vi "COD主界面（列队使用）.vi"() -> (8 "多列列表框":i32(listbox))   [LabVIEW 2016, in "斯坦道CODMn.lvlib"]
uses:
  <vilib>/Analysis/6fits.llb/Curve Fitting Criteria.ctl
  <vilib>/Utility/miscctls.llb/LVPointTypeDef.ctl
  <vilib>/Plasmionique/MB Master/MB_Master_Serial/MB_Master_Serial.lvclass
  D:/Program Files (x86)/National Instruments/LabVIEW 2016/vi.lib/Plasmionique/MB Master/MB_Master/MB_Master.lvclass
  <vilib>/Utility/config.llb/Write Key (Double).vi
  <vilib>/Utility/config.llb/Read Key (Double).vi
  <vilib>/Utility/config.llb/Read Key (Boolean).vi
  <vilib>/Utility/config.llb/Read Key (I32).vi
  <vilib>/Utility/config.llb/Write Key (Boolean).vi
  <vilib>/Utility/config.llb/Write Key (I32).vi
  <vilib>/Waveform/WDTFileIO.llb/Read Waveform from File.vi
  <vilib>/Plasmionique/MB Master/MB Master.lvlib
  <vilib>/ptbypt/NI_PtbyPt.lvlib
  <vilib>/Utility/config.llb/NI_LVConfig.lvlib
  <vilib>/Analysis/NI_AALPro.lvlib
panel:
  in  "一键写入":bool
  in  "测量模式(公式)":u16(ring)=1 items=["水样测试"=1, "标样核查"=2, "零点核查"=3, "跨度核查"=4, "空白测试"=5, "平行样"=6, "加标回收"=7]
  out "量程解释说明":string
  out "稀释倍数解释":string
  in  "低量程稀释倍数:":i8=1
  in  "高量程稀释倍数:":i8=2
  in  "测量模式":T1(ring)
  in  "高切低阈值":dbl
  in  "低切高阈值":dbl
  in  "数据查询":bool
  out "序列号:":string
  out "串口号:":refnum<visa-resource-name>
  in  "启用5":bool
  in  "校准5":bool
  in  "泵滴定数5":dbl
  in  "浓度5":dbl
  in  "启用4":bool
  in  "校准4":bool
  in  "泵滴定数4":dbl
  in  "浓度4":dbl
  out "波形时间":timestamp
  in  "历史波形":bool
  out "滴定数-ORP值":u16[](array[numeric]) caption="数组"
  in  "关闭 3":bool
  in  "滴定曲线":bool
  out "ORP滴定曲线2":u16[](graph)
  in  "跨度液浓度":dbl
  out "空白测试标记":bool
  out "跨度核查标记":bool
  out "启动选择 2":u16(ring) items=["水样测试", "标样核查", "零点核查", "跨度核查", "空白测试", "加标回收", "平行样", "校零", "校标"]
  in  "量程选择":enum16{"低量程", "高量程", "0-2量程"}(ring)
  in  "手动控制":bool
  in  "选用水样":enum16{"葡萄糖", "草酸钠"}(ring)
  in  "方程系数":cluster{"X":dbl, "b":dbl, "X^2":dbl} {"X^2" format="%#.4g"; "b" format="%#.4g"; "X" format="%#.4g"}
  out "多项式系数1":dbl[](array[numeric]) caption="多项式系数"
  out "XY图":cluster{"X Values":dbl[], "Y Values":dbl[]}[](graph)
  in  "模型":enum32{"线性", "多项式"}(ring)
  out "启动时间":timestamp format="%<%Y/%m/%d %H:%M:%S>T"
  in  "自动切换量程":bool=TRUE
  in  "24H周期设置":bool[](xcontrol)
  in  "关闭 2":bool
  in  "周期设置":bool
  out "r^2":dbl format="%.8g"
  out "拟合公式":string
  out "b":dbl format="%#.4g"
  out "K":dbl format="%#.4f"
  out "当前校准":i32
  in  "启用3":bool
  in  "启用2":bool
  in  "启用1":bool
  in  "校准3":bool
  in  "校准2":bool
  in  "校准1":bool
  in  "泵滴定数3":dbl
  in  "泵滴定数2":dbl
  in  "泵滴定数1":dbl
  in  "浓度3":dbl
  in  "浓度2":dbl
  in  "浓度1":dbl
  in  "写入":bool
  out "测量模式数字":i32
  out "零点核查标记":bool
  out "排液故障":bool
  out "进水样超量程":bool
  out "标样核查标记":bool
  out "平行样测量":bool
  out "加标回收测量":bool
  out "质控样测量":bool
  out "待机":bool
  out "校标错误":bool
  out "校零错误":bool
  out "测量错误":bool
  out "草酸钠报警":bool
  out "高锰酸钾报警":bool
  out "加热故障":bool
  out "温控器故障":bool
  out "ORP故障":bool
  out "排液标记":bool
  out "故障标记":bool
  out "校标标记":bool
  out "校零标记":bool
  out "通讯状态":bool
  out "水样测量":bool
  out "读取KB值":bool
  in  "读取":bool
  in  "返回":bool
  in  "校准配置":bool
  in  "修正系数 2":dbl
  in  "浓度 2":dbl
  in  "温度":dbl
  in  "恒温时间":dbl
  in  "基本量程":enum16{"L", "H"}(ring)
  in  "水样":dbl
  in  "蒸馏水":dbl
  in  "标液":dbl
  in  "质控样":dbl
  in  "加标回收":dbl
  in  "草酸钠":dbl
  in  "高锰酸钾":dbl
  in  "硫酸":dbl
  in  "零点泵计量数 2":dbl
  in  "标度泵计量数 2":dbl
  out "标度滴定值":dbl
  out "零点滴定值":dbl
  in  "保存":bool
  in  "关闭":bool
  out "测量数据区":T2 {"单位" items=["ug/L", "mg/L", "ppm", "mg/m3", "cm", "ppb", "ug/m3", "%", "nmol/mol", "umol/mol", "MPN/L", "MPN/100ml", "ng/m3", "NTU", "无量纲", "ms/cm", "us/cm", "℃", "mV", "万个/L"]}
  out "仪器时间":timestamp format="%<%Y/%m/%d %H:%M:%S>T"
  out "秒":u16
  out "分":u16
  out "COD浓度（mg/L)":dbl format="%.2g"
  out "进样管":dbl
  out "高锰酸钾":dbl
  out "草酸钠":dbl
  out "硫酸":dbl
  out "ORP显示":dbl
  out "温度":dbl
  out "加热":bool
  out "搅拌":bool
  out "进硫酸":bool
  out "进加标回收样":bool
  out "进质控样":bool
  out "进标液":bool
  out "进蒸馏水":bool
  out "进水样":bool
  out "进草酸钠":bool
  out "进高锰酸钾":bool
  out "定时启动":bool
  in  "启动":bool
  in  "故障清除":bool
  in  "参数配置":bool
  in  "停止":bool
  in  "单步启动":bool
  out "系统时间":timestamp
  in  "时间校准":bool
  in  "枚举":enum16{"读取数据", "写入数据", "读取写入DATABASE", "读取参数"}(ring)
  out "Registers":u16[](array[numeric])
  in  "Slave ID":u8=1
  in  "Serial Config":T3={"baud rate (bps)"=115200, "stop bits"=10, "parity"=0, "flow control"=0, "timeout"=1000, "retries"=1} {"stop bits" items=["1.0"=10, "1.5"=15, "2.0"=20]; "flow control" items=["None", "XON/XOFF", "RTS/CTS", "XON/XOFF & RTS/CTS", "DTR/DSR", "XON/XOFF & DTR/DSR"]; "parity" items=["None", "Odd", "Even", "Mark", "Space"]}
  in  "温度 2":dbl
  in  "浓度":dbl
  in  "修正系数":dbl
  in  "标样浓度 2":dbl
  out "模式（受控）":u16
  in  "VISA resource name":refnum<visa-resource-name>="COM4" caption="VISA资源名称"
  # "测量时间："
  # "水样~加标回收"
  # "mV"
  # "℃"
  # "注：遇到加热故障和排液故障时仪器不能正常启动，\n必须排查故障并点击报警清除按钮方可运行。"
  # "mg/L"
  # "基本参数设置"
  # "泵计量参数设置"
  # "校零校标结果"
  # "加热恒温温度（℃）："
  # "水样："
  # "高锰酸钾："
  # "校零结果："
  # "校零滴定值："
  # "恒温时间（分钟）："
  # "蒸馏水："
  # "草酸钠："
  # "校标结果："
  # "标度滴定值："
  # "标准液浓度（mg/L）："
  # "标液："
  # "硫酸："
  # "零点泵计量值："
  # "修正系数："
  # "标度泵计量值："
  # "质控样："
  # "跨度液浓度："
  # "标样浓度："
  # "基本量程（L、H可选）："
  # "加标回收样："
  # "（mg/L）"
  # "是否启用"
  # "泵滴定数"
  # "浓度"
  # "辅\n助\n计\n算\n区"
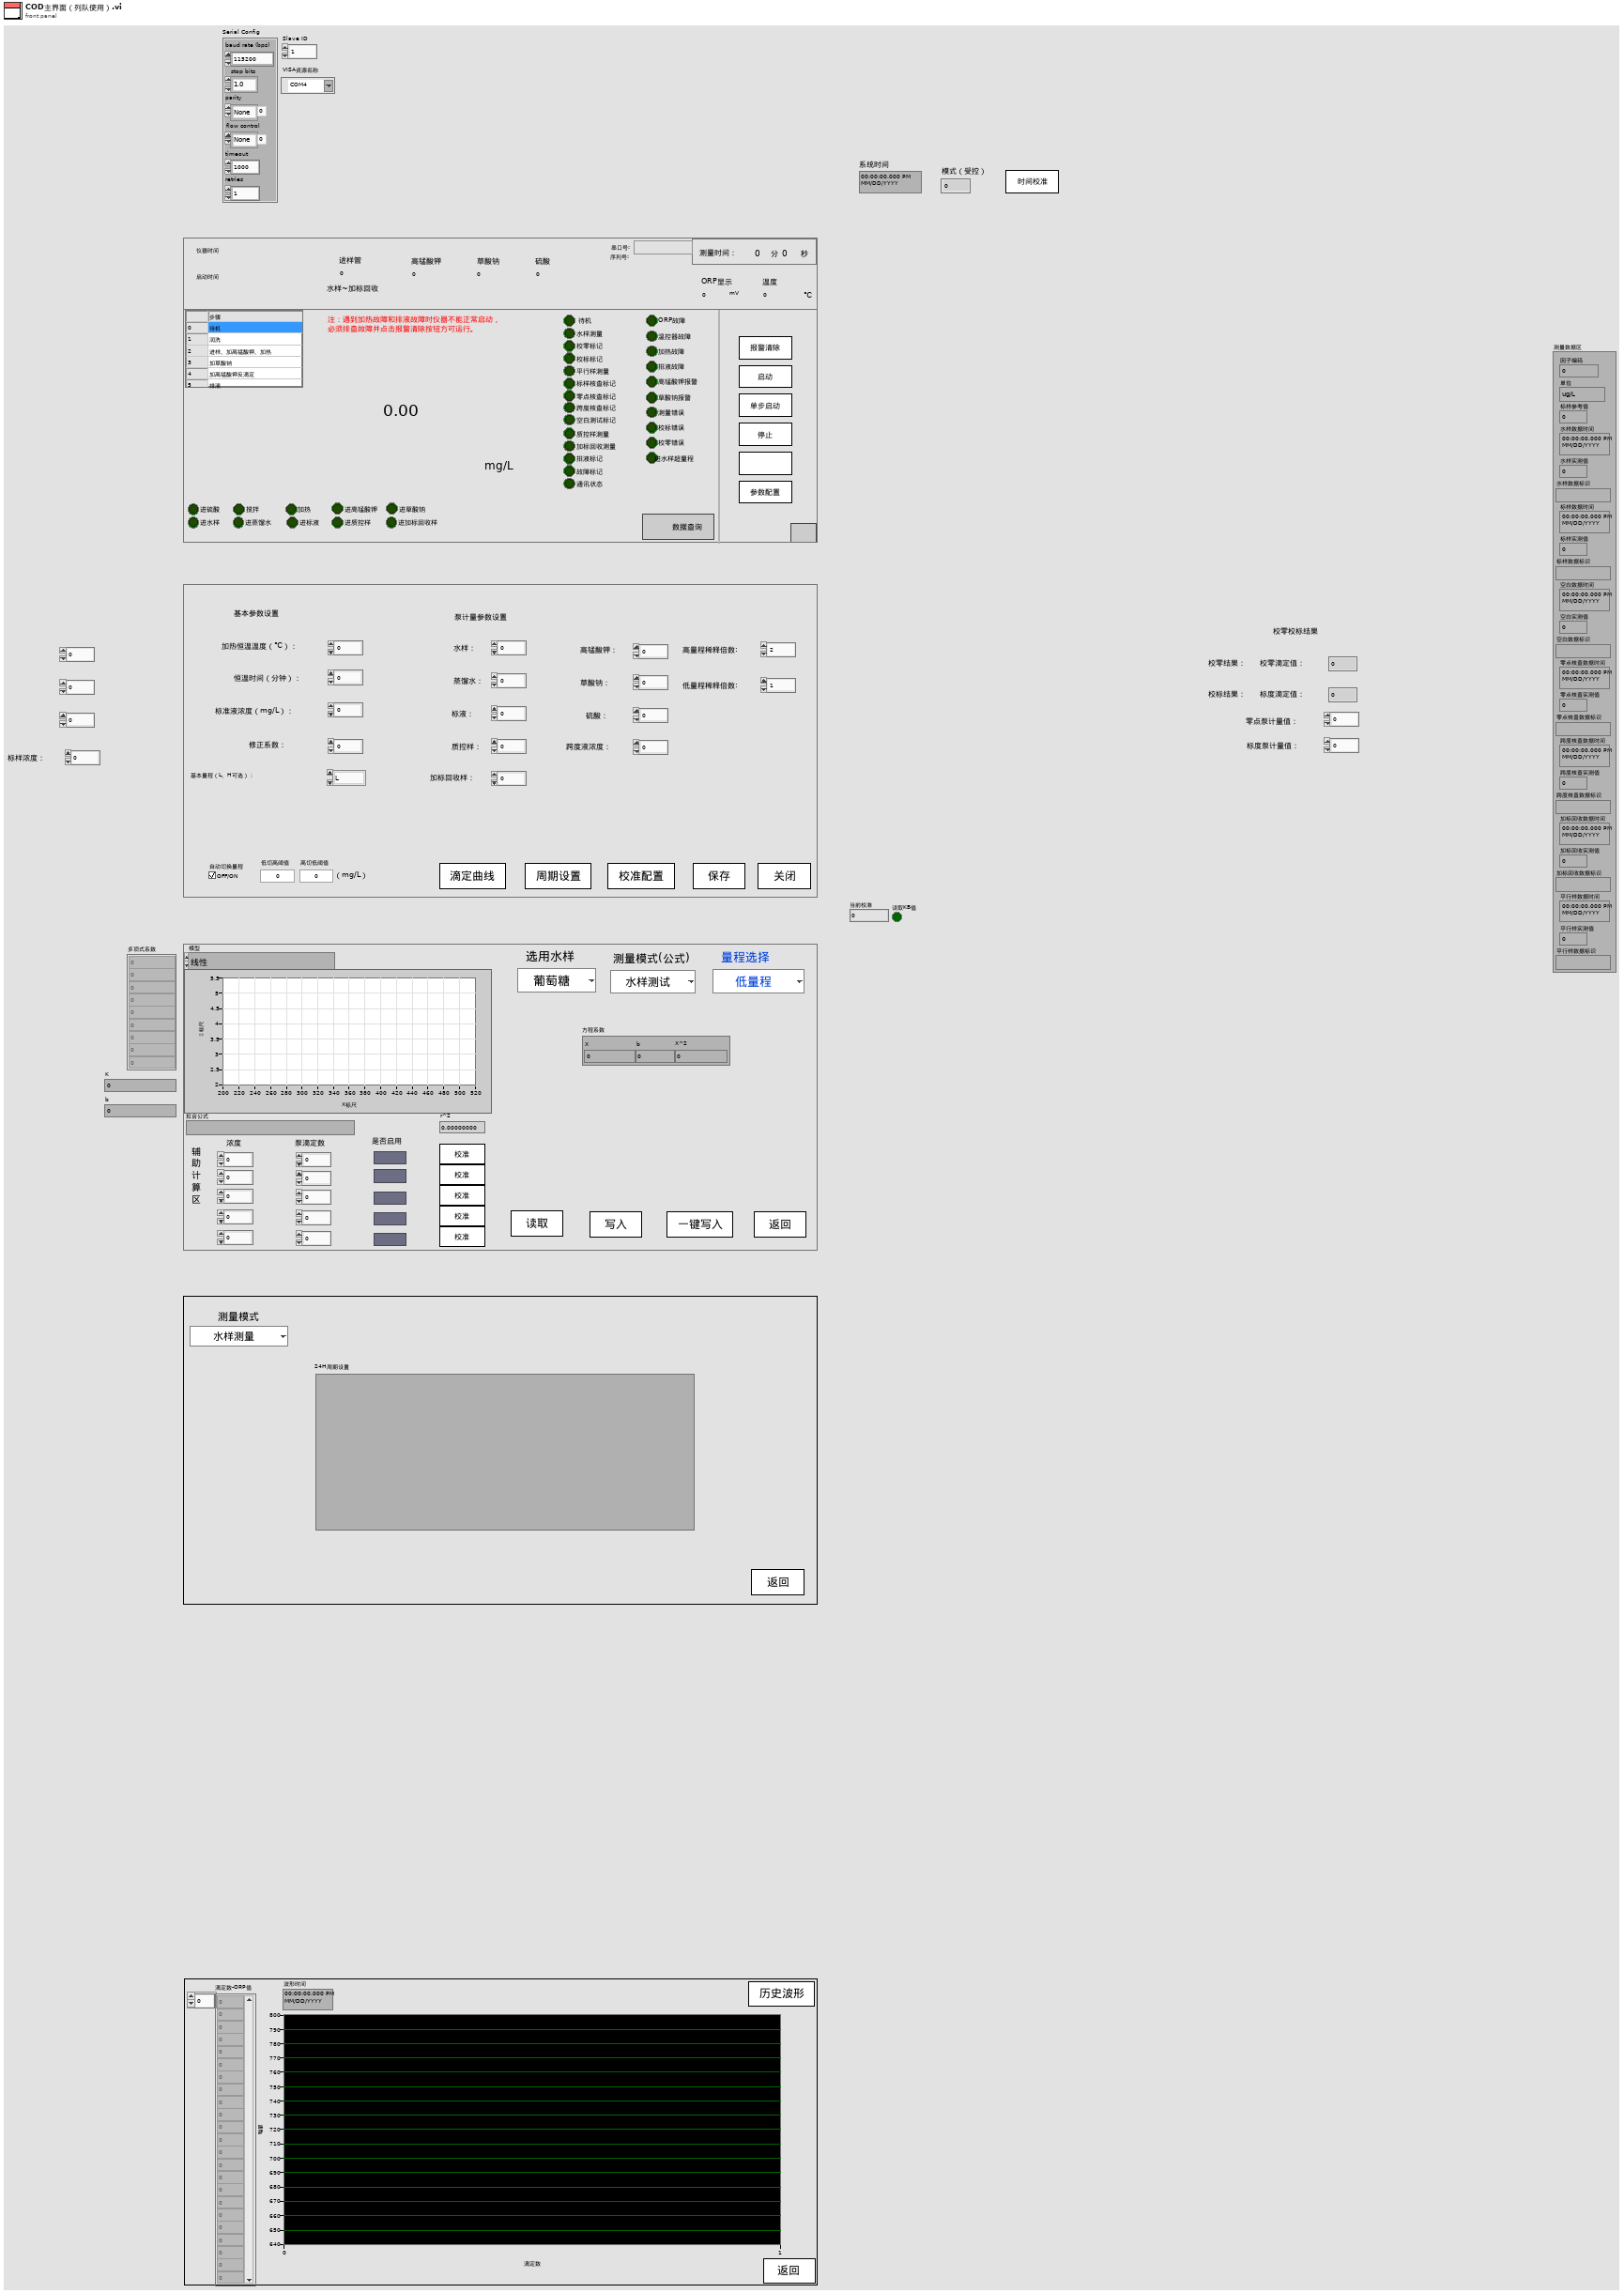
[diagram p1: front panel]
types:
  T1 = enum16{"水样测量", "标样核查", "零点核查", "跨度核查", "空白测试", "加标回收", "平行样", "校零", "校标"}
  T2 = cluster{"因子编码":u32, "单位":u16, "标样参考值":sgl, "水样数据时间":timestamp, "水样实测值":sgl, "水样数据标识":string, "标样数据时间":timestamp, "标样实测值":sgl, "标样数据标识":string, "空白数据时间":timestamp, "空白实测值":sgl, "空白数据标识":string, "零点核查数据时间":timestamp, "零点核查实测值":sgl, "零点核查数据标识":string, "跨度核查数据时间":timestamp, "跨度核查实测值":sgl, "跨度核查数据标识":string, "加标回收数据时间":timestamp, "加标回收实测值":sgl, "加标回收数据标识":string, "平行样数据时间":timestamp, "平行样实测值":sgl, "平行样数据标识":string}
  T3 = cluster{"baud rate (bps)":u32, "stop bits":u16, "parity":u16, "flow control":u16, "timeout":u32, "retries":i32}
  T4 = cluster{"starting address":u16, "number of holding registers":u16}
  T5 = cluster{"测量模式":enum16{"水样测量", "标样核查", "零点核查", "跨度核查", "空白测试", "加标回收", "平行样", "校零", "校标"}}
  T6 = cluster{"仪器测试类型":enum16{"水样测试", "标样核查", "空白测试", "跨度核查"}, "周期设置类型":enum16{"定点启动", "间隔启动"}, "定时功能启用":bool, "定时间隔":dbl, "24H周期设置":bool[]}
  T7 = typedef "LVDateTimeRec.ctl" = cluster{"秒数的小数部分":dbl, "秒":i32, "分":i32, "时":i32, "日":i32, "月":i32, "年":i32, "天数（周）":i32, "天数（年）":i32, "DST":i32}
  T8 = typedef "imagedata.ctl" = cluster{"image type":i32, "image depth":i32, "image":u8[], "mask":u8[], "colors":u32[], "Rectangle":cluster{"left":i16, "top":i16, "right":i16, "bottom":i16}}
  T9 = typedef "NI_LVConfig.lvlib/Config Data RefNum.ctl" = refnum<k1>
  T10 = typedef "LVPointTypeDef.ctl" = cluster{"Horizontal":i16, "Vertical":i16}
  T11 = enum8{"Enabled", "Disabled", "Disabled and Grayed Out"}
  T12 = cluster{"ORP故障":bool, "温控器故障":bool, "加热故障":bool, "高锰酸钾报警":bool, "草酸钠报警":bool, "测量错误":bool, "校零错误":bool, "校标错误":bool, " 进水样超量程":bool, "排液阀故障":bool}
  T13 = cluster{"时间标识":timestamp, "参数":string, "日志信息":string, "流程参数":string}
  T14 = cluster{"时间标识":timestamp, "设备":string, "日志信息":string}
  T15 = typedef "NI_AALPro.lvlib/Curve Fitting Criteria.ctl" = u16
  T16 = cluster{"时间标识":timestamp, "设备":string, "日志信息":string, "流程参数":string}
  T17 = cluster{"时间":timestamp, "测量模式":string, "数据类型":string, "检测值":sgl, "单位":string, "数据标识":string, "因子编码":string, "标样参考值":sgl, "ORP-A":sgl, "ORP-B":sgl, "ORP-K":sgl, "COD滴定值":sgl, "高锰酸钾滴定数":sgl, "温度":sgl, "序列号":string}
  T18 = cluster{"数组 2[0]":sgl, "数组 2[1]":sgl, "数组 2[2]":sgl, "数组 2[3]":sgl, "数组 2[4]":sgl, "数组 2[5]":sgl, "数组 2[6]":sgl, "数组 2[7]":sgl, "数组 2[8]":sgl, "数组 2[9]":sgl, "数组 2[10]":sgl, "数组 2[11]":sgl, "数组 2[12]":sgl, "数组 2[13]":sgl, "数组 2[14]":sgl, "数组 2[15]":sgl, "数组 2[16]":sgl, "数组 2[17]":sgl, "数组 2[18]":sgl, "数组 2[19]":sgl, "数组 2[20]":sgl, "数组 2[21]":sgl, "数组 2[22]":sgl, "数组 2[23]":sgl, "数组 2[24]":sgl, "数组 2[25]":sgl, "数组 2[26]":sgl, "数组 2[27]":sgl, "数组 2[28]":sgl, "数组 2[29]":sgl, "数组 2[30]":sgl, "数组 2[31]":sgl, "数组 2[32]":sgl, "数组 2[33]":sgl, "数组 2[34]":sgl, "数组 2[35]":sgl, "数组 2[36]":sgl, "数组 2[37]":sgl, "数组 2[38]":sgl, "数组 2[39]":sgl, "数组 2[40]":sgl, "数组 2[41]":sgl}
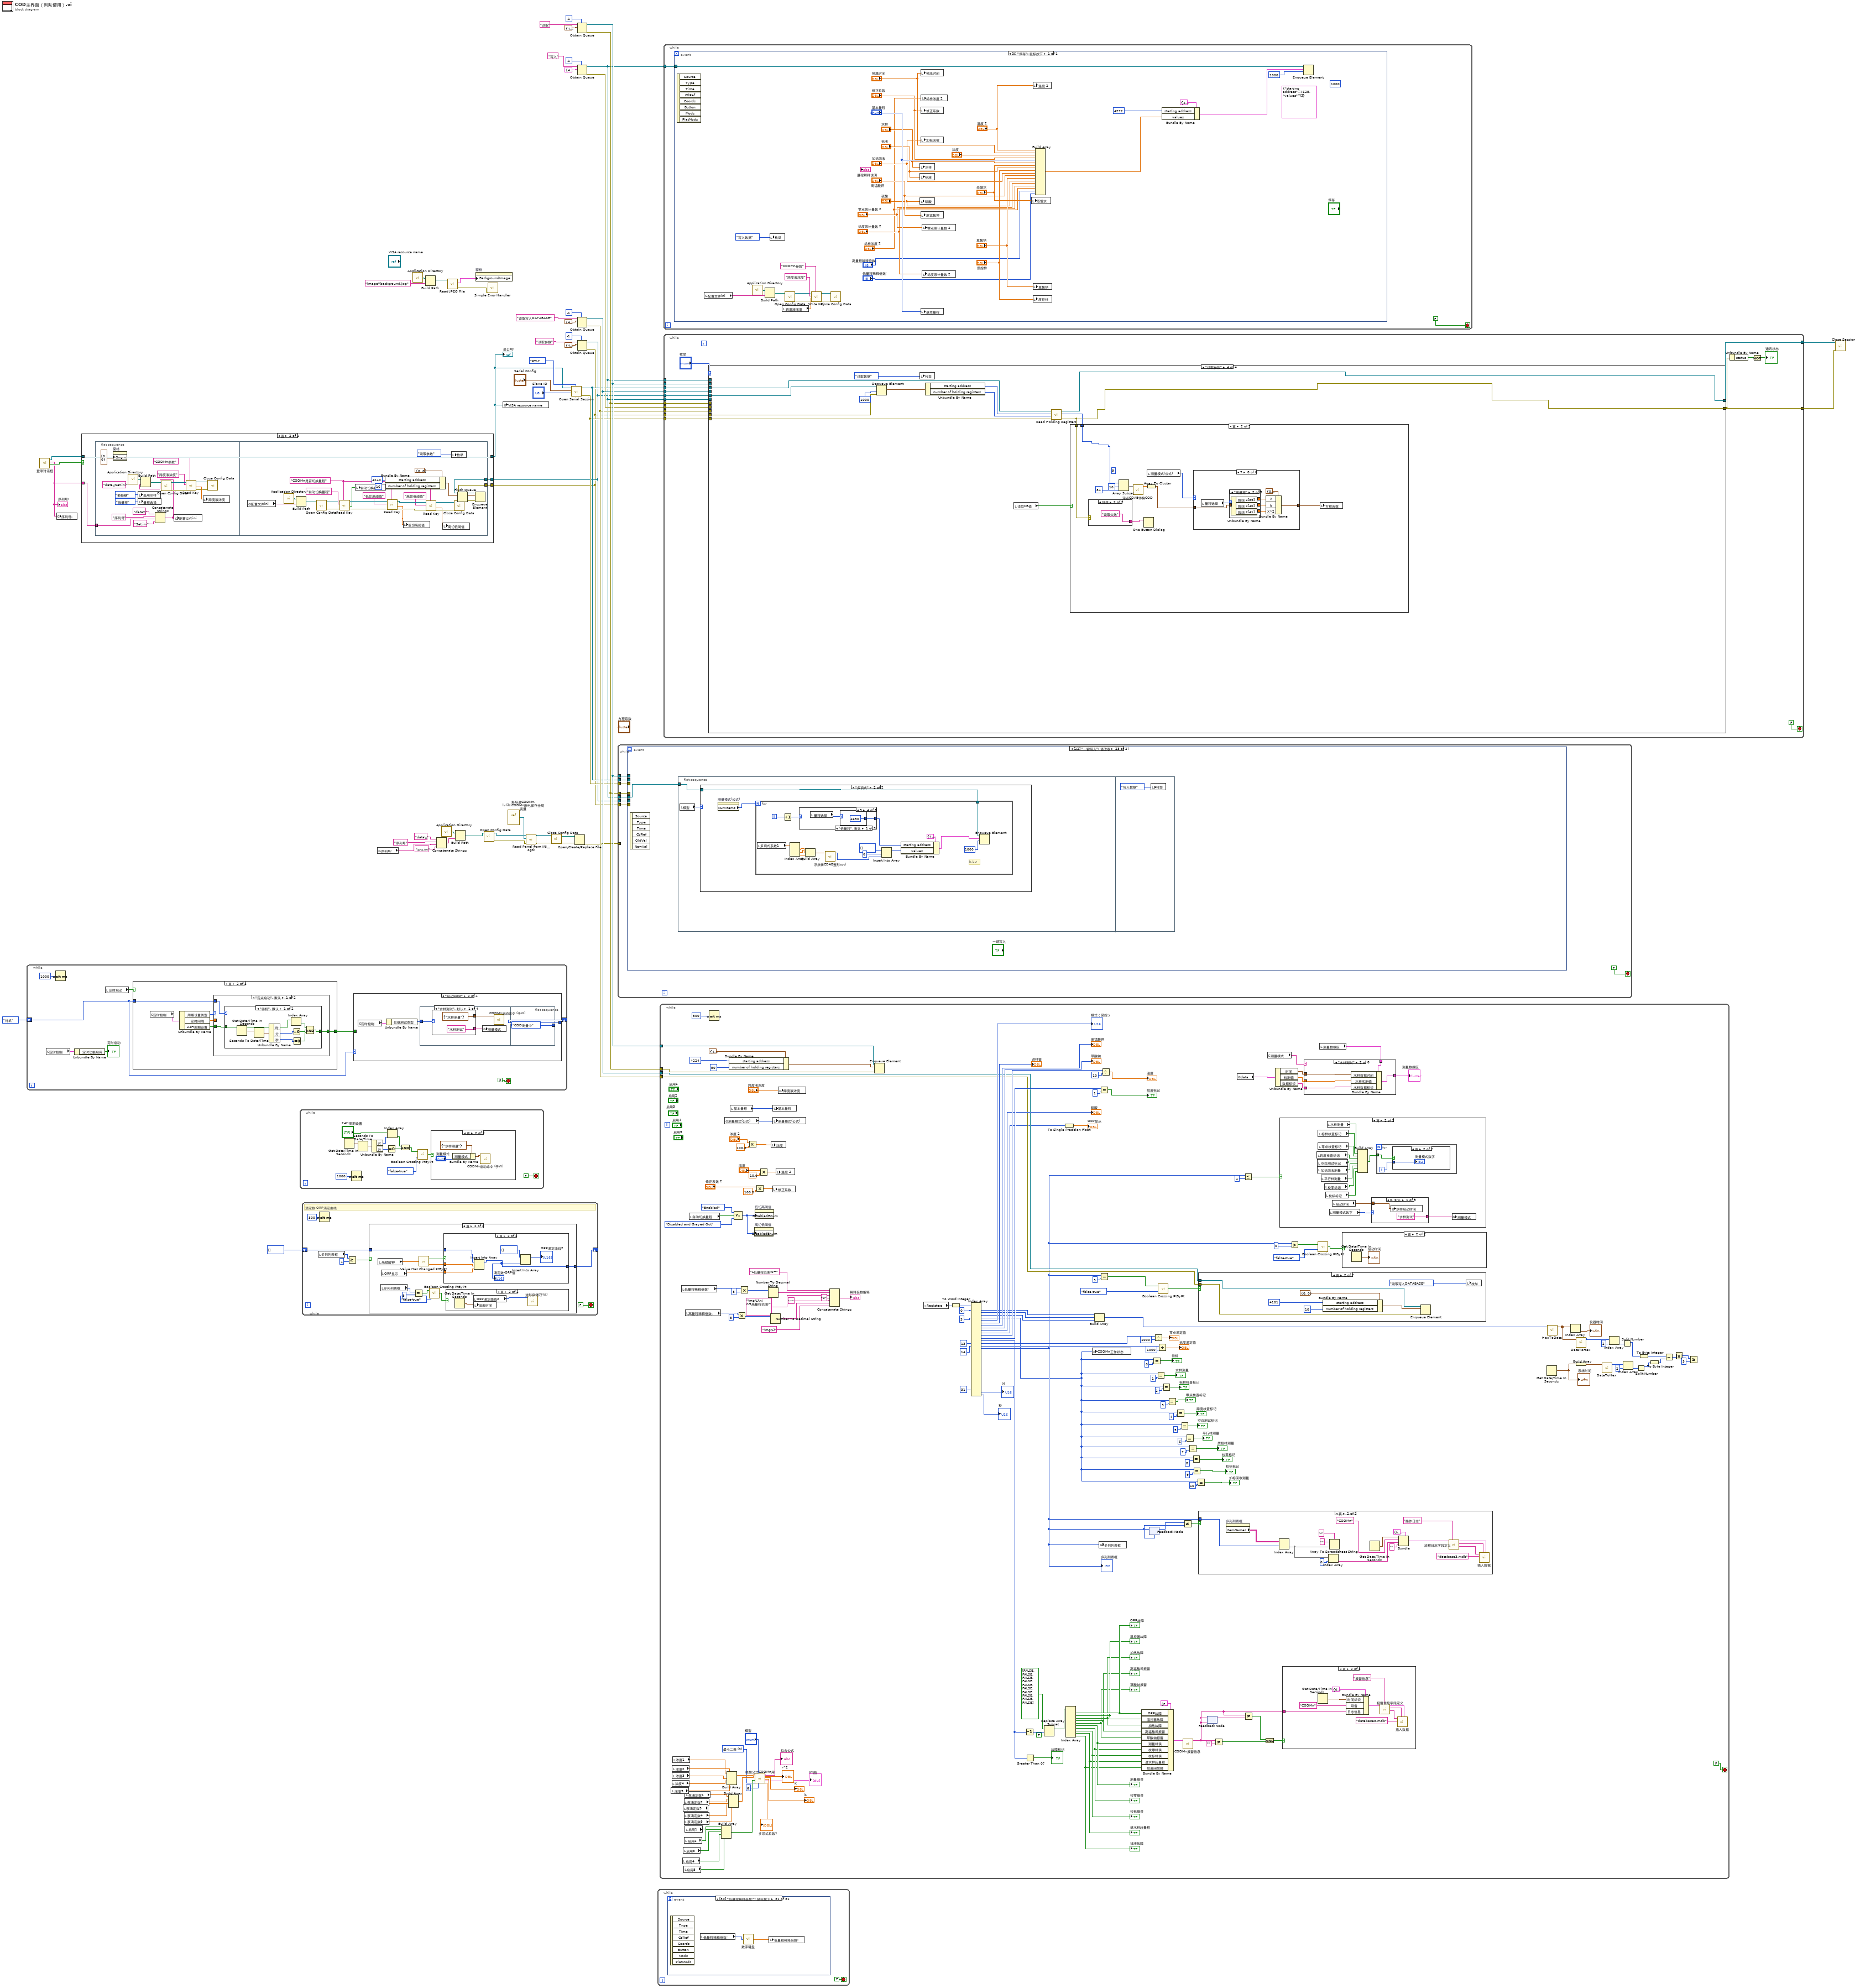
[diagram p0: block diagram]
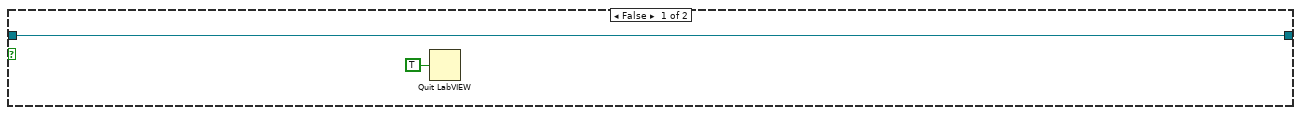
[diagram p2: hidden frame]
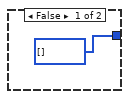
[diagram p3: hidden frame]
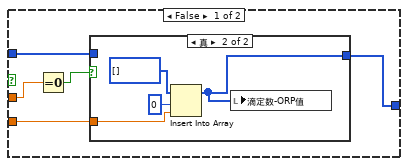
[diagram p5: hidden frame]
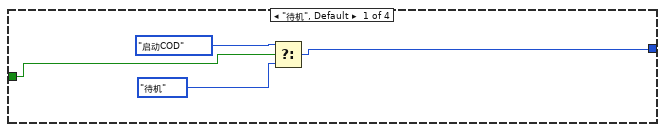
[diagram p8: hidden frame]
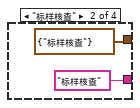
[diagram p9: hidden frame]
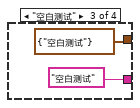
[diagram p10: hidden frame]
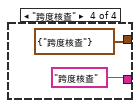
[diagram p11: hidden frame]
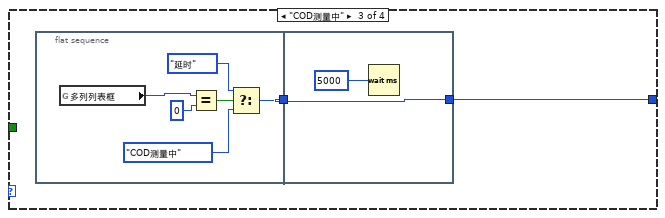
[diagram p12: hidden frame]
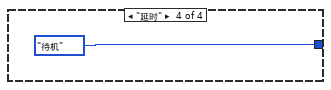
[diagram p13: hidden frame]
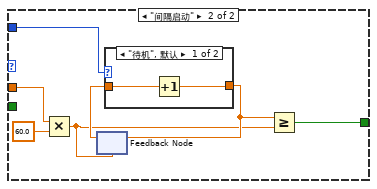
[diagram p16: hidden frame]
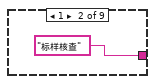
[diagram p20: hidden frame]
diagram:
  n1 = while {
    shift-right: [w54] -> _
    shift-left: enum16{"待机", "启动COD", "COD测量中", "延时"}."待机" -> [w56]
    stop <- FALSE stop-if-true
    n2 = global read "CODMn断电保存全局变量.vi" "定时控制"() -> (w58:T6)
    n3 = Wait (ms)(milliseconds to wait=u32 1000 ("等待时间（毫秒）")) -> ()  [unwired: 1 out]
    n4 = Unbundle By Name(w58) -> ("定时功能启用"=→"定时启动":bool)
    n5 = local read "定时启动"() -> (w60:bool)
    n6 = case shown="真" w60 {
      tunnel: w56 -> [_ w95]
      tunnel: [_ w94] -> w55
      frame False {
      }
      frame True {
        n7 = global read "CODMn断电保存全局变量.vi" "定时控制"() -> (w97:T6)
        n8 = Unbundle By Name(w97) -> ("周期设置类型"=w96:enum16{"定点启动", "间隔启动"}, "定时间隔"=w92:dbl, "24H周期设置"=w93:bool[])
        n9 = case shown="\"定点启动\", 默认" w96 {
          tunnel: w95 -> [w100 w116]
          tunnel: w93 -> [w99 _]
          tunnel: [w98 w111] -> w94
          tunnel: w92 -> [_ w110]
          frame "定点启动", Default {
            n10 = case shown="\"待机\", 默认" w100 {
              tunnel: w99 -> [w107 _]
              tunnel: [w101 _] -> w98
              frame "待机", Default {
                n11 = Get Date/Time In Seconds() -> (seconds since 1Jan1904=w109:timestamp)
                n12 = Seconds To Date/Time(time stamp (now)=w109) -> (date time rec=w108:T7)  [unwired: 1 in]
                n13 = Unbundle By Name(w108) -> ("分"=w105:i32, "秒"=w104:i32)  [unwired: 1 out]
                n14 = Index Array(array=w107) -> (element=w106:bool)  [unwired: 1 in]
                n15 = Equal To 0?(x=w105) -> (x = 0?=w103:bool)
                n16 = Equal To 0?(x=w104) -> (x = 0?=w102:bool)
                n17 = Compound Arithmetic op=AND ("复合运算")(w106, w103, w102) -> (w101:bool)
              }
              frame "启动COD" {
              }
            }
          }
          frame "间隔启动" {
            n18 = Multiply(x=w110, y=60.0) -> (x*y=w112:dbl)
            n19 = feedback #1(w112) -> (w115:dbl)
            n20 = case shown="\"待机\", 默认" w116 {
              tunnel: w115 -> [w118 _]
              tunnel: [w117 _] -> w113
              frame "待机", Default {
                n21 = Increment(x=w118) -> (x+1=w117:dbl)
              }
              frame "启动COD" {
              }
            }
            n22 = feedback-in #1(w113) -> ()
            n23 = Greater Or Equal?(x=w113, y=w112) -> (x >= y?=w111:bool)
          }
        }
      }
    }
    n24 = case shown="\"启动COD\"" w56 {
      tunnel: [w62 w68 w82 enum16{"待机", "启动COD", "COD测量中", "延时"}."待机"] -> w54
      tunnel: w55 -> [w63 _ _ _]
      frame "待机", Default {
        n25 = Select(t=enum16{"待机", "启动COD", "COD测量中", "延时"}."启动COD", s=w63, f=enum16{"待机", "启动COD", "COD测量中", "延时"}."待机") -> (s? t:f=w62:enum16{"待机", "启动COD", "COD测量中", "延时"})
      }
      frame "启动COD" {
        n26 = global read "CODMn断电保存全局变量.vi" "定时控制"() -> (w67:T6)
        n27 = Unbundle By Name(w67) -> ("仪器测试类型"=w66:enum16{"水样测试", "标样核查", "空白测试", "跨度核查"})
        n28 = flat-sequence {
          tunnel: w66 -> [w69]
          tunnel: [enum16{"待机", "启动COD", "COD测量中", "延时"}."COD测量中"] -> w68
          frame #0 {
            n29 = case shown="\"水样测试\", 默认" w69 {
              tunnel: ["水样测试" ("测量模式") "标样核查" ("测量模式") "空白测试" ("测量模式") "跨度核查" ("测量模式")] -> w71
              tunnel: [T5 {"测量模式"=enum."水样测量"} ("启动测量模式") T5 {"测量模式"=enum."标样核查"} ("启动测量模式") T5 {"测量模式"=enum."空白测试"} ("启动测量模式") T5 {"测量模式"=enum."跨度核查"} ("启动测量模式")] -> w70
              frame "水样测试", Default {
              }
              frame "标样核查" {
              }
              frame "空白测试" {
              }
              frame "跨度核查" {
              }
            }
            n30 = global write "COD测量模式全局.vi" "测量模式"(w71) -> ()
            n31 = call "CODMn启动命令 (子VI).vi"("启动测量模式"=w70) -> ()  [unwired: 11 in]
          }
          frame #1 {
          }
        }
      }
      frame "COD测量中" {
        n32 = flat-sequence {
          tunnel: [w83] -> w81
          tunnel: [w90] -> w82
          tunnel: w81 -> [w90]
          frame #0 {
            n33 = global read "运行时序全局变量.vi" "多列列表框"() -> (w88:i32)
            n34 = Equal?(x=w88, y=0) -> (x = y?=w86:bool)
            n35 = Select(t=enum16{"待机", "启动COD", "COD测量中", "延时"}."延时", s=w86, f=enum16{"待机", "启动COD", "COD测量中", "延时"}."COD测量中") -> (s? t:f=w83:enum16{"待机", "启动COD", "COD测量中", "延时"})
          }
          frame #1 {
            n36 = Wait (ms)(milliseconds to wait=u32 5000 ("等待时间（毫秒）")) -> ()  [unwired: 1 out]
          }
        }
      }
      frame "延时" {
      }
    }
  }
  n37 = call "登录对话框.vi"() -> ("输出"=w25:bool, "序列号"=w23:string, "串口号"=w26:refnum<visa-resource-name>)  [unwired: 7 in]
  "序列号:" <- w23
  n38 = global write "COD浓度全局变量.vi" "序列号:"(w23) -> ()
  n39 = while {
    stop <- FALSE stop-if-true
    n40 = Get Date/Time In Seconds() -> (seconds since 1Jan1904=w130:timestamp)
    n41 = Wait (ms)(milliseconds to wait=u32 1000 ("等待时间（毫秒）")) -> ()  [unwired: 1 out]
    n42 = Seconds To Date/Time(time stamp (now)=w130) -> (date time rec=w129:T7)  [unwired: 1 in]
    n43 = Unbundle By Name(w129) -> ("时"=w126:i32, "分"=w128:i32)
    n44 = Equal To 0?(x=w128) -> (x = 0?=w127:bool)
    n45 = Index Array(array="24H周期设置", index=w126) -> (element=w125:bool)
    n46 = And(x=w125, y=w127) -> (x .and. y?=w123:bool)
    n47 = call <vilib>:"Boolean Crossing PtByPt.vi"("direction"=enum16{"either", "false-true", "true-false"}."false-true", "input"=w123) -> ("crossing"=w122:bool)  [unwired: 1 in]
    n48 = case shown="真" w122 {
      frame False {
      }
      frame True {
        n49 = Bundle By Name(cluster=T5 {"测量模式"=enum."水样测量"} ("启动测量模式"), "测量模式"="测量模式") -> (w132:T5)
        n50 = call "CODMn启动命令 (子VI).vi"("启动测量模式"=w132) -> ()  [unwired: 11 in]
      }
    }
  }
  n51 = while {
    shift-right: [w137] -> _
    shift-left: u16[] [] ("ORP滴定曲线") -> [w138]
    stop <- FALSE stop-if-true
    # "滴定数-ORP滴定曲线"
    n52 = local read "多列列表框"() -> (w136:i32)
    n53 = Wait (ms)(milliseconds to wait=u32 300 ("等待时间（毫秒）")) -> ()  [unwired: 1 out]
    n54 = Greater Or Equal?(x=w136, y=4) -> (x >= y?=w134:bool)
    n55 = case shown="真" w134 {
      tunnel: w138 -> [_ w152]
      tunnel: [u16[] [] ("ORP滴定曲线") w151] -> w137
      frame False {
      }
      frame True {
        n56 = local read "高锰酸钾"() -> (w148:dbl)
        n57 = local read "多列列表框"() -> (w146:i32)
        n58 = local read "ORP显示"() -> (w147:dbl)
        n59 = Equal?(x=w146, y=5) -> (x = y?=w144:bool)
        n60 = call <vilib>:"Value Has Changed PtByPt.vi"("input data point"=w148) -> ("has changed"=w150:bool, "output data point"=w149:dbl)  [unwired: 1 in]
        n61 = call <vilib>:"Boolean Crossing PtByPt.vi"("direction"=enum16{"either", "false-true", "true-false"}."false-true", "input"=w144) -> ("crossing"=w142:bool)  [unwired: 1 in]
        n62 = case shown="真" w150 {
          tunnel: w152 -> [w158 w168]
          tunnel: [w157 w167] -> w151
          tunnel: w149 -> [w159 w166]
          tunnel: w147 -> [w155 w165]
          frame False {
            n63 = Equal To 0?(x=w159) -> (x = 0?=w156:bool)
            n64 = case shown="真" w156 {
              tunnel: [w160 w163] -> w157
              tunnel: w158 -> [w160 _]
              tunnel: w155 -> [_ w162]
              frame False {
              }
              frame True {
                n65 = Insert Into Array(array=u16[] [] ("ORP滴定曲线"), index=0 ("索引"), new element=w162) -> (w163:u16[])
                n66 = local write "滴定数-ORP值"(w163) -> ()
              }
            }
          }
          frame True {
            n67 = Insert Into Array(array=w168, index=w166, new element=w165) -> (w167:u16[])
            "滴定数-ORP值" <- w167
            n68 = Insert Into Array(array=u16[] [] ("ORP滴定曲线"), new element=w167) -> (→"ORP滴定曲线2":u16[])  [unwired: 1 in]
          }
        }
        n69 = case shown="真" w142 {
          frame False {
          }
          frame True {
            n70 = Get Date/Time In Seconds() -> (seconds since 1Jan1904=w153:timestamp)
            n71 = local read "ORP滴定曲线2"() -> (w154:u16[])
            n72 = local write "波形时间"(w153) -> ()
            n73 = call "波形存储(子VI).vi"("ORP滴定曲线"=w154) -> ()  [unwired: 11 in]
          }
        }
      }
    }
  }
  n74 = global read "COD浓度全局变量.vi" "序列号:"() -> (w11:string)
  n75 = call <vilib>:"Application Directory.vi"() -> ("Application Directory"=w22:path)
  n76 = Build Path(base path=w22, name or relative path="image\\background.jpg" ("名称或相对路径")) -> (appended path=w20:path)
  n77 = Concatenate Strings("data\\" ("字符串"), "序列号" ("字符串"), w11, "sys.ini" ("名称或相对路径")) -> (w12:string)
  n78 = call <vilib>:"Application Directory.vi"() -> ("Application Directory"=w7:path)
  n79 = call <vilib>:"Read JPEG File.vi"("path to JPEG file"=w20) -> ("error out"=w18:errorcluster, "image data"=w19:T8)  [unwired: 8 in, 1 out]
  n80 = Build Path(base path=w7, name or relative path=w12) -> (appended path=w13:path)
  n81 = property on="窗格" class="Pane"("BackgroundImage"=w19) -> ()  [unwired: 2 in, 2 out]
  n82 = call <vilib>:"Open Config Data.vi"("configuration file path"=w13) -> ("error out"=w4:errorcluster, "refnum"=w6:T9)  [unwired: 8 in, 1 out]
  n83 = call <vilib>:"Simple Error Handler.vi"("error in (no error)"=w18) -> ()  [unwired: 4 in, 5 out]
  n84 = vi-ref "斯坦道CODMn.lvlib:CODMn断电保存全局变量.vi"() -> (w5:refnum<vi>)
  n85 = call <userlib>:"Read Panel from INI__ogtk.vi"("error in (no error)"=w4, "VI ref"=w5, "refnum"=w6) -> ("error out"=w2:errorcluster, "refnum out"=w3:T9)  [unwired: 7 in]
  n86 = call <vilib>:"Close Config Data.vi"("error in (no error)"=w2, "refnum"=w3) -> ("error out"=w15:errorcluster, "file path"=w14:path)  [unwired: 8 in]
  n87 = Open/Create/Replace File(file path (use dialog)=w14, error in=w15) -> (error out=w1:errorcluster)  [unwired: 4 in, 2 out]
  n88 = Obtain Queue(max queue size (-1, unlimited)=-1 ("队列最大值（-1，无限）"), name (unnamed)="读取" ("名称（未命名）"), element data type=T4 {"starting address"=4224, "number of holding registers"=16}) -> (queue out=w44:refnum<queue>, error out=w43:errorcluster)  [unwired: 2 in, 1 out]
  n89 = Obtain Queue(max queue size (-1, unlimited)=-1 ("队列最大值（-1，无限）"), name (unnamed)="写入" ("名称（未命名）"), element data type=cluster{"starting address":u16, "values":u16[]} {"starting address"=4272, "values"=[]}) -> (queue out=w28:refnum<queue>, error out=w32:errorcluster)  [unwired: 2 in, 1 out]
  n90 = Obtain Queue(max queue size (-1, unlimited)=-1 ("队列最大值（-1，无限）"), name (unnamed)="读取写入DATABASE" ("名称（未命名）"), element data type=T4 {"starting address"=4224, "number of holding registers"=16}) -> (queue out=w34:refnum<queue>, error out=w33:errorcluster)  [unwired: 2 in, 1 out]
  n91 = Obtain Queue(max queue size (-1, unlimited)=-1 ("队列最大值（-1，无限）"), name (unnamed)="读取参数" ("名称（未命名）"), element data type=T4 {"starting address"=4224, "number of holding registers"=16}) -> (queue out=w17:refnum<queue>, error out=w16:errorcluster)  [unwired: 2 in, 1 out]
  n92 = case shown="真" w25 {
    tunnel: w26 -> [w171 w176]
    tunnel: [w171 w176] -> w24
    tunnel: w23 -> [_ w175]
    tunnel: w17 -> [_ w174]
    tunnel: w16 -> [_ w173]
    frame False {
      n93 = Quit LabVIEW(quit? (T)=TRUE ("退出？(T)")) -> ()
    }
    frame True {
      n94 = flat-sequence {
        tunnel: w175 -> [w179]
        tunnel: w174 -> [w213]
        tunnel: w173 -> [w212]
        frame #0 {
          (unwired) "data\\Set.ini" ("名称或相对路径")
          n95 = property on="窗格" class="Pane"("Origin"=T10 {"Horizontal"=0, "Vertical"=0} ("原点")) -> ()  [unwired: 2 in, 2 out]
          n96 = call <vilib>:"Application Directory.vi"() -> ("Application Directory"=w184:path)
          n97 = local write "选用水样"(enum16{"葡萄糖", "草酸钠"}."葡萄糖" ("选用水样")) -> ()
          n98 = local write "量程选择"(enum16{"低量程", "高量程", "0-2量程"}."低量程" ("量程选择")) -> ()
          n99 = Concatenate Strings("data\\" ("字符串"), "序列号" ("字符串"), w179, "Set.ini" ("名称或相对路径")) -> (w178:string)
          n100 = Build Path(base path=w184, name or relative path=w178) -> (appended path=w185:path)
          n101 = call <vilib>:"Open Config Data.vi"("configuration file path"=w185) -> ("error out"=w189:errorcluster, "refnum"=w188:T9)  [unwired: 8 in, 1 out]
          n102 = global write "COD浓度全局变量.vi" "配置文件ini"(w178) -> ()
          n103 = call-poly <vilib>:"Read Key.vi"("section"="CODMn参数" ("key"), "error in (no error)"=w189, "key"="跨度液浓度", "refnum"=w188) -> ("error out"=w191:errorcluster, "value"=w192:dbl, "refnum out"=w190:T9)  [unwired: 4 in, 1 out]
          n104 = local write "跨度液浓度"(w192) -> ()
          n105 = call <vilib>:"Close Config Data.vi"("error in (no error)"=w191, "refnum"=w190) -> ()  [unwired: 8 in, 2 out]
        }
        frame #1 {
          w208 = "CODMn是否切换量程" ("key")
          n106 = global read "COD浓度全局变量.vi" "配置文件ini"() -> (w200:string)
          n107 = call <vilib>:"Application Directory.vi"() -> ("Application Directory"=w196:path)
          n108 = Build Path(base path=w196, name or relative path=w200) -> (appended path=w197:path)
          n109 = call <vilib>:"Open Config Data.vi"("configuration file path"=w197) -> ("error out"=w195:errorcluster, "refnum"=w194:T9)  [unwired: 8 in, 1 out]
          n110 = call-poly <vilib>:"Read Key.vi"("section"=w208, "error in (no error)"=w195, "key"="自动切换量程", "refnum"=w194) -> ("error out"=w204:errorcluster, "value"=w199:bool, "refnum out"=w203:T9)  [unwired: 4 in, 1 out]
          n111 = local write "自动切换量程"(w199) -> ()
          n112 = Bundle By Name(cluster=T4 {"starting address"=0, "number of holding registers"=0}, "starting address"=u16 4240, "number of holding registers"=u16 16) -> (w220:T4)
          n113 = call-poly <vilib>:"Read Key.vi"("section"=w208, "error in (no error)"=w204, "key"="低切高阈值", "refnum"=w203) -> ("error out"=w207:errorcluster, "value"=w205:dbl, "refnum out"=w206:T9)  [unwired: 4 in, 1 out]
          n114 = local write "低切高阈值"(w205) -> ()
          n115 = call-poly <vilib>:"Read Key.vi"("section"=w208, "error in (no error)"=w207, "key"="高切低阈值", "refnum"=w206) -> ("error out"=w211:errorcluster, "value"=w209:dbl, "refnum out"=w210:T9)  [unwired: 4 in, 1 out]
          n116 = local write "高切低阈值"(w209) -> ()
          n117 = local write "枚举"(enum16{"读取数据", "写入数据", "读取写入DATABASE", "读取参数"}."读取参数" ("枚举")) -> ()
          n118 = call <vilib>:"Close Config Data.vi"("error in (no error)"=w211, "refnum"=w210) -> ()  [unwired: 8 in, 2 out]
          n119 = Flush Queue(queue=w213, error in (no error)=w212) -> (queue out=w216:refnum<queue>, error out=w215:errorcluster)  [unwired: 1 out]
          n120 = Enqueue Element(queue=w216, element=w220, error in (no error)=w215) -> ()  [unwired: 1 in, 3 out]
        }
      }
    }
  }
  "串口号:" <- w24
  n121 = global write "COD浓度全局变量.vi" "VISA resource name"(w24) -> ()
  n122 = call <vilib>:"Open Serial Session.vi"("Mode (RTU)"=enum16{"RTU", "ASCII"}."RTU", "Slave ID"="Slave ID", "Serial Config"="Serial Config", "VISA Resource"=w24) -> ("Error out"=w30:errorcluster, "MB_Serial session"=w31:refnum<class "MB_Master_Serial.lvclass">)  [unwired: 6 in]
  n123 = while {
    tunnel: w44 -> [w228]
    tunnel: w43 -> [w227]
    tunnel: w28 -> [w226]
    tunnel: w17 -> [w225]
    tunnel: w16 -> [w224]
    tunnel: w31 -> [w222]
    tunnel: w30 -> [w221]
    tunnel: w1 -> [_]
    stop <- FALSE stop-if-true
    n124 = event shown="[22] \"一键写入\": 值改变" {
      selector: _ -> [_ _ _ _ _ _ _ _ _ _ _ _ _ _ _ _ _ _ _ _ _ _ _ _ _ _ _]
      dyn-events: _ -> [_ _ _ _ _ _ _ _ _ _ _ _ _ _ _ _ _ _ _ _ _ _ _ _ _ _ _]
      timeout: _ -> [_ _ _ _ _ _ _ _ _ _ _ _ _ _ _ _ _ _ _ _ _ _ _ _ _ _ _]
      tunnel: w228 -> [_ _ _ _ _ _ _ _ _ _ _ _ _ _ _ _ _ _ _ _ _ _ _ _ _ _ _]
      tunnel: w227 -> [_ _ _ _ _ _ _ _ _ _ _ _ _ _ _ _ _ _ _ _ _ _ _ _ _ _ _]
      tunnel: w226 -> [w236 w269 w306 _ _ _ _ _ _ _ _ _ _ w690 w704 _ w730 _ _ _ _ w917 w1017 _ _ _ _]
      tunnel: w225 -> [_ _ _ _ w339 _ _ _ _ _ _ _ _ _ _ _ _ _ _ _ w909 _ _ _ _ _ _]
      tunnel: w224 -> [_ _ _ _ w338 _ _ _ _ _ _ _ _ _ _ _ _ _ _ _ w908 _ _ _ _ _ _]
      tunnel: w222 -> [_ _ _ w312 _ _ _ _ _ _ _ _ w689 _ _ _ _ _ _ _ _ _ _ _ _ _ _]
      tunnel: w221 -> [_ _ _ w311 _ _ _ _ _ _ _ _ w688 _ _ _ _ _ _ _ _ _ _ _ _ _ _]
      event "单步启动": Mouse Down {
        n125 = event-data() -> ()  [unwired: 1 in, 8 out]
        n126 = call "单步启动选择对话框.vi"() -> ("启动选择2"=w229:u16)  [unwired: 10 in, 1 out]
        n127 = case shown="3" w229 {
          tunnel: [u16 4610 ("address") u16 4610 ("address") u16 4610 ("address") u16 4610 ("address") u16 4610 ("address") u16 4610 ("address") u16 4610 ("address") u16 4610 ("address") u16 4610 ("address") u16 4610 ("address") u16 4610 ("address") u16 4610 ("address") u16 4610 ("address")] -> w235
          tunnel: [u16 1 ("address") u16 2 ("address") u16 3 ("address") u16 4 ("address") u16 5 ("address") u16 6 ("address") u16 7 ("address") u16 8 ("address") u16 9 ("holding register value") u16 10 ("holding register value") u16 11 ("holding register value") u16 12 ("address") u16 0 ("address")] -> w232
          frame 0 {
          }
          frame 1 {
          }
          frame 2 {
          }
          frame 3 {
          }
          frame 4 {
          }
          frame 5 {
          }
          frame 6 {
          }
          frame 7 {
          }
          frame 8 {
          }
          frame 9 {
          }
          frame 10 {
          }
          frame 11 {
          }
          frame 12, Default {
          }
        }
        n128 = local write "枚举"(enum16{"读取数据", "写入数据", "读取写入DATABASE", "读取参数"}."写入数据" ("枚举")) -> ()
        n129 = Insert Into Array(array=u16[] [] ("values"), index=0 ("索引"), new element=w232) -> (w231:u16[])
        n130 = Bundle By Name(cluster=cluster{"starting address":u16, "values":u16[]} {"starting address"=0, "values"=[]}, "starting address"=w235, "values"=w231) -> (w237:cluster{"starting address":u16, "values":u16[]})
        n131 = Enqueue Element(queue=w236, element=w237) -> ()  [unwired: 2 in, 3 out]
      }
      event "启动": Mouse Down {
        n132 = event-data() -> ()  [unwired: 1 in, 8 out]
        n133 = flat-sequence {
          tunnel: w269 -> [w272]
          tunnel: [w272] -> w268
          tunnel: [w271] -> w265
          tunnel: w268 -> [w275]
          tunnel: [w275] -> w267
          tunnel: [w273] -> w266
          tunnel: w265 -> [w273]
          tunnel: w267 -> [w277]
          tunnel: w266 -> [w276]
          frame #0 {
            n134 = call "启动测量模式选择对话框.vi"() -> ("启动选择 2"=w271:u16)  [unwired: 11 in]
            "启动选择 2" <- w271
          }
          frame #1 {
            n135 = property on="启动选择 2" class="Ring (严格)"() -> ("RingText.Text"=w274:string)  [unwired: 2 in, 2 out]
            n136 = global write "COD测量模式全局.vi" "测量模式"(w274) -> ()
          }
          frame #2 {
            n137 = case shown="9, 默认" w276 {
              tunnel: [u16 4608 ("address") u16 4608 ("address") u16 4608 ("address") u16 4608 ("address") u16 4608 ("address") u16 4608 ("address") u16 4608 ("address") u16 4608 ("address") u16 4608 ("address") u16 4608 ("address")] -> w278
              tunnel: [u16 1 ("address") u16 2 ("address") u16 3 ("address") u16 4 ("address") u16 5 ("address") u16 7 ("address") u16 6 ("address") u16 8 ("address") u16 9 ("address") u16 0 ("address")] -> w279
              frame 0 {
              }
              frame 1 {
              }
              frame 2 {
              }
              frame 3 {
              }
              frame 4 {
              }
              frame 5 {
              }
              frame 6 {
              }
              frame 7 {
              }
              frame 8 {
              }
              frame 9, Default {
              }
            }
            n138 = Insert Into Array(array=u16[] [] ("values"), index=0 ("索引"), new element=w279) -> (w284:u16[])
            n139 = Bundle By Name(cluster=cluster{"starting address":u16, "values":u16[]} {"starting address"=0, "values"=[]}, "starting address"=w278, "values"=w284) -> (w281:cluster{"starting address":u16, "values":u16[]})
            n140 = Enqueue Element(queue=w277, element=w281) -> ()  [unwired: 2 in, 3 out]
          }
        }
        n141 = local write "枚举"(enum16{"读取数据", "写入数据", "读取写入DATABASE", "读取参数"}."写入数据" ("枚举")) -> ()
      }
      event "停止": Value Change {
        n142 = event-data() -> ()  [unwired: 1 in, 6 out]
        n143 = local write "枚举"(enum16{"读取数据", "写入数据", "读取写入DATABASE", "读取参数"}."写入数据" ("枚举")) -> ()
        n144 = Bundle By Name(cluster=cluster{"starting address":u16, "values":u16[]} {"starting address"=0, "values"=[]}, "starting address"=u16 4608, "values"=u16[] [11]) -> (w308:cluster{"starting address":u16, "values":u16[]})
        n145 = Enqueue Element(queue=w306, element=w308) -> ()  [unwired: 2 in, 3 out]
      }
      event "手动控制": Value Change {
        n146 = event-data() -> ()  [unwired: 1 in, 6 out]
        n147 = call "数字密码键盘.vi"() -> ("NewNumber"=w313:sgl)  [unwired: 1 in]
        n148 = Equal?(x=w313, y=8.0) -> (x = y?=w314:bool)
        n149 = case shown="真" w314 {
          tunnel: w312 -> [_ w318]
          tunnel: w311 -> [_ w317]
          frame False {
            n150 = call "窗口弹出对话框(子VI).vi"("消息"="密码错误") -> ()  [unwired: 10 in, 1 out]
          }
          frame True {
            n151 = call "CODMn手动控制框.vi"("Error in"=w317, "MB_Serial session"=w318) -> ()  [unwired: 10 in]
          }
        }
      }
      event "参数配置": Value Change {
        w322 = "CODMn是否切换量程" ("key")
        n152 = event-data() -> ()  [unwired: 1 in, 6 out]
        n153 = property on="窗格" class="Pane"("Origin"=T10 {"Horizontal"=0, "Vertical"=650} ("原点")) -> ()  [unwired: 2 in, 2 out]
        n154 = Bundle By Name(cluster=T4 {"starting address"=0, "number of holding registers"=0}, "starting address"=u16 4272, "number of holding registers"=u16 20) -> (w346:T4)
        n155 = local write "读取KB值"(FALSE ("读取KB值")) -> ()
        n156 = local write "枚举"(enum16{"读取数据", "写入数据", "读取写入DATABASE", "读取参数"}."读取参数" ("枚举")) -> ()
        n157 = Flush Queue(queue=w339, error in (no error)=w338) -> (queue out=w342:refnum<queue>, error out=w341:errorcluster)  [unwired: 1 out]
        n158 = Enqueue Element(queue=w342, element=w346, error in (no error)=w341) -> ()  [unwired: 1 in, 3 out]
        n159 = global read "COD浓度全局变量.vi" "配置文件ini"() -> (w330:string)
        n160 = call <vilib>:"Application Directory.vi"() -> ("Application Directory"=w334:path)
        n161 = Build Path(base path=w334, name or relative path=w330) -> (appended path=w333:path)
        n162 = call <vilib>:"Open Config Data.vi"("configuration file path"=w333) -> ("error out"=w335:errorcluster, "refnum"=w336:T9)  [unwired: 8 in, 1 out]
        n163 = call-poly <vilib>:"Read Key.vi"("section"=w322, "error in (no error)"=w335, "key"="自动切换量程", "refnum"=w336) -> ("error out"=w326:errorcluster, "value"=w331:bool, "refnum out"=w327:T9)  [unwired: 4 in, 1 out]
        n164 = local write "自动切换量程"(w331) -> ()
        n165 = call-poly <vilib>:"Read Key.vi"("section"=w322, "error in (no error)"=w326, "key"="低切高阈值", "refnum"=w327) -> ("error out"=w323:errorcluster, "value"=w325:dbl, "refnum out"=w324:T9)  [unwired: 4 in, 1 out]
        n166 = local write "低切高阈值"(w325) -> ()
        n167 = call-poly <vilib>:"Read Key.vi"("section"=w322, "error in (no error)"=w323, "key"="高切低阈值", "refnum"=w324) -> ("error out"=w319:errorcluster, "value"=w321:dbl, "refnum out"=w320:T9)  [unwired: 4 in, 1 out]
        n168 = local write "高切低阈值"(w321) -> ()
        n169 = call <vilib>:"Close Config Data.vi"("error in (no error)"=w319, "refnum"=w320) -> ()  [unwired: 8 in, 2 out]
      }
      event "校准配置": Value Change {
        n170 = event-data() -> ()  [unwired: 1 in, 6 out]
        n171 = property on="窗格" class="Pane"("Origin"=T10 {"Horizontal"=0, "Vertical"=1300} ("原点")) -> ()  [unwired: 2 in, 2 out]
        n172 = global read "COD浓度全局变量.vi" "配置文件ini"() -> (w348:string)
        n173 = call <vilib>:"Application Directory.vi"() -> ("Application Directory"=w398:path)
        n174 = Build Path(base path=w398, name or relative path=w348) -> (appended path=w397:path)
        n175 = call <vilib>:"Open Config Data.vi"("configuration file path"=w397) -> ("error out"=w367:errorcluster, "refnum"=w368:T9)  [unwired: 8 in, 1 out]
        n176 = call-poly <vilib>:"Read Key.vi"("section"="CODMn模型选择" ("key"), "error in (no error)"=w367, "key"="线性和多项式", "refnum"=w368) -> ("error out"=w363:errorcluster, "value"=w366:i32, "refnum out"=w364:T9)  [unwired: 4 in, 1 out]
        n177 = local write "模型"(w366) -> ()
        n178 = call-poly <vilib>:"Read Key.vi"("section"="标线选择", "error in (no error)"=w363, "key"="选用水样", "refnum"=w364) -> ("error out"=w361:errorcluster, "value"=w365:i32, "refnum out"=w362:T9)  [unwired: 4 in, 1 out]
        n179 = local write "选用水样"(w365) -> ()
        n180 = local read "量程选择"() -> (w374:enum16{"低量程", "高量程", "0-2量程"})
        n181 = case shown="0, 默认" w365 {
          tunnel: ["葡萄糖标线" ("section") "草酸钠标线" ("section")] -> w373
          frame 0, Default {
          }
          frame 1 {
          }
        }
        n182 = case shown="\"0-2量程\"" w374 {
          tunnel: ["低量程" "高量程" "0-2量程"] -> w372
          frame "低量程", Default {
          }
          frame "高量程" {
          }
          frame "0-2量程" {
          }
        }
        n183 = Concatenate Strings(w373, w372) -> (w371:string)
        n184 = call-poly <vilib>:"Read Key.vi"("section"=w371, "error in (no error)"=w361, "key"="浓度1", "refnum"=w362) -> ("error out"=w402:errorcluster, "value"=w400:dbl, "refnum out"=w401:T9)  [unwired: 4 in, 1 out]
        n185 = local write "浓度1"(w400) -> ()
        n186 = call-poly <vilib>:"Read Key.vi"("section"=w371, "error in (no error)"=w402, "key"="浓度2", "refnum"=w401) -> ("error out"=w416:errorcluster, "value"=w403:dbl, "refnum out"=w415:T9)  [unwired: 4 in, 1 out]
        n187 = local write "浓度2"(w403) -> ()
        n188 = call-poly <vilib>:"Read Key.vi"("section"=w371, "error in (no error)"=w416, "key"="浓度3", "refnum"=w415) -> ("error out"=w417:errorcluster, "value"=w405:dbl, "refnum out"=w414:T9)  [unwired: 4 in, 1 out]
        n189 = local write "浓度3"(w405) -> ()
        n190 = call-poly <vilib>:"Read Key.vi"("section"=w371, "error in (no error)"=w417, "key"="泵滴定数1", "refnum"=w414) -> ("error out"=w418:errorcluster, "value"=w407:dbl, "refnum out"=w413:T9)  [unwired: 4 in, 1 out]
        n191 = local write "泵滴定数1"(w407) -> ()
        n192 = call-poly <vilib>:"Read Key.vi"("section"=w371, "error in (no error)"=w418, "key"="泵滴定数2", "refnum"=w413) -> ("error out"=w412:errorcluster, "value"=w410:dbl, "refnum out"=w419:T9)  [unwired: 4 in, 1 out]
        n193 = local write "泵滴定数2"(w410) -> ()
        n194 = call-poly <vilib>:"Read Key.vi"("section"=w371, "error in (no error)"=w412, "key"="泵滴定数3", "refnum"=w419) -> ("error out"=w424:errorcluster, "value"=w423:dbl, "refnum out"=w420:T9)  [unwired: 4 in, 1 out]
        n195 = local write "泵滴定数3"(w423) -> ()
        n196 = call-poly <vilib>:"Read Key.vi"("section"=w371, "error in (no error)"=w424, "key"="浓度4", "refnum"=w420) -> ("error out"=w425:errorcluster, "value"=w354:dbl, "refnum out"=w421:T9)  [unwired: 4 in, 1 out]
        n197 = local write "浓度4"(w354) -> ()
        n198 = call-poly <vilib>:"Read Key.vi"("section"=w371, "error in (no error)"=w425, "key"="浓度5", "refnum"=w421) -> ("error out"=w359:errorcluster, "value"=w353:dbl, "refnum out"=w360:T9)  [unwired: 4 in, 1 out]
        n199 = local write "浓度5"(w353) -> ()
        n200 = call-poly <vilib>:"Read Key.vi"("section"=w371, "error in (no error)"=w359, "key"="泵滴定数4", "refnum"=w360) -> ("error out"=w426:errorcluster, "value"=w352:dbl, "refnum out"=w422:T9)  [unwired: 4 in, 1 out]
        n201 = local write "泵滴定数4"(w352) -> ()
        n202 = call-poly <vilib>:"Read Key.vi"("section"=w371, "error in (no error)"=w426, "key"="泵滴定数5", "refnum"=w422) -> ("error out"=w357:errorcluster, "value"=w351:dbl, "refnum out"=w358:T9)  [unwired: 4 in, 1 out]
        n203 = local write "泵滴定数5"(w351) -> ()
        n204 = call-poly <vilib>:"Read Key.vi"("section"=w371, "error in (no error)"=w357, "key"="当前选用的校准", "refnum"=w358) -> ("error out"=w393:errorcluster, "value"=w395:i32, "refnum out"=w394:T9)  [unwired: 4 in, 1 out]
        n205 = local write "当前校准"(w395) -> ()
        n206 = call-poly <vilib>:"Read Key.vi"("section"=w371, "error in (no error)"=w393, "key"="启用1", "refnum"=w394) -> ("error out"=w390:errorcluster, "value"=w379:bool, "refnum out"=w391:T9)  [unwired: 4 in, 1 out]
        n207 = local write "启用1"(w379) -> ()
        n208 = call-poly <vilib>:"Read Key.vi"("section"=w371, "error in (no error)"=w390, "key"="启用2", "refnum"=w391) -> ("error out"=w388:errorcluster, "value"=w378:bool, "refnum out"=w389:T9)  [unwired: 4 in, 1 out]
        n209 = local write "启用2"(w378) -> ()
        n210 = call-poly <vilib>:"Read Key.vi"("section"=w371, "error in (no error)"=w388, "key"="启用3", "refnum"=w389) -> ("error out"=w386:errorcluster, "value"=w377:bool, "refnum out"=w387:T9)  [unwired: 4 in, 1 out]
        n211 = local write "启用3"(w377) -> ()
        n212 = call-poly <vilib>:"Read Key.vi"("section"=w371, "error in (no error)"=w386, "key"="启用4", "refnum"=w387) -> ("error out"=w384:errorcluster, "value"=w350:bool, "refnum out"=w385:T9)  [unwired: 4 in, 1 out]
        n213 = local write "启用4"(w350) -> ()
        n214 = call-poly <vilib>:"Read Key.vi"("section"=w371, "error in (no error)"=w384, "key"="启用5", "refnum"=w385) -> ("error out"=w355:errorcluster, "value"=w349:bool, "refnum out"=w356:T9)  [unwired: 4 in, 1 out]
        n215 = local write "启用5"(w349) -> ()
        n216 = call <vilib>:"Close Config Data.vi"("error in (no error)"=w355, "refnum"=w356) -> ()  [unwired: 8 in, 2 out]
      }
      event "选用水样": Value Change {
        (unwired) "浓度6" ("key")
        n217 = event-data() -> ()  [unwired: 1 in, 6 out]
        n218 = property on="窗格" class="Pane"("Origin"=T10 {"Horizontal"=0, "Vertical"=1300} ("原点")) -> ()  [unwired: 2 in, 2 out]
        n219 = local read "量程选择"() -> (w451:enum16{"低量程", "高量程", "0-2量程"})
        n220 = global read "COD浓度全局变量.vi" "配置文件ini"() -> (w437:string)
        n221 = case shown="\"0-2量程\"" w451 {
          tunnel: ["低量程" "高量程" "0-2量程"] -> w452
          frame "低量程", Default {
          }
          frame "高量程" {
          }
          frame "0-2量程" {
          }
        }
        n222 = case shown="\"葡萄糖\", 默认" "选用水样" {
          tunnel: ["葡萄糖标线" ("section") "草酸钠标线" ("section")] -> w453
          frame "葡萄糖", Default {
          }
          frame "草酸钠" {
          }
        }
        n223 = call <vilib>:"Application Directory.vi"() -> ("Application Directory"=w476:path)
        n224 = Build Path(base path=w476, name or relative path=w437) -> (appended path=w475:path)
        n225 = call <vilib>:"Open Config Data.vi"("configuration file path"=w475) -> ("error out"=w477:errorcluster, "refnum"=w478:T9)  [unwired: 8 in, 1 out]
        n226 = Concatenate Strings(w453, w452) -> (w450:string)
        n227 = call-poly <vilib>:"Read Key.vi"("section"=w450, "error in (no error)"=w477, "key"="浓度1", "refnum"=w478) -> ("error out"=w482:errorcluster, "value"=w480:dbl, "refnum out"=w481:T9)  [unwired: 4 in, 1 out]
        n228 = local write "浓度1"(w480) -> ()
        n229 = call-poly <vilib>:"Read Key.vi"("section"=w450, "error in (no error)"=w482, "key"="浓度2", "refnum"=w481) -> ("error out"=w496:errorcluster, "value"=w483:dbl, "refnum out"=w495:T9)  [unwired: 4 in, 1 out]
        n230 = local write "浓度2"(w483) -> ()
        n231 = call-poly <vilib>:"Read Key.vi"("section"=w450, "error in (no error)"=w496, "key"="浓度3", "refnum"=w495) -> ("error out"=w497:errorcluster, "value"=w485:dbl, "refnum out"=w494:T9)  [unwired: 4 in, 1 out]
        n232 = local write "浓度3"(w485) -> ()
        n233 = call-poly <vilib>:"Read Key.vi"("section"=w450, "error in (no error)"=w497, "key"="泵滴定数1", "refnum"=w494) -> ("error out"=w498:errorcluster, "value"=w487:dbl, "refnum out"=w493:T9)  [unwired: 4 in, 1 out]
        n234 = local write "泵滴定数1"(w487) -> ()
        n235 = call-poly <vilib>:"Read Key.vi"("section"=w450, "error in (no error)"=w498, "key"="泵滴定数2", "refnum"=w493) -> ("error out"=w492:errorcluster, "value"=w490:dbl, "refnum out"=w499:T9)  [unwired: 4 in, 1 out]
        n236 = local write "泵滴定数2"(w490) -> ()
        n237 = call-poly <vilib>:"Read Key.vi"("section"=w450, "error in (no error)"=w492, "key"="泵滴定数3", "refnum"=w499) -> ("error out"=w504:errorcluster, "value"=w503:dbl, "refnum out"=w500:T9)  [unwired: 4 in, 1 out]
        n238 = local write "泵滴定数3"(w503) -> ()
        n239 = call-poly <vilib>:"Read Key.vi"("section"=w450, "error in (no error)"=w504, "key"="浓度4", "refnum"=w500) -> ("error out"=w505:errorcluster, "value"=w445:dbl, "refnum out"=w501:T9)  [unwired: 4 in, 1 out]
        n240 = local write "浓度4"(w445) -> ()
        n241 = call-poly <vilib>:"Read Key.vi"("section"=w450, "error in (no error)"=w505, "key"="浓度5", "refnum"=w501) -> ("error out"=w448:errorcluster, "value"=w444:dbl, "refnum out"=w449:T9)  [unwired: 4 in, 1 out]
        n242 = local write "浓度5"(w444) -> ()
        n243 = call-poly <vilib>:"Read Key.vi"("section"=w450, "error in (no error)"=w448, "key"="泵滴定数4", "refnum"=w449) -> ("error out"=w506:errorcluster, "value"=w443:dbl, "refnum out"=w502:T9)  [unwired: 4 in, 1 out]
        n244 = local write "泵滴定数4"(w443) -> ()
        n245 = call-poly <vilib>:"Read Key.vi"("section"=w450, "error in (no error)"=w506, "key"="泵滴定数5", "refnum"=w502) -> ("error out"=w446:errorcluster, "value"=w442:dbl, "refnum out"=w447:T9)  [unwired: 4 in, 1 out]
        n246 = local write "泵滴定数5"(w442) -> ()
        n247 = call-poly <vilib>:"Read Key.vi"("section"=w450, "error in (no error)"=w446, "key"="当前选用的校准", "refnum"=w447) -> ("error out"=w471:errorcluster, "value"=w473:i32, "refnum out"=w472:T9)  [unwired: 4 in, 1 out]
        n248 = local write "当前校准"(w473) -> ()
        n249 = call-poly <vilib>:"Read Key.vi"("section"=w450, "error in (no error)"=w471, "key"="启用1", "refnum"=w472) -> ("error out"=w468:errorcluster, "value"=w457:bool, "refnum out"=w469:T9)  [unwired: 4 in, 1 out]
        n250 = local write "启用1"(w457) -> ()
        n251 = call-poly <vilib>:"Read Key.vi"("section"=w450, "error in (no error)"=w468, "key"="启用2", "refnum"=w469) -> ("error out"=w466:errorcluster, "value"=w456:bool, "refnum out"=w467:T9)  [unwired: 4 in, 1 out]
        n252 = local write "启用2"(w456) -> ()
        n253 = call-poly <vilib>:"Read Key.vi"("section"=w450, "error in (no error)"=w466, "key"="启用3", "refnum"=w467) -> ("error out"=w464:errorcluster, "value"=w455:bool, "refnum out"=w465:T9)  [unwired: 4 in, 1 out]
        n254 = local write "启用3"(w455) -> ()
        n255 = call-poly <vilib>:"Read Key.vi"("section"=w450, "error in (no error)"=w464, "key"="启用4", "refnum"=w465) -> ("error out"=w462:errorcluster, "value"=w439:bool, "refnum out"=w463:T9)  [unwired: 4 in, 1 out]
        n256 = local write "启用4"(w439) -> ()
        n257 = call-poly <vilib>:"Read Key.vi"("section"=w450, "error in (no error)"=w462, "key"="启用5", "refnum"=w463) -> ("error out"=w440:errorcluster, "value"=w438:bool, "refnum out"=w441:T9)  [unwired: 4 in, 1 out]
        n258 = local write "启用5"(w438) -> ()
        n259 = call <vilib>:"Close Config Data.vi"("error in (no error)"=w440, "refnum"=w441) -> ()  [unwired: 8 in, 2 out]
      }
      event "量程选择": Value Change {
        n260 = event-data() -> ()  [unwired: 1 in, 6 out]
        n261 = property on="窗格" class="Pane"("Origin"=T10 {"Horizontal"=0, "Vertical"=1300} ("原点")) -> ()  [unwired: 2 in, 2 out]
        n262 = local read "选用水样"() -> (w534:enum16{"葡萄糖", "草酸钠"})
        n263 = global read "COD浓度全局变量.vi" "配置文件ini"() -> (w517:string)
        n264 = case shown="\"葡萄糖\", 默认" w534 {
          tunnel: ["葡萄糖标线" ("section") "草酸钠标线" ("section")] -> w533
          frame "葡萄糖", Default {
          }
          frame "草酸钠" {
          }
        }
        n265 = case shown="\"0-2量程\"" "量程选择" {
          tunnel: ["低量程" "高量程" "0-2量程"] -> w530
          frame "低量程", Default {
          }
          frame "高量程" {
          }
          frame "0-2量程" {
          }
        }
        n266 = call <vilib>:"Application Directory.vi"() -> ("Application Directory"=w556:path)
        n267 = Build Path(base path=w556, name or relative path=w517) -> (appended path=w555:path)
        n268 = call <vilib>:"Open Config Data.vi"("configuration file path"=w555) -> ("error out"=w557:errorcluster, "refnum"=w558:T9)  [unwired: 8 in, 1 out]
        n269 = Concatenate Strings(w533, w530) -> (w532:string)
        n270 = call-poly <vilib>:"Read Key.vi"("section"=w532, "error in (no error)"=w557, "key"="浓度1", "refnum"=w558) -> ("error out"=w562:errorcluster, "value"=w560:dbl, "refnum out"=w561:T9)  [unwired: 4 in, 1 out]
        n271 = local write "浓度1"(w560) -> ()
        n272 = call-poly <vilib>:"Read Key.vi"("section"=w532, "error in (no error)"=w562, "key"="浓度2", "refnum"=w561) -> ("error out"=w576:errorcluster, "value"=w563:dbl, "refnum out"=w575:T9)  [unwired: 4 in, 1 out]
        n273 = local write "浓度2"(w563) -> ()
        n274 = call-poly <vilib>:"Read Key.vi"("section"=w532, "error in (no error)"=w576, "key"="浓度3", "refnum"=w575) -> ("error out"=w577:errorcluster, "value"=w565:dbl, "refnum out"=w574:T9)  [unwired: 4 in, 1 out]
        n275 = local write "浓度3"(w565) -> ()
        n276 = call-poly <vilib>:"Read Key.vi"("section"=w532, "error in (no error)"=w577, "key"="泵滴定数1", "refnum"=w574) -> ("error out"=w578:errorcluster, "value"=w567:dbl, "refnum out"=w573:T9)  [unwired: 4 in, 1 out]
        n277 = local write "泵滴定数1"(w567) -> ()
        n278 = call-poly <vilib>:"Read Key.vi"("section"=w532, "error in (no error)"=w578, "key"="泵滴定数2", "refnum"=w573) -> ("error out"=w572:errorcluster, "value"=w570:dbl, "refnum out"=w579:T9)  [unwired: 4 in, 1 out]
        n279 = local write "泵滴定数2"(w570) -> ()
        n280 = call-poly <vilib>:"Read Key.vi"("section"=w532, "error in (no error)"=w572, "key"="泵滴定数3", "refnum"=w579) -> ("error out"=w584:errorcluster, "value"=w583:dbl, "refnum out"=w580:T9)  [unwired: 4 in, 1 out]
        n281 = local write "泵滴定数3"(w583) -> ()
        n282 = call-poly <vilib>:"Read Key.vi"("section"=w532, "error in (no error)"=w584, "key"="浓度4", "refnum"=w580) -> ("error out"=w585:errorcluster, "value"=w521:dbl, "refnum out"=w581:T9)  [unwired: 4 in, 1 out]
        n283 = local write "浓度4"(w521) -> ()
        n284 = call-poly <vilib>:"Read Key.vi"("section"=w532, "error in (no error)"=w585, "key"="浓度5", "refnum"=w581) -> ("error out"=w528:errorcluster, "value"=w520:dbl, "refnum out"=w529:T9)  [unwired: 4 in, 1 out]
        n285 = local write "浓度5"(w520) -> ()
        n286 = call-poly <vilib>:"Read Key.vi"("section"=w532, "error in (no error)"=w528, "key"="泵滴定数4", "refnum"=w529) -> ("error out"=w586:errorcluster, "value"=w519:dbl, "refnum out"=w582:T9)  [unwired: 4 in, 1 out]
        n287 = local write "泵滴定数4"(w519) -> ()
        n288 = call-poly <vilib>:"Read Key.vi"("section"=w532, "error in (no error)"=w586, "key"="泵滴定数5", "refnum"=w582) -> ("error out"=w526:errorcluster, "value"=w518:dbl, "refnum out"=w527:T9)  [unwired: 4 in, 1 out]
        n289 = local write "泵滴定数5"(w518) -> ()
        n290 = call-poly <vilib>:"Read Key.vi"("section"=w532, "error in (no error)"=w526, "key"="当前选用的校准", "refnum"=w527) -> ("error out"=w551:errorcluster, "value"=w553:i32, "refnum out"=w552:T9)  [unwired: 4 in, 1 out]
        n291 = local write "当前校准"(w553) -> ()
        n292 = call-poly <vilib>:"Read Key.vi"("section"=w532, "error in (no error)"=w551, "key"="启用1", "refnum"=w552) -> ("error out"=w548:errorcluster, "value"=w537:bool, "refnum out"=w549:T9)  [unwired: 4 in, 1 out]
        n293 = local write "启用1"(w537) -> ()
        n294 = call-poly <vilib>:"Read Key.vi"("section"=w532, "error in (no error)"=w548, "key"="启用2", "refnum"=w549) -> ("error out"=w546:errorcluster, "value"=w536:bool, "refnum out"=w547:T9)  [unwired: 4 in, 1 out]
        n295 = local write "启用2"(w536) -> ()
        n296 = call-poly <vilib>:"Read Key.vi"("section"=w532, "error in (no error)"=w546, "key"="启用3", "refnum"=w547) -> ("error out"=w544:errorcluster, "value"=w535:bool, "refnum out"=w545:T9)  [unwired: 4 in, 1 out]
        n297 = local write "启用3"(w535) -> ()
        n298 = call-poly <vilib>:"Read Key.vi"("section"=w532, "error in (no error)"=w544, "key"="启用4", "refnum"=w545) -> ("error out"=w542:errorcluster, "value"=w523:bool, "refnum out"=w543:T9)  [unwired: 4 in, 1 out]
        n299 = local write "启用4"(w523) -> ()
        n300 = call-poly <vilib>:"Read Key.vi"("section"=w532, "error in (no error)"=w542, "key"="启用5", "refnum"=w543) -> ("error out"=w524:errorcluster, "value"=w522:bool, "refnum out"=w525:T9)  [unwired: 4 in, 1 out]
        n301 = local write "启用5"(w522) -> ()
        n302 = call <vilib>:"Close Config Data.vi"("error in (no error)"=w524, "refnum"=w525) -> ()  [unwired: 8 in, 2 out]
      }
      event "测量模式(公式)": Value Change {
        n303 = event-data() -> ()  [unwired: 1 in, 6 out]
        n304 = flat-sequence {
          frame #0 {
            n305 = local read "测量模式(公式)"() -> (w597:u16)
            n306 = global write "CODMn断电保存全局变量.vi" "测量模式(公式)"(w597) -> ()
          }
          frame #1 {
            n307 = call <vilib>:"Application Directory.vi"() -> ("Application Directory"=w611:path)
            n308 = Build Path(base path=w611, name or relative path="data\\sys.ini" ("名称或相对路径")) -> (appended path=w609:path)
            n309 = call <vilib>:"Open Config Data.vi"("configuration file path"=w609) -> ("error out"=w605:errorcluster, "refnum"=w608:T9)  [unwired: 8 in, 1 out]
            n310 = vi-ref "斯坦道CODMn.lvlib:CODMn断电保存全局变量.vi"() -> (w607:refnum<vi>)
            n311 = call <userlib>:"Write Panel to INI__ogtk.vi"("error in (no error)"=w605, "VI ref"=w607, "refnum"=w608) -> ("error out"=w604:errorcluster, "refnum out"=w606:T9)  [unwired: 7 in]
            n312 = call <vilib>:"Close Config Data.vi"("error in (no error)"=w604, "refnum"=w606) -> ("error out"=w599:errorcluster, "file path"=w598:path)  [unwired: 8 in]
            n313 = Open/Create/Replace File(file path (use dialog)=w598, error in=w599) -> (refnum out=w602:refnum<file>, error out=w603:errorcluster)  [unwired: 4 in, 1 out]
            n314 = Flush File(refnum=w602, error in=w603) -> (refnum out=w601:refnum<file>, error out=w600:errorcluster)
            n315 = Close File(refnum=w601, error in=w600) -> ()  [unwired: 2 out]
          }
        }
      }
      event "周期设置": Value Change {
        n316 = event-data() -> ()  [unwired: 1 in, 6 out]
        n317 = call "数字密码键盘.vi"() -> ("NewNumber"=w612:sgl)  [unwired: 1 in]
        n318 = Equal?(x=w612, y=8.0) -> (x = y?=w613:bool)
        n319 = case shown="真" w613 {
          frame False {
            n320 = call "窗口弹出对话框(子VI).vi"("消息"="密码错误") -> ()  [unwired: 10 in, 1 out]
          }
          frame True {
            n321 = call "窗口弹出对话框(子VI).vi"("消息"="登录成功") -> ("true"=w616:bool)  [unwired: 10 in]
            n322 = case shown="真" w616 {
              frame False {
              }
              frame True {
                n323 = property on="窗格" class="Pane"("Origin"=T10 {"Horizontal"=0, "Vertical"=1950} ("原点")) -> ()  [unwired: 2 in, 2 out]
              }
            }
          }
        }
      }
      event "返回": Value Change {
        (unwired) "泵滴定数6" ("key")
        w633 = "CODMn" ("section")
        n324 = event-data() -> ()  [unwired: 1 in, 6 out]
        n325 = property on="窗格" class="Pane"("Origin"=T10 {"Horizontal"=0, "Vertical"=0} ("原点")) -> ()  [unwired: 2 in, 2 out]
        n326 = global read "COD浓度全局变量.vi" "配置文件ini"() -> (w619:string)
        n327 = call <vilib>:"Application Directory.vi"() -> ("Application Directory"=w685:path)
        n328 = Build Path(base path=w685, name or relative path=w619) -> (appended path=w684:path)
        n329 = local write "读取KB值"(FALSE ("读取KB值")) -> ()
        n330 = call <vilib>:"Open Config Data.vi"("configuration file path"=w684) -> ("error out"=w682:errorcluster, "refnum"=w683:T9)  [unwired: 8 in, 1 out]
        n331 = local read "浓度1"() -> (w680:dbl)
        n332 = local read "浓度2"() -> (w664:dbl)
        n333 = call-poly <vilib>:"Write Key.vi"("section"=w633, "error in (no error)"=w682, "value"=w680, "key"="浓度1", "refnum"=w683) -> ("error out"=w679:errorcluster, "refnum out"=w678:T9)  [unwired: 4 in, 1 out]
        n334 = local read "浓度3"() -> (w660:dbl)
        n335 = call-poly <vilib>:"Write Key.vi"("section"=w633, "error in (no error)"=w679, "value"=w664, "key"="浓度2", "refnum"=w678) -> ("error out"=w677:errorcluster, "refnum out"=w676:T9)  [unwired: 4 in, 1 out]
        n336 = local read "泵滴定数1"() -> (w658:dbl)
        n337 = call-poly <vilib>:"Write Key.vi"("section"=w633, "error in (no error)"=w677, "value"=w660, "key"="浓度3", "refnum"=w676) -> ("error out"=w675:errorcluster, "refnum out"=w674:T9)  [unwired: 4 in, 1 out]
        n338 = call-poly <vilib>:"Write Key.vi"("section"=w633, "error in (no error)"=w675, "value"=w658, "key"="泵滴定数1", "refnum"=w674) -> ("error out"=w673:errorcluster, "refnum out"=w672:T9)  [unwired: 4 in, 1 out]
        n339 = local read "泵滴定数2"() -> (w656:dbl)
        n340 = call-poly <vilib>:"Write Key.vi"("section"=w633, "error in (no error)"=w673, "value"=w656, "key"="泵滴定数2", "refnum"=w672) -> ("error out"=w671:errorcluster, "refnum out"=w670:T9)  [unwired: 4 in, 1 out]
        n341 = local read "泵滴定数3"() -> (w654:dbl)
        n342 = local read "浓度4"() -> (w621:dbl)
        n343 = call-poly <vilib>:"Write Key.vi"("section"=w633, "error in (no error)"=w671, "value"=w654, "key"="泵滴定数3", "refnum"=w670) -> ("error out"=w669:errorcluster, "refnum out"=w668:T9)  [unwired: 4 in, 1 out]
        n344 = call-poly <vilib>:"Write Key.vi"("section"=w633, "error in (no error)"=w669, "value"=w621, "key"="浓度4", "refnum"=w668) -> ("error out"=w662:errorcluster, "refnum out"=w663:T9)  [unwired: 4 in, 1 out]
        n345 = local read "浓度5"() -> (w620:dbl)
        n346 = call-poly <vilib>:"Write Key.vi"("section"=w633, "error in (no error)"=w662, "value"=w620, "key"="浓度5", "refnum"=w663) -> ("error out"=w630:errorcluster, "refnum out"=w631:T9)  [unwired: 4 in, 1 out]
        n347 = local read "泵滴定数4"() -> (w622:dbl)
        n348 = call-poly <vilib>:"Write Key.vi"("section"=w633, "error in (no error)"=w630, "value"=w622, "key"="泵滴定数4", "refnum"=w631) -> ("error out"=w667:errorcluster, "refnum out"=w666:T9)  [unwired: 4 in, 1 out]
        n349 = local read "泵滴定数5"() -> (w623:dbl)
        n350 = call-poly <vilib>:"Write Key.vi"("section"=w633, "error in (no error)"=w667, "value"=w623, "key"="泵滴定数5", "refnum"=w666) -> ("error out"=w628:errorcluster, "refnum out"=w629:T9)  [unwired: 4 in, 1 out]
        n351 = local read "启用1"() -> (w642:bool)
        n352 = call-poly <vilib>:"Write Key.vi"("section"=w633, "error in (no error)"=w628, "value"=w642, "key"="启用1", "refnum"=w629) -> ("error out"=w638:errorcluster, "refnum out"=w641:T9)  [unwired: 4 in, 1 out]
        n353 = local read "启用2"() -> (w639:bool)
        n354 = call-poly <vilib>:"Write Key.vi"("section"=w633, "error in (no error)"=w638, "value"=w639, "key"="启用2", "refnum"=w641) -> ("error out"=w649:errorcluster, "refnum out"=w648:T9)  [unwired: 4 in, 1 out]
        n355 = local read "启用3"() -> (w637:bool)
        n356 = call-poly <vilib>:"Write Key.vi"("section"=w633, "error in (no error)"=w649, "value"=w637, "key"="启用3", "refnum"=w648) -> ("error out"=w647:errorcluster, "refnum out"=w646:T9)  [unwired: 4 in, 1 out]
        n357 = local read "启用4"() -> (w625:bool)
        n358 = call-poly <vilib>:"Write Key.vi"("section"=w633, "error in (no error)"=w647, "value"=w625, "key"="启用4", "refnum"=w646) -> ("error out"=w645:errorcluster, "refnum out"=w644:T9)  [unwired: 4 in, 1 out]
        n359 = local read "启用5"() -> (w624:bool)
        n360 = call-poly <vilib>:"Write Key.vi"("section"=w633, "error in (no error)"=w645, "value"=w624, "key"="启用5", "refnum"=w644) -> ("error out"=w626:errorcluster, "refnum out"=w627:T9)  [unwired: 4 in, 1 out]
        n361 = call <vilib>:"Close Config Data.vi"("error in (no error)"=w626, "refnum"=w627) -> ()  [unwired: 8 in, 2 out]
      }
      event "关闭", "关闭 2", "关闭 3": Value Change {
        n362 = event-data() -> ()  [unwired: 1 in, 6 out]
        n363 = property on="窗格" class="Pane"("Origin"=T10 {"Horizontal"=0, "Vertical"=0} ("原点")) -> ()  [unwired: 2 in, 2 out]
      }
      event Timeout; Application Instance Close {
        n364 = event-data() -> ()  [unwired: 1 in, 3 out]
        n365 = call-dynamic "Close Session.vi"("error in (no error)"=w688, "MB_Serial session"=w689) -> ()  [unwired: 9 in, 1 out]
      }
      event "时间校准": Value Change {
        n366 = event-data() -> ()  [unwired: 1 in, 6 out]
        n367 = flat-sequence {
          tunnel: w690 -> [w695]
          frame #0 {
            n368 = Get Date/Time In Seconds() -> (seconds since 1Jan1904=w700:timestamp)
            n369 = Build Array(w700) -> (w699:timestamp[])
            n370 = call "DateToHex.vi"("DATE"=w699) -> ("数组"=w693:u16[])  [unwired: 10 in]
            n371 = Insert Into Array(array=u16[] [1] ("values"), index=1 ("索引"), new element=w693) -> (w691:u16[])
            n372 = Bundle By Name(cluster=cluster{"starting address":u16, "values":u16[]} {"starting address"=0, "values"=[]}, "starting address"=u16 4612, "values"=w691) -> (w696:cluster{"starting address":u16, "values":u16[]})
            n373 = Enqueue Element(queue=w695, element=w696) -> ()  [unwired: 2 in, 3 out]
          }
          frame #1 {
            n374 = local write "枚举"(enum16{"读取数据", "写入数据", "读取写入DATABASE", "读取参数"}."写入数据" ("枚举")) -> ()
          }
        }
      }
      event "故障清除": Value Change {
        n375 = event-data() -> ()  [unwired: 1 in, 6 out]
        n376 = local write "枚举"(enum16{"读取数据", "写入数据", "读取写入DATABASE", "读取参数"}."写入数据" ("枚举")) -> ()
        n377 = Bundle By Name(cluster=cluster{"starting address":u16, "values":u16[]} {"starting address"=0, "values"=[]}, "starting address"=u16 4611, "values"=u16[] [1]) -> (w705:cluster{"starting address":u16, "values":u16[]})
        n378 = Enqueue Element(queue=w704, element=w705) -> ()  [unwired: 2 in, 3 out]
      }
      event "定时启动": Mouse Down {
        n379 = event-data() -> ()  [unwired: 1 in, 8 out]
        n380 = flat-sequence {
          frame #0 {
            n381 = global read "CODMn断电保存全局变量.vi" "定时控制"() -> (w708:T6)
            n382 = call "周期设置.vi"("定时控制参数输入"=w708) -> ("定时控制参数输出"=w709:T6)  [unwired: 10 in]
            n383 = global write "CODMn断电保存全局变量.vi" "定时控制"(w709) -> ()
          }
          frame #1 {
            n384 = global read "COD浓度全局变量.vi" "序列号:"() -> (w714:string)
            n385 = Concatenate Strings("data\\" ("字符串"), "序列号" ("字符串"), w714, "sys.ini" ("名称或相对路径")) -> (w715:string)
            n386 = call <vilib>:"Application Directory.vi"() -> ("Application Directory"=w710:path)
            n387 = Build Path(base path=w710, name or relative path=w715) -> (appended path=w716:path)
            n388 = call <vilib>:"Open Config Data.vi"("configuration file path"=w716) -> ("error out"=w719:errorcluster, "refnum"=w717:T9)  [unwired: 8 in, 1 out]
            n389 = vi-ref "斯坦道CODMn.lvlib:CODMn断电保存全局变量.vi"() -> (w718:refnum<vi>)
            n390 = call <userlib>:"Write Panel to INI__ogtk.vi"("error in (no error)"=w719, "VI ref"=w718, "refnum"=w717) -> ("error out"=w721:errorcluster, "refnum out"=w720:T9)  [unwired: 7 in]
            n391 = call <vilib>:"Close Config Data.vi"("error in (no error)"=w721, "refnum"=w720) -> ("error out"=w723:errorcluster, "file path"=w722:path)  [unwired: 8 in]
            n392 = Open/Create/Replace File(file path (use dialog)=w722, error in=w723) -> (refnum out=w724:refnum<file>, error out=w725:errorcluster)  [unwired: 4 in, 1 out]
            n393 = Flush File(refnum=w724, error in=w725) -> (refnum out=w726:refnum<file>, error out=w727:errorcluster)
            n394 = Close File(refnum=w726, error in=w727) -> ()  [unwired: 2 out]
          }
        }
      }
      event "校准1", "校准2", "校准3", "校准4", "校准5": Value Change {
        n395 = event-data() -> ()  [unwired: 1 in, 6 out]
        n396 = flat-sequence {
          tunnel: w730 -> [w735]
          tunnel: [w734] -> w729
          tunnel: [w733] -> w728
          tunnel: w729 -> [w768]
          tunnel: w728 -> [w767]
          frame #0 {
            n397 = Build Array("校准1", "校准2", "校准3", "校准4", "校准5") -> (w736:bool[])
            n398 = for {
              tunnel: w736 -> [w750] mode=indexing
              tunnel: w735 -> [w746]
              tunnel: [w742] -> w734
              tunnel: [w741] -> w733
              i -> [w740]
              n399 = case shown="4" w740 {
                tunnel: ["浓度1" "浓度2" "浓度3" "浓度4" "浓度5"] -> w745
                frame 0, Default {
                }
                frame 1 {
                }
                frame 2 {
                }
                frame 3 {
                }
                frame 4 {
                }
              }
              n400 = Multiply(x=w745, y=100.0) -> (x*y=w743:dbl)
              n401 = Insert Into Array(array=u16[] [] ("values"), index=0 ("索引"), new element=w743) -> (w747:u16[])
              n402 = case shown="真" w750 {
                tunnel: w747 -> [_ w762]
                tunnel: w746 -> [w756 w761]
                tunnel: [w756 w760] -> w742
                tunnel: [_ w759] -> w741
                tunnel: w740 -> [_ w758]
                frame False {
                }
                frame True {
                  n403 = Increment(x=w758) -> (x+1=→"当前校准":i32)
                  n404 = Bundle By Name(cluster=cluster{"starting address":u16, "values":u16[]} {"starting address"=4272, "values"=[]}, "starting address"=u16 4274, "values"=w762) -> (w764:cluster{"starting address":u16, "values":u16[]})
                  n405 = Enqueue Element(queue=w761, element=w764) -> (queue out=w760:refnum<queue>, error out=w759:errorcluster)  [unwired: 2 in, 1 out]
                }
              }
            }
          }
          frame #1 {
            n406 = local read "当前校准"() -> (w773:i32)
            n407 = case shown="5" w773 {
              tunnel: [w779 w780 w781 w782 w783] -> w772
              frame 1, Default {
                n408 = local read "浓度1"() -> (w779:dbl)
              }
              frame 2 {
                n409 = local read "浓度2"() -> (w780:dbl)
              }
              frame 3 {
                n410 = local read "浓度3"() -> (w781:dbl)
              }
              frame 4 {
                n411 = local read "浓度4"() -> (w782:dbl)
              }
              frame 5 {
                n412 = local read "浓度5"() -> (w783:dbl)
              }
            }
            n413 = Not Equal To 0?(x=w772) -> (x != 0?=w771:bool)
            n414 = case shown="假" w771 {
              tunnel: [u16 8 ("address") u16 9 ("address")] -> w776
              tunnel: ["校零" ("测量模式") "校标" ("测量模式")] -> w766
              frame False {
              }
              frame True {
              }
            }
            n415 = global write "COD测量模式全局.vi" "测量模式"(w766) -> ()
            n416 = Insert Into Array(array=u16[] [] ("values"), index=0 ("索引"), new element=w776) -> (w770:u16[])
            n417 = Bundle By Name(cluster=cluster{"starting address":u16, "values":u16[]} {"starting address"=0, "values"=[]}, "starting address"=u16 4608 ("address"), "values"=w770) -> (w778:cluster{"starting address":u16, "values":u16[]})
            n418 = Enqueue Element(queue=w768, element=w778, error in (no error)=w767) -> ()  [unwired: 1 in, 3 out]
          }
          frame #2 {
            n419 = global read "COD浓度全局变量.vi" "配置文件ini"() -> (w788:string)
            n420 = local write "枚举"(enum16{"读取数据", "写入数据", "读取写入DATABASE", "读取参数"}."写入数据" ("枚举")) -> ()
            n421 = call <vilib>:"Application Directory.vi"() -> ("Application Directory"=w796:path)
            n422 = Build Path(base path=w796, name or relative path=w788) -> (appended path=w797:path)
            n423 = local read "当前校准"() -> (w791:i32)
            n424 = call <vilib>:"Open Config Data.vi"("configuration file path"=w797) -> ("error out"=w794:errorcluster, "refnum"=w795:T9)  [unwired: 8 in, 1 out]
            n425 = call-poly <vilib>:"Write Key.vi"("section"="CODMn", "error in (no error)"=w794, "value"=w791, "key"="当前选用的校准" ("section"), "refnum"=w795) -> ("error out"=w789:errorcluster, "refnum out"=w790:T9)  [unwired: 4 in, 1 out]
            n426 = call <vilib>:"Close Config Data.vi"("error in (no error)"=w789, "refnum"=w790) -> ()  [unwired: 8 in, 2 out]
          }
        }
      }
      event "自动切换量程", "低切高阈值", "高切低阈值": Value Change {
        w809 = "CODMn是否切换量程" ("key")
        n427 = event-data() -> ()  [unwired: 1 in, 6 out]
        n428 = global read "COD浓度全局变量.vi" "配置文件ini"() -> (w810:string)
        n429 = call <vilib>:"Application Directory.vi"() -> ("Application Directory"=w816:path)
        n430 = Build Path(base path=w816, name or relative path=w810) -> (appended path=w815:path)
        n431 = local read "自动切换量程"() -> (w811:bool)
        n432 = call <vilib>:"Open Config Data.vi"("configuration file path"=w815) -> ("error out"=w813:errorcluster, "refnum"=w814:T9)  [unwired: 8 in, 1 out]
        n433 = call-poly <vilib>:"Write Key.vi"("section"=w809, "error in (no error)"=w813, "value"=w811, "key"="自动切换量程", "refnum"=w814) -> ("error out"=w806:errorcluster, "refnum out"=w808:T9)  [unwired: 4 in, 1 out]
        n434 = local read "低切高阈值"() -> (w800:dbl)
        n435 = call-poly <vilib>:"Write Key.vi"("section"=w809, "error in (no error)"=w806, "value"=w800, "key"="低切高阈值", "refnum"=w808) -> ("error out"=w803:errorcluster, "refnum out"=w805:T9)  [unwired: 4 in, 1 out]
        n436 = local read "高切低阈值"() -> (w799:dbl)
        n437 = call-poly <vilib>:"Write Key.vi"("section"=w809, "error in (no error)"=w803, "value"=w799, "key"="高切低阈值", "refnum"=w805) -> ("error out"=w801:errorcluster, "refnum out"=w802:T9)  [unwired: 4 in, 1 out]
        n438 = call <vilib>:"Close Config Data.vi"("error in (no error)"=w801, "refnum"=w802) -> ()  [unwired: 8 in, 2 out]
      }
      event "模型": Value Change {
        n439 = event-data() -> ()  [unwired: 1 in, 6 out]
        n440 = global read "COD浓度全局变量.vi" "配置文件ini"() -> (w817:string)
        n441 = call <vilib>:"Application Directory.vi"() -> ("Application Directory"=w826:path)
        n442 = Build Path(base path=w826, name or relative path=w817) -> (appended path=w825:path)
        n443 = call <vilib>:"Open Config Data.vi"("configuration file path"=w825) -> ("error out"=w823:errorcluster, "refnum"=w824:T9)  [unwired: 8 in, 1 out]
        n444 = local read "模型"() -> (w818:enum32{"线性", "多项式"})
        n445 = call-poly <vilib>:"Write Key.vi"("section"="CODMn模型选择" ("key"), "error in (no error)"=w823, "value"=w818, "key"="线性和多项式", "refnum"=w824) -> ("error out"=w819:errorcluster, "refnum out"=w820:T9)  [unwired: 4 in, 1 out]
        n446 = call <vilib>:"Close Config Data.vi"("error in (no error)"=w819, "refnum"=w820) -> ()  [unwired: 8 in, 2 out]
      }
      event "浓度1", "浓度2", "浓度3", "泵滴定数1", "泵滴定数2", "泵滴定数3", "启用1", "启用2", "启用3", "浓度4", "浓度5", "泵滴定数4", "泵滴定数5", "启用4", "启用5": Value Change {
        n447 = event-data() -> ()  [unwired: 1 in, 6 out]
        n448 = global read "COD浓度全局变量.vi" "配置文件ini"() -> (w827:string)
        n449 = local read "选用水样"() -> (w843:enum16{"葡萄糖", "草酸钠"})
        n450 = local read "量程选择"() -> (w842:enum16{"低量程", "高量程", "0-2量程"})
        n451 = case shown="\"0-2量程\"" w842 {
          tunnel: ["低量程" "高量程" "0-2量程"] -> w840
          frame "低量程", Default {
          }
          frame "高量程" {
          }
          frame "0-2量程" {
          }
        }
        n452 = call <vilib>:"Application Directory.vi"() -> ("Application Directory"=w901:path)
        n453 = case shown="\"葡萄糖\", 默认" w843 {
          tunnel: ["葡萄糖标线" ("section") "草酸钠标线" ("section")] -> w849
          frame "葡萄糖", Default {
          }
          frame "草酸钠" {
          }
        }
        n454 = Build Path(base path=w901, name or relative path=w827) -> (appended path=w900:path)
        n455 = call <vilib>:"Open Config Data.vi"("configuration file path"=w900) -> ("error out"=w898:errorcluster, "refnum"=w899:T9)  [unwired: 8 in, 1 out]
        n456 = local read "浓度1"() -> (w896:dbl)
        n457 = Concatenate Strings(w849, w840) -> (w841:string)
        n458 = local read "浓度2"() -> (w880:dbl)
        n459 = call-poly <vilib>:"Write Key.vi"("section"=w841, "error in (no error)"=w898, "value"=w896, "key"="浓度1", "refnum"=w899) -> ("error out"=w895:errorcluster, "refnum out"=w894:T9)  [unwired: 4 in, 1 out]
        n460 = local read "浓度3"() -> (w876:dbl)
        n461 = call-poly <vilib>:"Write Key.vi"("section"=w841, "error in (no error)"=w895, "value"=w880, "key"="浓度2", "refnum"=w894) -> ("error out"=w893:errorcluster, "refnum out"=w892:T9)  [unwired: 4 in, 1 out]
        n462 = local read "泵滴定数1"() -> (w874:dbl)
        n463 = call-poly <vilib>:"Write Key.vi"("section"=w841, "error in (no error)"=w893, "value"=w876, "key"="浓度3", "refnum"=w892) -> ("error out"=w891:errorcluster, "refnum out"=w890:T9)  [unwired: 4 in, 1 out]
        n464 = call-poly <vilib>:"Write Key.vi"("section"=w841, "error in (no error)"=w891, "value"=w874, "key"="泵滴定数1", "refnum"=w890) -> ("error out"=w889:errorcluster, "refnum out"=w888:T9)  [unwired: 4 in, 1 out]
        n465 = local read "泵滴定数2"() -> (w872:dbl)
        n466 = call-poly <vilib>:"Write Key.vi"("section"=w841, "error in (no error)"=w889, "value"=w872, "key"="泵滴定数2", "refnum"=w888) -> ("error out"=w887:errorcluster, "refnum out"=w886:T9)  [unwired: 4 in, 1 out]
        n467 = local read "泵滴定数3"() -> (w870:dbl)
        n468 = local read "浓度4"() -> (w839:dbl)
        n469 = call-poly <vilib>:"Write Key.vi"("section"=w841, "error in (no error)"=w887, "value"=w870, "key"="泵滴定数3", "refnum"=w886) -> ("error out"=w885:errorcluster, "refnum out"=w884:T9)  [unwired: 4 in, 1 out]
        n470 = local read "浓度5"() -> (w838:dbl)
        n471 = call-poly <vilib>:"Write Key.vi"("section"=w841, "error in (no error)"=w885, "value"=w839, "key"="浓度4", "refnum"=w884) -> ("error out"=w878:errorcluster, "refnum out"=w879:T9)  [unwired: 4 in, 1 out]
        n472 = call-poly <vilib>:"Write Key.vi"("section"=w841, "error in (no error)"=w878, "value"=w838, "key"="浓度5", "refnum"=w879) -> ("error out"=w836:errorcluster, "refnum out"=w837:T9)  [unwired: 4 in, 1 out]
        n473 = local read "泵滴定数4"() -> (w835:dbl)
        n474 = call-poly <vilib>:"Write Key.vi"("section"=w841, "error in (no error)"=w836, "value"=w835, "key"="泵滴定数4", "refnum"=w837) -> ("error out"=w883:errorcluster, "refnum out"=w882:T9)  [unwired: 4 in, 1 out]
        n475 = local read "泵滴定数5"() -> (w834:dbl)
        n476 = call-poly <vilib>:"Write Key.vi"("section"=w841, "error in (no error)"=w883, "value"=w834, "key"="泵滴定数5", "refnum"=w882) -> ("error out"=w832:errorcluster, "refnum out"=w833:T9)  [unwired: 4 in, 1 out]
        n477 = local read "启用1"() -> (w858:bool)
        n478 = call-poly <vilib>:"Write Key.vi"("section"=w841, "error in (no error)"=w832, "value"=w858, "key"="启用1", "refnum"=w833) -> ("error out"=w854:errorcluster, "refnum out"=w857:T9)  [unwired: 4 in, 1 out]
        n479 = local read "启用2"() -> (w855:bool)
        n480 = call-poly <vilib>:"Write Key.vi"("section"=w841, "error in (no error)"=w854, "value"=w855, "key"="启用2", "refnum"=w857) -> ("error out"=w865:errorcluster, "refnum out"=w864:T9)  [unwired: 4 in, 1 out]
        n481 = local read "启用3"() -> (w853:bool)
        n482 = call-poly <vilib>:"Write Key.vi"("section"=w841, "error in (no error)"=w865, "value"=w853, "key"="启用3", "refnum"=w864) -> ("error out"=w863:errorcluster, "refnum out"=w862:T9)  [unwired: 4 in, 1 out]
        n483 = local read "启用4"() -> (w828:bool)
        n484 = call-poly <vilib>:"Write Key.vi"("section"=w841, "error in (no error)"=w863, "value"=w828, "key"="启用4", "refnum"=w862) -> ("error out"=w861:errorcluster, "refnum out"=w860:T9)  [unwired: 4 in, 1 out]
        n485 = local read "启用5"() -> (w829:bool)
        n486 = call-poly <vilib>:"Write Key.vi"("section"=w841, "error in (no error)"=w861, "value"=w829, "key"="启用5", "refnum"=w860) -> ("error out"=w830:errorcluster, "refnum out"=w831:T9)  [unwired: 4 in, 1 out]
        n487 = local read "选用水样"() -> (w848:enum16{"葡萄糖", "草酸钠"})
        n488 = call-poly <vilib>:"Write Key.vi"("section"="标线选择", "error in (no error)"=w830, "value"=w848, "key"="选用水样", "refnum"=w831) -> ("error out"=w845:errorcluster, "refnum out"=w846:T9)  [unwired: 4 in, 1 out]
        n489 = call <vilib>:"Close Config Data.vi"("error in (no error)"=w845, "refnum"=w846) -> ()  [unwired: 8 in, 2 out]
      }
      event "读取": Value Change {
        n490 = event-data() -> ()  [unwired: 1 in, 6 out]
        n491 = local write "枚举"(enum16{"读取数据", "写入数据", "读取写入DATABASE", "读取参数"}."读取参数" ("枚举")) -> ()
        n492 = Bundle By Name(cluster=T4 {"starting address"=0, "number of holding registers"=0}, "starting address"=u16 4616, "number of holding registers"=u16 94) -> (w916:T4)
        n493 = Flush Queue(queue=w909, error in (no error)=w908) -> (queue out=w912:refnum<queue>, error out=w911:errorcluster)  [unwired: 1 out]
        n494 = Enqueue Element(queue=w912, element=w916, error in (no error)=w911) -> ()  [unwired: 1 in, 3 out]
        "读取KB值" <- TRUE
      }
      event "写入": Mouse Down {
        n495 = event-data() -> ()  [unwired: 1 in, 8 out]
        n496 = flat-sequence {
          tunnel: w917 -> [w920]
          frame #0 {
            n497 = local read "模型"() -> (w918:enum32{"线性", "多项式"})
            n498 = case shown="\"线性\", 默认" w918 {
              tunnel: [w932 w973] -> w922
              tunnel: w920 -> [w926 w972]
              tunnel: [w926 w972] -> w919
              frame "线性", Default {
                n499 = local read "测量模式(公式)"() -> (w924:u16)
                n500 = local read "K"() -> (w929:dbl)
                n501 = local read "b"() -> (w928:dbl)
                n502 = case shown="7" w924 {
                  tunnel: [u16 4626 ("starting address") w935 w940 w945 w950 w955 w960 w965] -> w923
                  frame 0, Default {
                  }
                  frame 1 {
                    n503 = local read "量程选择"() -> (w934:enum16{"低量程", "高量程", "0-2量程"})
                    n504 = case shown="\"0-2量程\"" w934 {
                      tunnel: [u16 4626 ("starting address") u16 4632 ("starting address") u16 4638 ("starting address")] -> w935
                      frame "低量程", Default {
                      }
                      frame "高量程" {
                      }
                      frame "0-2量程" {
                      }
                    }
                  }
                  frame 2 {
                    n505 = local read "量程选择"() -> (w939:enum16{"低量程", "高量程", "0-2量程"})
                    n506 = case shown="\"低量程\", 默认" w939 {
                      tunnel: [u16 4638 ("starting address") u16 4644 ("starting address") u16 4638 ("starting address")] -> w940
                      frame "低量程", Default {
                      }
                      frame "高量程" {
                      }
                      frame "0-2量程" {
                      }
                    }
                  }
                  frame 3 {
                    n507 = local read "量程选择"() -> (w944:enum16{"低量程", "高量程", "0-2量程"})
                    n508 = case shown="\"低量程\", 默认" w944 {
                      tunnel: [u16 4650 ("starting address") u16 4656 ("starting address") u16 4638 ("starting address")] -> w945
                      frame "低量程", Default {
                      }
                      frame "高量程" {
                      }
                      frame "0-2量程" {
                      }
                    }
                  }
                  frame 4 {
                    n509 = local read "量程选择"() -> (w949:enum16{"低量程", "高量程", "0-2量程"})
                    n510 = case shown="\"低量程\", 默认" w949 {
                      tunnel: [u16 4662 ("starting address") u16 4668 ("starting address") u16 4638 ("starting address")] -> w950
                      frame "低量程", Default {
                      }
                      frame "高量程" {
                      }
                      frame "0-2量程" {
                      }
                    }
                  }
                  frame 5 {
                    n511 = local read "量程选择"() -> (w954:enum16{"低量程", "高量程", "0-2量程"})
                    n512 = case shown="\"低量程\", 默认" w954 {
                      tunnel: [u16 4674 ("starting address") u16 4680 ("starting address") u16 4638 ("starting address")] -> w955
                      frame "低量程", Default {
                      }
                      frame "高量程" {
                      }
                      frame "0-2量程" {
                      }
                    }
                  }
                  frame 6 {
                    n513 = local read "量程选择"() -> (w959:enum16{"低量程", "高量程", "0-2量程"})
                    n514 = case shown="\"低量程\", 默认" w959 {
                      tunnel: [u16 4686 ("starting address") u16 4692 ("starting address") u16 4638 ("starting address")] -> w960
                      frame "低量程", Default {
                      }
                      frame "高量程" {
                      }
                      frame "0-2量程" {
                      }
                    }
                  }
                  frame 7 {
                    n515 = local read "量程选择"() -> (w964:enum16{"低量程", "高量程", "0-2量程"})
                    n516 = case shown="\"低量程\", 默认" w964 {
                      tunnel: [u16 4698 ("starting address") u16 4704 ("starting address") u16 4638 ("starting address")] -> w965
                      frame "低量程", Default {
                      }
                      frame "高量程" {
                      }
                      frame "0-2量程" {
                      }
                    }
                  }
                }
                n517 = Build Array(w929, w928, 0.0 ("元素")) -> (w927:dbl[])
                n518 = call "浮点转CDAB整形cod.vi"("浮点数"=w927) -> ("CDAB整形输出"=w930:u16[])  [unwired: 10 in]
                n519 = Bundle By Name(cluster=cluster{"starting address":u16, "values":u16[]} {"starting address"=4272, "values"=[]}, "starting address"=w923, "values"=w930) -> (w932:cluster{"starting address":u16, "values":u16[]})
              }
              frame "多项式" {
                # "b,k,c"
                n520 = local read "测量模式(公式)"() -> (w970:u16)
                n521 = local read "多项式系数1"() -> (w979:dbl[])
                n522 = Index Array(array=w979) -> (element #1=w975:dbl, element #2=w976:dbl, element #3=w971:dbl)  [unwired: 3 in]
                n523 = case shown="7" w970 {
                  tunnel: [u16 4626 ("starting address") w982 w987 w992 w997 w1002 w1007 w1012] -> w969
                  frame 0, Default {
                  }
                  frame 1 {
                    n524 = local read "量程选择"() -> (w981:enum16{"低量程", "高量程", "0-2量程"})
                    n525 = case shown="\"0-2量程\"" w981 {
                      tunnel: [u16 4626 ("starting address") u16 4632 ("starting address") u16 4638 ("starting address")] -> w982
                      frame "低量程", Default {
                      }
                      frame "高量程" {
                      }
                      frame "0-2量程" {
                      }
                    }
                  }
                  frame 2 {
                    n526 = local read "量程选择"() -> (w986:enum16{"低量程", "高量程", "0-2量程"})
                    n527 = case shown="\"低量程\", 默认" w986 {
                      tunnel: [u16 4638 ("starting address") u16 4644 ("starting address") u16 4638 ("starting address")] -> w987
                      frame "低量程", Default {
                      }
                      frame "高量程" {
                      }
                      frame "0-2量程" {
                      }
                    }
                  }
                  frame 3 {
                    n528 = local read "量程选择"() -> (w991:enum16{"低量程", "高量程", "0-2量程"})
                    n529 = case shown="\"低量程\", 默认" w991 {
                      tunnel: [u16 4650 ("starting address") u16 4656 ("starting address") u16 4638 ("starting address")] -> w992
                      frame "低量程", Default {
                      }
                      frame "高量程" {
                      }
                      frame "0-2量程" {
                      }
                    }
                  }
                  frame 4 {
                    n530 = local read "量程选择"() -> (w996:enum16{"低量程", "高量程", "0-2量程"})
                    n531 = case shown="\"低量程\", 默认" w996 {
                      tunnel: [u16 4662 ("starting address") u16 4668 ("starting address") u16 4638 ("starting address")] -> w997
                      frame "低量程", Default {
                      }
                      frame "高量程" {
                      }
                      frame "0-2量程" {
                      }
                    }
                  }
                  frame 5 {
                    n532 = local read "量程选择"() -> (w1001:enum16{"低量程", "高量程", "0-2量程"})
                    n533 = case shown="\"低量程\", 默认" w1001 {
                      tunnel: [u16 4674 ("starting address") u16 4680 ("starting address") u16 4638 ("starting address")] -> w1002
                      frame "低量程", Default {
                      }
                      frame "高量程" {
                      }
                      frame "0-2量程" {
                      }
                    }
                  }
                  frame 6 {
                    n534 = local read "量程选择"() -> (w1006:enum16{"低量程", "高量程", "0-2量程"})
                    n535 = case shown="\"低量程\", 默认" w1006 {
                      tunnel: [u16 4686 ("starting address") u16 4692 ("starting address") u16 4638 ("starting address")] -> w1007
                      frame "低量程", Default {
                      }
                      frame "高量程" {
                      }
                      frame "0-2量程" {
                      }
                    }
                  }
                  frame 7 {
                    n536 = local read "量程选择"() -> (w1011:enum16{"低量程", "高量程", "0-2量程"})
                    n537 = case shown="\"低量程\", 默认" w1011 {
                      tunnel: [u16 4698 ("starting address") u16 4704 ("starting address") u16 4638 ("starting address")] -> w1012
                      frame "低量程", Default {
                      }
                      frame "高量程" {
                      }
                      frame "0-2量程" {
                      }
                    }
                  }
                }
                n538 = Build Array(w976, w975, w971) -> (w978:dbl[])
                n539 = call "浮点转CDAB整形cod.vi"("浮点数"=w978) -> ("CDAB整形输出"=w977:u16[])  [unwired: 10 in]
                n540 = Bundle By Name(cluster=cluster{"starting address":u16, "values":u16[]} {"starting address"=4272, "values"=[]}, "starting address"=w969, "values"=w977) -> (w973:cluster{"starting address":u16, "values":u16[]})
              }
            }
            n541 = Enqueue Element(queue=w919, element=w922, timeout in ms (-1)=1000 ("超时毫秒(-1)")) -> ()  [unwired: 1 in, 3 out]
          }
          frame #1 {
            n542 = local write "枚举"(enum16{"读取数据", "写入数据", "读取写入DATABASE", "读取参数"}."写入数据" ("枚举")) -> ()
          }
        }
      }
      event "一键写入": Value Change {
        n543 = event-data() -> ()  [unwired: 1 in, 6 out]
        n544 = flat-sequence {
          tunnel: w1017 -> [w1019]
          frame #0 {
            n545 = local read "模型"() -> (w1018:enum32{"线性", "多项式"})
            n546 = case shown="\"多项式\"" w1018 {
              tunnel: w1019 -> [w1020 w1074]
              frame "线性", Default {
                n547 = property on="测量模式(公式)" class="Ring (严格)"() -> ("NumItems"=w1021:u32)  [unwired: 2 in, 2 out]
                n548 = for {
                  N: w1021 -> [_]
                  tunnel: w1020 -> [w1029]
                  i -> [w1025]
                  n549 = Increment(x=w1025) -> (x+1=w1026:i32)
                  n550 = case shown="7" w1026 {
                    tunnel: [u16 4626 ("starting address") w1039 w1044 w1049 w1054 w1059 w1064 w1069] -> w1022
                    frame 0, Default {
                    }
                    frame 1 {
                      n551 = local read "量程选择"() -> (w1038:enum16{"低量程", "高量程", "0-2量程"})
                      n552 = case shown="\"低量程\", 默认" w1038 {
                        tunnel: [u16 4626 ("starting address") u16 4632 ("starting address") u16 4638 ("starting address")] -> w1039
                        frame "低量程", Default {
                        }
                        frame "高量程" {
                        }
                        frame "0-2量程" {
                        }
                      }
                    }
                    frame 2 {
                      n553 = local read "量程选择"() -> (w1043:enum16{"低量程", "高量程", "0-2量程"})
                      n554 = case shown="\"低量程\", 默认" w1043 {
                        tunnel: [u16 4638 ("starting address") u16 4644 ("starting address") u16 4638 ("starting address")] -> w1044
                        frame "低量程", Default {
                        }
                        frame "高量程" {
                        }
                        frame "0-2量程" {
                        }
                      }
                    }
                    frame 3 {
                      n555 = local read "量程选择"() -> (w1048:enum16{"低量程", "高量程", "0-2量程"})
                      n556 = case shown="\"低量程\", 默认" w1048 {
                        tunnel: [u16 4650 ("starting address") u16 4656 ("starting address") u16 4638 ("starting address")] -> w1049
                        frame "低量程", Default {
                        }
                        frame "高量程" {
                        }
                        frame "0-2量程" {
                        }
                      }
                    }
                    frame 4 {
                      n557 = local read "量程选择"() -> (w1053:enum16{"低量程", "高量程", "0-2量程"})
                      n558 = case shown="\"高量程\"" w1053 {
                        tunnel: [u16 4662 ("starting address") u16 4668 ("starting address") u16 4638 ("starting address")] -> w1054
                        frame "低量程", Default {
                        }
                        frame "高量程" {
                        }
                        frame "0-2量程" {
                        }
                      }
                    }
                    frame 5 {
                      n559 = local read "量程选择"() -> (w1058:enum16{"低量程", "高量程", "0-2量程"})
                      n560 = case shown="\"低量程\", 默认" w1058 {
                        tunnel: [u16 4674 ("starting address") u16 4680 ("starting address") u16 4638 ("starting address")] -> w1059
                        frame "低量程", Default {
                        }
                        frame "高量程" {
                        }
                        frame "0-2量程" {
                        }
                      }
                    }
                    frame 6 {
                      n561 = local read "量程选择"() -> (w1063:enum16{"低量程", "高量程", "0-2量程"})
                      n562 = case shown="\"低量程\", 默认" w1063 {
                        tunnel: [u16 4686 ("starting address") u16 4692 ("starting address") u16 4638 ("starting address")] -> w1064
                        frame "低量程", Default {
                        }
                        frame "高量程" {
                        }
                        frame "0-2量程" {
                        }
                      }
                    }
                    frame 7 {
                      n563 = local read "量程选择"() -> (w1068:enum16{"低量程", "高量程", "0-2量程"})
                      n564 = case shown="\"高量程\"" w1068 {
                        tunnel: [u16 4698 ("starting address") u16 4704 ("starting address") u16 4638 ("starting address")] -> w1069
                        frame "低量程", Default {
                        }
                        frame "高量程" {
                        }
                        frame "0-2量程" {
                        }
                      }
                    }
                  }
                  n565 = local read "K"() -> (w1033:dbl)
                  n566 = local read "b"() -> (w1034:dbl)
                  n567 = Build Array(w1033, w1034, 0.0 ("元素")) -> (w1035:dbl[])
                  n568 = call "浮点转CDAB整形cod.vi"("浮点数"=w1035) -> ("CDAB整形输出"=w1024:u16[])  [unwired: 10 in]
                  n569 = Insert Into Array(array=u16[] [], index=0 ("索引"), new element=w1024) -> (w1023:u16[])
                  n570 = Bundle By Name(cluster=cluster{"starting address":u16, "values":u16[]} {"starting address"=4272, "values"=[]}, "starting address"=w1022, "values"=w1023) -> (w1030:cluster{"starting address":u16, "values":u16[]})
                  n571 = Enqueue Element(queue=w1029, element=w1030, timeout in ms (-1)=1000 ("超时毫秒(-1)")) -> ()  [unwired: 1 in, 3 out]
                }
              }
              frame "多项式" {
                n572 = property on="测量模式(公式)" class="Ring (严格)"() -> ("NumItems"=w1073:u32)  [unwired: 2 in, 2 out]
                n573 = for {
                  N: w1073 -> [_]
                  tunnel: w1074 -> [w1078]
                  i -> [w1077]
                  # "b,k,c"
                  n574 = local read "多项式系数1"() -> (w1090:dbl[])
                  n575 = Increment(x=w1077) -> (x+1=w1076:i32)
                  n576 = Index Array(array=w1090) -> (element #1=w1087:dbl, element #2=w1088:dbl, element #3=w1085:dbl)  [unwired: 3 in]
                  n577 = case shown="3" w1076 {
                    tunnel: [u16 4626 ("starting address") w1093 w1098 w1103 w1108 w1113 w1118 w1123] -> w1075
                    frame 0, Default {
                    }
                    frame 1 {
                      n578 = local read "量程选择"() -> (w1092:enum16{"低量程", "高量程", "0-2量程"})
                      n579 = case shown="\"0-2量程\"" w1092 {
                        tunnel: [u16 4626 ("starting address") u16 4632 ("starting address") u16 4638 ("starting address")] -> w1093
                        frame "低量程", Default {
                        }
                        frame "高量程" {
                        }
                        frame "0-2量程" {
                        }
                      }
                    }
                    frame 2 {
                      n580 = local read "量程选择"() -> (w1097:enum16{"低量程", "高量程", "0-2量程"})
                      n581 = case shown="\"低量程\", 默认" w1097 {
                        tunnel: [u16 4638 ("starting address") u16 4644 ("starting address") u16 4638 ("starting address")] -> w1098
                        frame "低量程", Default {
                        }
                        frame "高量程" {
                        }
                        frame "0-2量程" {
                        }
                      }
                    }
                    frame 3 {
                      n582 = local read "量程选择"() -> (w1102:enum16{"低量程", "高量程", "0-2量程"})
                      n583 = case shown="\"低量程\", 默认" w1102 {
                        tunnel: [u16 4650 ("starting address") u16 4656 ("starting address") u16 4638 ("starting address")] -> w1103
                        frame "低量程", Default {
                        }
                        frame "高量程" {
                        }
                        frame "0-2量程" {
                        }
                      }
                    }
                    frame 4 {
                      n584 = local read "量程选择"() -> (w1107:enum16{"低量程", "高量程", "0-2量程"})
                      n585 = case shown="\"低量程\", 默认" w1107 {
                        tunnel: [u16 4662 ("starting address") u16 4668 ("starting address") u16 4638 ("starting address")] -> w1108
                        frame "低量程", Default {
                        }
                        frame "高量程" {
                        }
                        frame "0-2量程" {
                        }
                      }
                    }
                    frame 5 {
                      n586 = local read "量程选择"() -> (w1112:enum16{"低量程", "高量程", "0-2量程"})
                      n587 = case shown="\"低量程\", 默认" w1112 {
                        tunnel: [u16 4674 ("starting address") u16 4680 ("starting address") u16 4638 ("starting address")] -> w1113
                        frame "低量程", Default {
                        }
                        frame "高量程" {
                        }
                        frame "0-2量程" {
                        }
                      }
                    }
                    frame 6 {
                      n588 = local read "量程选择"() -> (w1117:enum16{"低量程", "高量程", "0-2量程"})
                      n589 = case shown="\"低量程\", 默认" w1117 {
                        tunnel: [u16 4686 ("starting address") u16 4692 ("starting address") u16 4638 ("starting address")] -> w1118
                        frame "低量程", Default {
                        }
                        frame "高量程" {
                        }
                        frame "0-2量程" {
                        }
                      }
                    }
                    frame 7 {
                      n590 = local read "量程选择"() -> (w1122:enum16{"低量程", "高量程", "0-2量程"})
                      n591 = case shown="\"低量程\", 默认" w1122 {
                        tunnel: [u16 4698 ("starting address") u16 4704 ("starting address") u16 4638 ("starting address")] -> w1123
                        frame "低量程", Default {
                        }
                        frame "高量程" {
                        }
                        frame "0-2量程" {
                        }
                      }
                    }
                  }
                  n592 = Build Array(w1088, w1087, w1085) -> (w1089:dbl[])
                  n593 = call "浮点转CDAB整形cod.vi"("浮点数"=w1089) -> ("CDAB整形输出"=w1082:u16[])  [unwired: 10 in]
                  n594 = Insert Into Array(array=u16[] [], index=0 ("索引"), new element=w1082) -> (w1081:u16[])
                  n595 = Bundle By Name(cluster=cluster{"starting address":u16, "values":u16[]} {"starting address"=4272, "values"=[]}, "starting address"=w1075, "values"=w1081) -> (w1079:cluster{"starting address":u16, "values":u16[]})
                  n596 = Enqueue Element(queue=w1078, element=w1079, timeout in ms (-1)=1000 ("超时毫秒(-1)")) -> ()  [unwired: 1 in, 3 out]
                }
              }
            }
          }
          frame #1 {
            n597 = local write "枚举"(enum16{"读取数据", "写入数据", "读取写入DATABASE", "读取参数"}."写入数据" ("枚举")) -> ()
          }
        }
      }
      event "滴定曲线": Value Change {
        n598 = event-data() -> ()  [unwired: 1 in, 6 out]
        n599 = property on="窗格" class="Pane"("Origin"=T10 {"Horizontal"=0, "Vertical"=3200} ("原点")) -> ()  [unwired: 2 in, 2 out]
      }
      event "历史波形": Value Change {
        n600 = event-data() -> ()  [unwired: 1 in, 6 out]
        n601 = call-poly <vilib>:"Read Waveforms from File.vi"() -> ("error out"=w1129:errorcluster, "first waveform in record"=w1130:waveform(dbl))  [unwired: 6 in, 2 out]
        n602 = case shown="无错误" w1129 {
          tunnel: w1130 -> [w1133 _]
          frame No Error {
            n603 = Unbundle By Name(w1133) -> ("t0"=→"波形时间":timestamp, "Y"=w1132:dbl[])  [unwired: 2 out]
            n604 = local write "ORP滴定曲线2"(w1132) -> ()
            n605 = local write "滴定数-ORP值"(w1132) -> ()
          }
          frame Error {
            n606 = One Button Dialog(message="打开失败" ("消息")) -> ()  [unwired: 1 in, 1 out]
          }
        }
      }
      event "数据查询": Value Change {
        n607 = event-data() -> ()  [unwired: 1 in, 6 out]
        n608 = call "数据查询_仪器数据.vi"() -> ()  [unwired: 12 in]
      }
      event Panel Close {
        n609 = event-data() -> ()  [unwired: 1 in, 4 out]
        n610 = Quit LabVIEW(quit? (T)=TRUE ("退出？(T)")) -> ()
      }
    }
  }
  n611 = while {
    stop <- FALSE stop-if-true
    n612 = event shown="[30] \"低量程稀释倍数:\": 鼠标按下" {
      selector: _ -> [_ _ _ _ _ _ _ _ _ _ _ _ _ _ _ _ _ _ _ _ _ _ _ _ _ _ _ _ _ _ _]
      dyn-events: _ -> [_ _ _ _ _ _ _ _ _ _ _ _ _ _ _ _ _ _ _ _ _ _ _ _ _ _ _ _ _ _ _]
      timeout: _ -> [_ _ _ _ _ _ _ _ _ _ _ _ _ _ _ _ _ _ _ _ _ _ _ _ _ _ _ _ _ _ _]
      event Timeout {
        n613 = event-data() -> ()  [unwired: 1 in, 3 out]
      }
      event "温度": Mouse Down {
        n614 = event-data() -> ()  [unwired: 1 in, 8 out]
        n615 = local read "温度"() -> (w1138:dbl)
        n616 = call "数字键盘.vi"("OldNumber"=w1138) -> ("NewNumber"=w1137:sgl)
        n617 = local write "温度"(w1137) -> ()
      }
      event "恒温时间": Mouse Down {
        n618 = event-data() -> ()  [unwired: 1 in, 8 out]
        n619 = local read "恒温时间"() -> (w1139:dbl)
        n620 = call "数字键盘.vi"("OldNumber"=w1139) -> ("NewNumber"=w1140:sgl)
        n621 = local write "恒温时间"(w1140) -> ()
      }
      event "浓度 2": Mouse Down {
        n622 = event-data() -> ()  [unwired: 1 in, 8 out]
        n623 = local read "浓度 2"() -> (w1142:dbl)
        n624 = call "数字键盘.vi"("OldNumber"=w1142) -> ("NewNumber"=w1141:sgl)
        n625 = local write "浓度 2"(w1141) -> ()
      }
      event "修正系数 2": Mouse Down {
        n626 = event-data() -> ()  [unwired: 1 in, 8 out]
        n627 = local read "修正系数 2"() -> (w1143:dbl)
        n628 = call "数字键盘.vi"("OldNumber"=w1143) -> ("NewNumber"=w1144:sgl)
        n629 = local write "修正系数 2"(w1144) -> ()
      }
      event "水样": Mouse Down {
        n630 = event-data() -> ()  [unwired: 1 in, 8 out]
        n631 = local read "水样"() -> (w1145:dbl)
        n632 = call "数字键盘.vi"("OldNumber"=w1145) -> ("NewNumber"=w1146:sgl)
        n633 = local write "水样"(w1146) -> ()
      }
      event "蒸馏水": Mouse Down {
        n634 = event-data() -> ()  [unwired: 1 in, 8 out]
        n635 = local read "蒸馏水"() -> (w1147:dbl)
        n636 = call "数字键盘.vi"("OldNumber"=w1147) -> ("NewNumber"=w1148:sgl)
        n637 = local write "蒸馏水"(w1148) -> ()
      }
      event "标液": Mouse Down {
        n638 = event-data() -> ()  [unwired: 1 in, 8 out]
        n639 = local read "标液"() -> (w1149:dbl)
        n640 = call "数字键盘.vi"("OldNumber"=w1149) -> ("NewNumber"=w1150:sgl)
        n641 = local write "标液"(w1150) -> ()
      }
      event "质控样": Mouse Down {
        n642 = event-data() -> ()  [unwired: 1 in, 8 out]
        n643 = local read "质控样"() -> (w1151:dbl)
        n644 = call "数字键盘.vi"("OldNumber"=w1151) -> ("NewNumber"=w1152:sgl)
        n645 = local write "质控样"(w1152) -> ()
      }
      event "加标回收": Mouse Down {
        n646 = event-data() -> ()  [unwired: 1 in, 8 out]
        n647 = local read "加标回收"() -> (w1153:dbl)
        n648 = call "数字键盘.vi"("OldNumber"=w1153) -> ("NewNumber"=w1154:sgl)
        n649 = local write "加标回收"(w1154) -> ()
      }
      event "草酸钠": Mouse Down {
        n650 = event-data() -> ()  [unwired: 1 in, 8 out]
        n651 = local read "草酸钠"() -> (w1155:dbl)
        n652 = call "数字键盘.vi"("OldNumber"=w1155) -> ("NewNumber"=w1156:sgl)
        n653 = local write "草酸钠"(w1156) -> ()
      }
      event "高锰酸钾": Mouse Down {
        n654 = event-data() -> ()  [unwired: 1 in, 8 out]
        n655 = local read "高锰酸钾"() -> (w1157:dbl)
        n656 = call "数字键盘.vi"("OldNumber"=w1157) -> ("NewNumber"=w1158:sgl)
        n657 = local write "高锰酸钾"(w1158) -> ()
      }
      event "硫酸": Mouse Down {
        n658 = event-data() -> ()  [unwired: 1 in, 8 out]
        n659 = local read "硫酸"() -> (w1159:dbl)
        n660 = call "数字键盘.vi"("OldNumber"=w1159) -> ("NewNumber"=w1160:sgl)
        n661 = local write "硫酸"(w1160) -> ()
      }
      event "零点泵计量数 2": Mouse Down {
        n662 = event-data() -> ()  [unwired: 1 in, 8 out]
        n663 = local read "零点泵计量数 2"() -> (w1161:dbl)
        n664 = call "数字键盘.vi"("OldNumber"=w1161) -> ("NewNumber"=w1162:sgl)
        n665 = local write "零点泵计量数 2"(w1162) -> ()
      }
      event "标度泵计量数 2": Mouse Down {
        n666 = event-data() -> ()  [unwired: 1 in, 8 out]
        n667 = local read "标度泵计量数 2"() -> (w1163:dbl)
        n668 = call "数字键盘.vi"("OldNumber"=w1163) -> ("NewNumber"=w1164:sgl)
        n669 = local write "标度泵计量数 2"(w1164) -> ()
      }
      event "标样浓度 2": Mouse Down {
        n670 = event-data() -> ()  [unwired: 1 in, 8 out]
        n671 = local read "标样浓度 2"() -> (w1165:dbl)
        n672 = call "数字键盘.vi"("OldNumber"=w1165) -> ("NewNumber"=w1166:sgl)
        n673 = local write "标样浓度 2"(w1166) -> ()
      }
      event "浓度1": Mouse Down {
        n674 = event-data() -> ()  [unwired: 1 in, 8 out]
        n675 = local read "浓度1"() -> (w1168:dbl)
        n676 = call "数字键盘.vi"("OldNumber"=w1168) -> ("NewNumber"=w1167:sgl)
        n677 = property on="浓度1" class="DigNum (严格)"("Val(Sgnl)"=w1167) -> ()  [unwired: 2 in, 2 out]
      }
      event "浓度2": Mouse Down {
        n678 = event-data() -> ()  [unwired: 1 in, 8 out]
        n679 = local read "浓度2"() -> (w1170:dbl)
        n680 = call "数字键盘.vi"("OldNumber"=w1170) -> ("NewNumber"=w1169:sgl)
        n681 = property on="浓度2" class="DigNum (严格)"("Val(Sgnl)"=w1169) -> ()  [unwired: 2 in, 2 out]
      }
      event "浓度3": Mouse Down {
        n682 = event-data() -> ()  [unwired: 1 in, 8 out]
        n683 = local read "浓度3"() -> (w1172:dbl)
        n684 = call "数字键盘.vi"("OldNumber"=w1172) -> ("NewNumber"=w1171:sgl)
        n685 = property on="浓度3" class="DigNum (严格)"("Val(Sgnl)"=w1171) -> ()  [unwired: 2 in, 2 out]
      }
      event "浓度4": Mouse Down {
        n686 = event-data() -> ()  [unwired: 1 in, 8 out]
        n687 = local read "浓度4"() -> (w1174:dbl)
        n688 = call "数字键盘.vi"("OldNumber"=w1174) -> ("NewNumber"=w1173:sgl)
        n689 = property on="浓度4" class="DigNum (严格)"("Val(Sgnl)"=w1173) -> ()  [unwired: 2 in, 2 out]
      }
      event "浓度5": Mouse Down {
        n690 = event-data() -> ()  [unwired: 1 in, 8 out]
        n691 = local read "浓度5"() -> (w1176:dbl)
        n692 = call "数字键盘.vi"("OldNumber"=w1176) -> ("NewNumber"=w1175:sgl)
        n693 = property on="浓度5" class="DigNum (严格)"("Val(Sgnl)"=w1175) -> ()  [unwired: 2 in, 2 out]
      }
      event "跨度液浓度": Mouse Down {
        n694 = event-data() -> ()  [unwired: 1 in, 8 out]
        n695 = local read "跨度液浓度"() -> (w1178:dbl)
        n696 = call "数字键盘.vi"("OldNumber"=w1178) -> ("NewNumber"=w1177:sgl)
        n697 = property on="跨度液浓度" class="DigNum (严格)"("Val(Sgnl)"=w1177) -> ()  [unwired: 2 in, 2 out]
      }
      event "跨度液浓度": Value Change {
        n698 = event-data() -> ()  [unwired: 1 in, 6 out]
        n699 = call <vilib>:"Application Directory.vi"() -> ("Application Directory"=w1182:path)
        n700 = Build Path(base path=w1182, name or relative path="data\\Set.ini" ("名称或相对路径")) -> (appended path=w1184:path)
        n701 = local read "跨度液浓度"() -> (w1179:dbl)
        n702 = call <vilib>:"Open Config Data.vi"("configuration file path"=w1184) -> ("error out"=w1186:errorcluster, "refnum"=w1185:T9)  [unwired: 8 in, 1 out]
        n703 = call-poly <vilib>:"Write Key.vi"("section"="CODMn参数" ("key"), "error in (no error)"=w1186, "value"=w1179, "key"="跨度液浓度", "refnum"=w1185) -> ("error out"=w1188:errorcluster, "refnum out"=w1187:T9)  [unwired: 4 in, 1 out]
        n704 = call <vilib>:"Close Config Data.vi"("error in (no error)"=w1188, "refnum"=w1187) -> ()  [unwired: 8 in, 2 out]
      }
      event "泵滴定数1": Mouse Down {
        n705 = event-data() -> ()  [unwired: 1 in, 8 out]
        n706 = local read "泵滴定数1"() -> (w1190:dbl)
        n707 = call "数字键盘.vi"("OldNumber"=w1190) -> ("NewNumber"=w1189:sgl)
        n708 = property on="泵滴定数1" class="DigNum (严格)"("Val(Sgnl)"=w1189) -> ()  [unwired: 2 in, 2 out]
      }
      event "泵滴定数2": Mouse Down {
        n709 = event-data() -> ()  [unwired: 1 in, 8 out]
        n710 = local read "泵滴定数2"() -> (w1192:dbl)
        n711 = call "数字键盘.vi"("OldNumber"=w1192) -> ("NewNumber"=w1191:sgl)
        n712 = property on="泵滴定数2" class="DigNum (严格)"("Val(Sgnl)"=w1191) -> ()  [unwired: 2 in, 2 out]
      }
      event "泵滴定数3": Mouse Down {
        n713 = event-data() -> ()  [unwired: 1 in, 8 out]
        n714 = local read "泵滴定数3"() -> (w1194:dbl)
        n715 = call "数字键盘.vi"("OldNumber"=w1194) -> ("NewNumber"=w1193:sgl)
        n716 = property on="泵滴定数3" class="DigNum (严格)"("Val(Sgnl)"=w1193) -> ()  [unwired: 2 in, 2 out]
      }
      event "泵滴定数4": Mouse Down {
        n717 = event-data() -> ()  [unwired: 1 in, 8 out]
        n718 = local read "泵滴定数4"() -> (w1196:dbl)
        n719 = call "数字键盘.vi"("OldNumber"=w1196) -> ("NewNumber"=w1195:sgl)
        n720 = property on="泵滴定数4" class="DigNum (严格)"("Val(Sgnl)"=w1195) -> ()  [unwired: 2 in, 2 out]
      }
      event "泵滴定数5": Mouse Down {
        n721 = event-data() -> ()  [unwired: 1 in, 8 out]
        n722 = local read "泵滴定数5"() -> (w1198:dbl)
        n723 = call "数字键盘.vi"("OldNumber"=w1198) -> ("NewNumber"=w1197:sgl)
        n724 = property on="泵滴定数5" class="DigNum (严格)"("Val(Sgnl)"=w1197) -> ()  [unwired: 2 in, 2 out]
      }
      event "低切高阈值", "高切低阈值": Mouse Down {
        n725 = event-data() -> ("CtlRef"=w1202:refnum<vi>)  [unwired: 1 in, 7 out]
        n726 = property class="DigNum (严格)"(reference=w1202) -> (reference out=w1200:refnum<vi>, "Value"=w1201:dbl)  [unwired: 1 in, 1 out]
        n727 = call "数字键盘.vi"("OldNumber"=w1201) -> ("NewNumber"=w1199:sgl)
        n728 = property class="DigNum (严格)"(reference=w1200, "Val(Sgnl)"=w1199) -> ()  [unwired: 1 in, 2 out]
      }
      event "高量程稀释倍数:": Mouse Down {
        n729 = event-data() -> ()  [unwired: 1 in, 8 out]
        n730 = local read "高量程稀释倍数:"() -> (w1204:i8)
        n731 = call "数字键盘.vi"("OldNumber"=w1204) -> ("NewNumber"=w1203:sgl)
        n732 = local write "高量程稀释倍数:"(w1203) -> ()
      }
      event "低量程稀释倍数:": Mouse Down {
        n733 = event-data() -> ()  [unwired: 1 in, 8 out]
        n734 = local read "低量程稀释倍数:"() -> (w1206:i8)
        n735 = call "数字键盘.vi"("OldNumber"=w1206) -> ("NewNumber"=w1205:sgl)
        n736 = local write "低量程稀释倍数:"(w1205) -> ()
      }
    }
  }
  n737 = while {
    tunnel: w44 -> [w1346]
    tunnel: w43 -> [w1345]
    tunnel: w34 -> [w1341]
    tunnel: w33 -> [w1340]
    stop <- FALSE stop-if-true
    w1266 = T15 0 items=["最小二乘", "最小绝对残差", "Bisquare"] ("method")
    n738 = local read "浓度5"() -> (w1246:dbl)
    n739 = local read "浓度4"() -> (w1247:dbl)
    n740 = local read "浓度2"() -> (w1279:dbl)
    n741 = local read "浓度3"() -> (w1280:dbl)
    n742 = local read "浓度1"() -> (w1278:dbl)
    n743 = local read "低量程稀释倍数:"() -> (w1212:i8)
    n744 = local read "启用4"() -> (w1243:bool)
    n745 = local read "泵滴定数3"() -> (w1283:dbl)
    n746 = local read "启用3"() -> (w1286:bool)
    n747 = local read "启用5"() -> (w1242:bool)
    n748 = local read "泵滴定数2"() -> (w1282:dbl)
    n749 = local read "泵滴定数4"() -> (w1245:dbl)
    n750 = local read "泵滴定数5"() -> (w1244:dbl)
    n751 = local read "启用2"() -> (w1285:bool)
    n752 = local read "泵滴定数1"() -> (w1281:dbl)
    n753 = local read "启用1"() -> (w1284:bool)
    n754 = local read "高量程稀释倍数:"() -> (w1210:i8)
    n755 = local read "自动切换量程"() -> (w1241:bool)
    n756 = Wait (ms)(milliseconds to wait=u32 500 ("等待时间（毫秒）")) -> ()  [unwired: 1 out]
    n757 = Build Array(w1284, w1285, w1286, w1243, w1242) -> (w1267:bool[])
    n758 = global read "CODMn断电保存全局变量.vi" "测量模式(公式)"() -> (w1207:u16)
    n759 = Build Array(w1278, w1279, w1280, w1247, w1246) -> (w1269:dbl[])
    n760 = Build Array(w1281, w1282, w1283, w1245, w1244) -> (w1268:dbl[])
    n761 = Bundle By Name(cluster=T4 {"starting address"=4224, "number of holding registers"=16}, "starting address"=u16 4224, "number of holding registers"=u16 50) -> (w1389:T4)
    n762 = local read "基本量程"() -> (w1249:enum16{"L", "H"})
    n763 = Select(t=T11."Enabled" ("禁用"), s=w1241, f=T11."Disabled and Grayed Out" ("禁用")) -> (s? t:f=w1238:T11)
    n764 = Multiply(x=w1210, y=i8 8) -> (x*y=w1213:i8)
    n765 = Multiply(x=w1212, y=i8 8) -> (x*y=w1214:i8)
    n766 = Multiply(x="浓度 2", y=100.0) -> (x*y=w1321:dbl)
    n767 = property on="高切低阈值" class="DigNum (严格)"("DisabledEnum"=w1238) -> ()  [unwired: 2 in, 2 out]
    n768 = Multiply(x="修正系数 2", y=100.0) -> (x*y=w1318:dbl)
    n769 = property on="低切高阈值" class="DigNum (严格)"("DisabledEnum"=w1238) -> ()  [unwired: 2 in, 2 out]
    n770 = call "线性公式CODMn用.vi"("标液浓度"=w1269, "监测浓度"=w1268, "启用"=w1267, "method"=w1266, "模型"="模型", "精度"=6) -> ("拟合方程"=→"拟合公式":string, "r^2"=→"r^2":dbl, "slope"=→"K":dbl, "intercept"=→"b":dbl, "XY图"=→"XY图":cluster{"X Values":dbl[], "Y Values":dbl[]}[], "Polynomial Coefficients"=→"多项式系数1":dbl[])  [unwired: 8 in]
    n771 = Multiply(x="温度", y=10.0) -> (x*y=w1324:dbl)
    n772 = Number To Decimal String(number=w1214) -> (decimal integer string=w1219:string)  [unwired: 1 in]
    n773 = Number To Decimal String(number=w1213) -> (decimal integer string=w1217:string)  [unwired: 1 in]
    n774 = local write "浓度"(w1321) -> ()
    n775 = local write "修正系数"(w1318) -> ()
    n776 = global write "COD浓度全局变量.vi" "基本量程"(w1249) -> ()
    n777 = local write "测量模式(公式)"(w1207) -> ()
    n778 = local write "温度 2"(w1324) -> ()
    n779 = global write "COD浓度全局变量.vi" "跨度液浓度"("跨度液浓度") -> ()
    n780 = Concatenate Strings("L低量程范围:0~" ("量程解释说明"), w1219, "(mg/L)\n\nH高量程范围:" ("量程解释说明"), "0" ("字符串"), "~" ("量程解释说明"), w1217, "(mg/L)" ("量程解释说明")) -> (→"稀释倍数解释":string)
    n781 = Enqueue Element(queue=w1346, element=w1389, error in (no error)=w1345) -> ()  [unwired: 1 in, 3 out]
    n782 = local read "Registers"() -> (w1258:u16[])
    n783 = To Word Integer(number=w1258) -> (16bit integer=w1257:i16[])
    n784 = Index Array(array=w1257, index #1=0 ("索引"), index #4=3 ("索引"), index #14=13 ("索引"), index #15=14 ("索引"), index #32=31 ("索引")) -> (element #1=w1315:i16, element #2=w1314:i16, element #3=w1313:i16, element #4=w1248:i16, element #5=→"模式（受控）":i16, element #6=→"进样管":i16, element #7=→"高锰酸钾":i16, element #8=→"草酸钠":i16, element #9=→"硫酸":i16, element #10=w1256:i16, element #11=w1373:i16, element #12=w1375:i16, element #13=w1223:i16, element #14=w1380:i16, element #15=w1348:i16, element #16=w1272:i16, element #33=→"分":i16, element #34=→"秒":i16)  [unwired: 29 in, 16 out]
    "多列列表框" <- w1272
    n785 = Decrement(x=w1223) -> (x-1=w1234:i16)
    n786 = Greater Than 0?(x=w1223) -> (x > 0?=→"故障标记":bool)
    n787 = Replace Array Subset(array=bool[] [FALSE, FALSE, FALSE, FALSE, FALSE, FALSE, FALSE, FALSE, FALSE, FALSE], new element=TRUE ("新元素/子数组"), index=w1234) -> (w1235:bool[])
    n788 = To Single Precision Float(number=w1256) -> (single precision float=→"ORP显示":sgl)
    n789 = Index Array(array=w1235) -> (element #1=w1233:bool, element #2=w1232:bool, element #3=w1231:bool, element #4=w1230:bool, element #5=w1229:bool, element #6=w1228:bool, element #7=w1227:bool, element #8=w1226:bool, element #9=w1225:bool, element #10=w1224:bool)  [unwired: 10 in]
    "ORP故障" <- w1233
    "温控器故障" <- w1232
    "加热故障" <- w1231
    "高锰酸钾报警" <- w1230
    "草酸钠报警" <- w1229
    "测量错误" <- w1228
    "校零错误" <- w1227
    "校标错误" <- w1226
    "进水样超量程" <- w1225
    "排液故障" <- w1224
    n790 = global write "COD测量模式全局.vi" "CODMn工作状态"(w1248) -> ()
    n791 = Build Array(w1315, w1314, w1313) -> (w1316:i16[])
    n792 = global write "运行时序全局变量.vi" "多列列表框"(w1272) -> ()
    n793 = Equal?(x=w1375, y=u16 1) -> (x = y?=→"排液标记":bool)
    n794 = Equal?(x=w1272, y=u16 5) -> (x = y?=w1344:bool)
    n795 = Divide(x=w1373, y=u16 10) -> (x/y=→"温度":dbl)
    n796 = Bundle By Name(cluster=T12 {"ORP故障"=FALSE, "温控器故障"=FALSE, "加热故障"=FALSE, "高锰酸钾报警"=FALSE, "草酸钠报警"=FALSE, "测量错误"=FALSE, "校零错误"=FALSE, "校标错误"=FALSE, " 进水样超量程"=FALSE, "排液阀故障"=FALSE} ("报警簇"), "ORP故障"=w1233, "温控器故障"=w1232, "加热故障"=w1231, "高锰酸钾报警"=w1230, "草酸钠报警"=w1229, "测量错误"=w1228, "校零错误"=w1227, "校标错误"=w1226, "进水样超量程"=w1225, "排液阀故障"=w1224) -> (w1332:T12)
    n797 = feedback #2(w1272) -> (w1331:i16)
    n798 = feedback-in #2(w1272) -> ()
    n799 = Equal?(x=w1248, y=u16 0) -> (x = y?=→"待机":bool)
    n800 = Divide(x=w1380, y=u16 1000) -> (x/y=→"零点滴定值":dbl)
    n801 = Equal?(x=w1248, y=u16 1) -> (x = y?=→"水样测量":bool)
    n802 = Divide(x=w1348, y=u16 1000) -> (x/y=→"标度滴定值":dbl)
    n803 = call <vilib>:"Boolean Crossing PtByPt.vi"("direction"=enum16{"either", "false-true", "true-false"}."false-true", "input"=w1344) -> ("crossing"=w1342:bool)  [unwired: 1 in]
    n804 = Equal?(x=w1248, y=u16 2) -> (x = y?=→"标样核查标记":bool)
    n805 = Equal?(x=w1248, y=u16 3) -> (x = y?=→"零点核查标记":bool)
    n806 = Equal?(x=w1248, y=u16 4) -> (x = y?=→"跨度核查标记":bool)
    n807 = Equal?(x=w1248, y=u16 5) -> (x = y?=→"空白测试标记":bool)
    n808 = Not Equal?(x=w1272, y=w1331) -> (x != y?=w1330:bool)
    n809 = call "CODMn报警信息.vi"("报警簇"=w1332) -> ("CODMN报警信息"=w1333:string)  [unwired: 10 in]
    n810 = Equal?(x=w1248, y=u16 6) -> (x = y?=→"平行样测量":bool)
    n811 = Equal?(x=w1248, y=u16 7) -> (x = y?=→"质控样测量":bool)
    n812 = Equal?(x=w1248, y=u16 8) -> (x = y?=→"校零标记":bool)
    n813 = Equal?(x=w1248, y=u16 9) -> (x = y?=→"校标标记":bool)
    n814 = Equal?(x=w1248, y=u16 10) -> (x = y?=→"加标回收测量":bool)
    n815 = case shown="真" w1342 {
      tunnel: w1341 -> [_ w1487]
      tunnel: w1340 -> [_ w1482]
      frame False {
      }
      frame True {
        n816 = Bundle By Name(cluster=T4 {"starting address"=0, "number of holding registers"=0}, "starting address"=u16 4101, "number of holding registers"=u16 10) -> (w1486:T4)
        n817 = Enqueue Element(queue=w1487, element=w1486, error in (no error)=w1482) -> ()  [unwired: 1 in, 3 out]
        n818 = local write "枚举"(enum16{"读取数据", "写入数据", "读取写入DATABASE", "读取参数"}."读取写入DATABASE" ("枚举")) -> ()
      }
    }
    n819 = case shown="真" w1330 {
      tunnel: w1272 -> [_ w1465]
      frame False {
      }
      frame True {
        n820 = property on="多列列表框" class="MCListbox (严格)"() -> ("ItemNames"=w1459:string[][])  [unwired: 2 in, 2 out]
        n821 = Index Array(array=w1459, index (row)=w1465) -> (element=w1456:string[])  [unwired: 1 in]
        n822 = Index Array(array=w1456, index=0 ("索引")) -> (element=w1454:string)
        n823 = Array To Spreadsheet String(delimiter (Tab)="-" ("分隔符(Tab)"), array=w1456, 3:"" ("格式字符串")) -> ()  [unwired: 1 out]
        n824 = Get Date/Time In Seconds() -> (seconds since 1Jan1904=w1463:timestamp)
        n825 = Bundle(cluster=T13 {"时间标识"=timestamp(0 s since 1904-01-01), "参数"="", "日志信息"="", "流程参数"=""} ("data in"), "时间标识"=w1463, "参数"="CODMn" ("table输入"), "日志信息"=w1454, "流程参数"="" ("table输入")) -> (w1460:T13)
        n826 = call "流程日志字段定义.vi"("table输入"="操作日志", "data in"=w1460) -> ("table输出"=w1468:string, "columns"=w1469:string[], "data out"=w1470:T16)  [unwired: 7 in]
        n827 = call "插入数据.vi"("data"=w1470, "columns"=w1469, "database"="database3.mdb", "table"=w1468) -> ()  [unwired: 7 in, 1 out]
      }
    }
    n828 = feedback #3(w1333) -> (w1334:string)
    n829 = feedback-in #3(w1333) -> ()
    n830 = Not Equal?(x=w1333, y="") -> (x != y?=w1338:bool)
    n831 = global read "COD读取DATA全局.vi" "data"() -> (w1294:T17)
    n832 = Less Or Equal?(x=w1272, y=u16 4) -> (x <= y?=w1276:bool)
    n833 = Not Equal?(x=w1333, y=w1334) -> (x != y?=w1335:bool)
    n834 = And(x=w1335, y=w1338) -> (x .and. y?=w1336:bool)
    n835 = global read "COD测量模式全局.vi" "测量模式"() -> (w1293:string)
    n836 = Unbundle By Name(w1294) -> ("时间"=w1291:timestamp, "检测值"=w1290:sgl, "数据标识"=w1289:string)
    n837 = case shown="真" w1276 {
      frame False {
      }
      frame True {
        n838 = local read "跨度核查标记"() -> (w1397:bool)
        n839 = local read "空白测试标记"() -> (w1396:bool)
        n840 = local read "加标回收测量"() -> (w1395:bool)
        n841 = local read "标样核查标记"() -> (w1402:bool)
        n842 = local read "零点核查标记"() -> (w1401:bool)
        n843 = local read "平行样测量"() -> (w1394:bool)
        n844 = local read "校零标记"() -> (w1393:bool)
        n845 = local read "校标标记"() -> (w1392:bool)
        n846 = local read "水样测量"() -> (w1403:bool)
        n847 = local read "测量模式数字"() -> (w1399:i32)
        n848 = local read "启动时间"() -> (w1391:timestamp)
        n849 = Build Array(w1403, w1402, w1401, w1397, w1396, w1395, w1394, w1393, w1392) -> (w1400:bool[])
        n850 = case shown="0, 默认" w1399 {
          tunnel: ["水样测试" ("测量模式") "标样核查" ("测量模式") "零点核查" ("测量模式") "跨度核查" ("测量模式") "空白测试" ("测量模式") "加标回收" ("测量模式") "平行样" ("测量模式") "校零" ("测量模式") "校标" ("测量模式")] -> w1398
          tunnel: w1391 -> [w1404 _ _ _ _ w1410 _ _ _]
          frame 0, Default {
            n851 = global write "COD测量模式全局.vi" "水样启动时间"(w1404) -> ()
          }
          frame 1 {
          }
          frame 2 {
          }
          frame 3 {
          }
          frame 4 {
          }
          frame 5 {
            n852 = global write "COD测量模式全局.vi" "加标回收启动时间"(w1410) -> ()
          }
          frame 6 {
          }
          frame 7 {
          }
          frame 8 {
          }
        }
        n853 = for {
          tunnel: w1400 -> [w1416] mode=indexing
          i -> [w1415]
          n854 = case shown="真" w1416 {
            tunnel: w1415 -> [_ w1417]
            frame False {
            }
            frame True {
              "测量模式数字" <- w1417
            }
          }
        }
        n855 = global write "COD测量模式全局.vi" "测量模式"(w1398) -> ()
      }
    }
    n856 = case shown="真" w1336 {
      tunnel: w1333 -> [_ w1471]
      frame False {
      }
      frame True {
        n857 = Get Date/Time In Seconds() -> (seconds since 1Jan1904=w1473:timestamp)
        n858 = Bundle By Name(cluster=T14 {"时间标识"=timestamp(0 s since 1904-01-01), "设备"="", "日志信息"=""} ("data in"), "时间标识"=w1473, "设备"="CODMn", "日志信息"=w1471) -> (w1474:T14)
        n859 = call "报警信息字段定义.vi"("table输入"="报警信息", "data in"=w1474) -> ("table输出"=w1478:string, "columns"=w1479:string[], "data out"=w1480:T14)  [unwired: 7 in]
        n860 = call "插入数据.vi"("data"=w1480, "columns"=w1479, "database"="database3.mdb", "table"=w1478) -> ()  [unwired: 7 in, 1 out]
      }
    }
    n861 = Greater?(x=w1272, y=u16 0) -> (0:w1273:bool)
    n862 = call <vilib>:"Boolean Crossing PtByPt.vi"("direction"=enum16{"either", "false-true", "true-false"}."false-true", "input"=w1273) -> ("crossing"=w1271:bool)  [unwired: 1 in]
    n863 = local read "测量数据区"() -> (w1295:T2)
    n864 = case shown="\"水样测试\"" w1293 {
      tunnel: w1295 -> [w1418 w1423 w1428 w1433 w1438 w1443 w1448 w1453]
      tunnel: [w1418 w1422 w1424 w1432 w1437 w1442 w1444 w1452] -> w1292
      tunnel: w1291 -> [_ w1421 w1427 w1431 w1436 w1441 w1447 w1451]
      tunnel: w1290 -> [_ w1420 w1426 w1430 w1435 w1440 w1446 w1450]
      tunnel: w1289 -> [_ w1419 w1425 w1429 w1434 w1439 w1445 w1449]
      frame "", Default {
      }
      frame "水样测试" {
        n865 = Bundle By Name(cluster=w1423, "水样数据时间"=w1421, "水样实测值"=w1420, "水样数据标识"=w1419) -> (w1422:T2)
      }
      frame "标样核查" {
        n866 = Bundle By Name(cluster=w1428, "跨度核查数据时间"=w1427, "跨度核查实测值"=w1426, "跨度核查数据标识"=w1425) -> (w1424:T2)
      }
      frame "零点核查" {
        n867 = Bundle By Name(cluster=w1433, "零点核查数据时间"=w1431, "零点核查实测值"=w1430, "零点核查数据标识"=w1429) -> (w1432:T2)
      }
      frame "加标回收" {
        n868 = Bundle By Name(cluster=w1438, "加标回收数据时间"=w1436, "加标回收实测值"=w1435, "加标回收数据标识"=w1434) -> (w1437:T2)
      }
      frame "平行样" {
        n869 = Bundle By Name(cluster=w1443, "平行样数据时间"=w1441, "平行样实测值"=w1440, "平行样数据标识"=w1439) -> (w1442:T2)
      }
      frame "校零" {
        n870 = Bundle By Name(cluster=w1448, "空白数据时间"=w1447, "空白实测值"=w1446, "空白数据标识"=w1445) -> (w1444:T2)
      }
      frame "校标" {
        n871 = Bundle By Name(cluster=w1453, "标样数据时间"=w1451, "标样实测值"=w1450, "标样数据标识"=w1449) -> (w1452:T2)
      }
    }
    "测量数据区" <- w1292
    n872 = case shown="真" w1271 {
      frame False {
      }
      frame True {
        n873 = Get Date/Time In Seconds() -> (seconds since 1Jan1904=→"启动时间":timestamp)
      }
    }
    n874 = Get Date/Time In Seconds() -> (seconds since 1Jan1904=w1310:timestamp)
    "系统时间" <- w1310
    n875 = call "HexToDate.vi"("数组"=w1316) -> ("DATE"=w1311:timestamp[])  [unwired: 10 in]
    n876 = Index Array(array=w1311) -> (element=→"仪器时间":timestamp)  [unwired: 1 in]
    n877 = Build Array(w1310) -> (w1309:timestamp[])
    n878 = call "DateToHex.vi"("DATE"=w1311) -> ("数组"=w1303:u16[])  [unwired: 10 in]
    n879 = call "DateToHex.vi"("DATE"=w1309) -> ("数组"=w1308:u16[])  [unwired: 10 in]
    n880 = Index Array(array=w1303, index=2 ("索引")) -> (element=w1305:u16)
    n881 = Split Number(x=w1305) -> (hi(x)=w1299:u8)  [unwired: 1 out]
    n882 = Index Array(array=w1308, index=2 ("索引")) -> (element=w1306:u16)
    n883 = Split Number(x=w1306) -> (hi(x)=w1302:u8)  [unwired: 1 out]
    n884 = To Byte Integer(number=w1299) -> (8bit integer=w1298:i8)
    n885 = To Byte Integer(number=w1302) -> (8bit integer=w1301:i8)
    n886 = Subtract(x=w1298, y=w1301) -> (x-y=w1300:i8)
    n887 = Absolute Value(x=w1300) -> (abs(x)=w1297:i8)
    n888 = Greater Or Equal?(x=w1297, y=i8 5) -> ()  [unwired: 1 out]
  }
  n889 = while {
    tunnel: w28 -> [w1489]
    stop <- FALSE stop-if-true
    n890 = event shown="[0] \"保存\": 鼠标按下" {
      selector: _ -> [_]
      dyn-events: _ -> [_]
      timeout: _ -> [_]
      tunnel: w1489 -> [w1511]
      event "保存": Mouse Down {
        (unwired) 1000 ("超时毫秒(-1)")
        (unwired) cluster{"starting address":u16, "values":u16[]} {"starting address"=4625, "values"=[]}
        n891 = event-data() -> ()  [unwired: 1 in, 8 out]
        n892 = global read "COD浓度全局变量.vi" "配置文件ini"() -> (w1492:string)
        n893 = call <vilib>:"Application Directory.vi"() -> ("Application Directory"=w1498:path)
        n894 = Build Path(base path=w1498, name or relative path=w1492) -> (appended path=w1497:path)
        n895 = local write "枚举"(enum16{"读取数据", "写入数据", "读取写入DATABASE", "读取参数"}."写入数据" ("枚举")) -> ()
        n896 = local read "跨度液浓度"() -> (w1501:dbl)
        n897 = call <vilib>:"Open Config Data.vi"("configuration file path"=w1497) -> ("error out"=w1495:errorcluster, "refnum"=w1496:T9)  [unwired: 8 in, 1 out]
        n898 = call-poly <vilib>:"Write Key.vi"("section"="CODMn参数" ("key"), "error in (no error)"=w1495, "value"=w1501, "key"="跨度液浓度", "refnum"=w1496) -> ("error out"=w1493:errorcluster, "refnum out"=w1494:T9)  [unwired: 4 in, 1 out]
        n899 = call <vilib>:"Close Config Data.vi"("error in (no error)"=w1493, "refnum"=w1494) -> ()  [unwired: 8 in, 2 out]
        n900 = local write "水样"("水样") -> ()
        n901 = local write "标液"("标液") -> ()
        n902 = local write "硫酸"("硫酸") -> ()
        n903 = local write "恒温时间"("恒温时间") -> ()
        n904 = local write "修正系数"("修正系数") -> ()
        n905 = local write "加标回收"("加标回收") -> ()
        n906 = local write "高锰酸钾"("高锰酸钾") -> ()
        n907 = local write "基本量程"("基本量程") -> ()
        n908 = local write "标样浓度 2"("标样浓度 2") -> ()
        n909 = local write "零点泵计量数 2"("零点泵计量数 2") -> ()
        n910 = local write "标度泵计量数 2"("标度泵计量数 2") -> ()
        n911 = local write "蒸馏水"("蒸馏水") -> ()
        n912 = local write "温度 2"("温度 2") -> ()
        n913 = local write "草酸钠"("草酸钠") -> ()
        n914 = local write "质控样"("质控样") -> ()
        n915 = Build Array("温度 2", "恒温时间", "浓度", "修正系数", "基本量程", "水样", "蒸馏水", "标液", "质控样", "加标回收", "高锰酸钾", "草酸钠", "硫酸", "零点泵计量数 2", "标度泵计量数 2", "标样浓度 2", "高量程稀释倍数:", "低量程稀释倍数:") -> (w1509:dbl[])
        n916 = Bundle By Name(cluster=cluster{"starting address":u16, "values":u16[]} {"starting address"=4272, "values"=[]}, "starting address"=u16 4272, "values"=w1509) -> (w1507:cluster{"starting address":u16, "values":u16[]})
        n917 = Enqueue Element(queue=w1511, element=w1507, timeout in ms (-1)=1000 ("超时毫秒(-1)")) -> ()  [unwired: 1 in, 3 out]
      }
    }
  }
  n918 = while {
    tunnel: w31 -> [w1541]
    tunnel: w30 -> [w1540]
    tunnel: w28 -> [w1539]
    tunnel: w44 -> [w1538]
    tunnel: w43 -> [w1537]
    tunnel: [w1527] -> w42
    tunnel: [w1536] -> w41
    tunnel: w17 -> [w1534]
    tunnel: w16 -> [w1533]
    tunnel: w34 -> [w1532]
    tunnel: w33 -> [w1531]
    tunnel: w32 -> [w1530]
    tunnel: w28 -> [w1525]
    stop <- FALSE stop-if-true
    n919 = case shown="\"读取参数\"" "枚举" {
      tunnel: w1541 -> [w1577 w1587 w1685 w1779]
      tunnel: w1540 -> [w1576 w1583 w1684 w1778]
      tunnel: w1539 -> [_ w1586 _ _]
      tunnel: [w1543 w1585 w1687 w1773] -> w1536
      tunnel: [w1542 w1584 w1686 w1771] -> w1527
      tunnel: w1538 -> [w1574 _ _ _]
      tunnel: w1537 -> [w1570 _ _ _]
      tunnel: w1534 -> [_ _ _ w1777]
      tunnel: w1533 -> [_ _ _ w1776]
      tunnel: w1532 -> [_ _ w1683 _]
      tunnel: w1531 -> [_ _ w1682 _]
      tunnel: w1530 -> [_ w1582 _ _]
      tunnel: w1525 -> [_ _ w1636 _]
      frame "读取数据", Default {
        n920 = Dequeue Element(queue=w1574, timeout in ms (-1)=1000 ("超时毫秒(-1)"), error in (no error)=w1570) -> (element=w1573:T4)  [unwired: 3 out]
        n921 = Unbundle By Name(w1573) -> ("starting address"=w1572:u16, "number of holding registers"=w1571:u16)
        n922 = call <vilib>:"Read Holding Registers.vi"("error in (no error)"=w1576, "quantity"=w1571, "starting address"=w1572, "MB session in"=w1577) -> ("error out"=w1565:errorcluster, "Registers"=→"Registers":u16[], "MB session out"=w1568:refnum<class "MB_Master_Serial.lvclass">)  [unwired: 5 in]
        n923 = call <vilib>:"Read Coils.vi"("error in (no error)"=w1565, "quantity"=u16 8, "starting address"=u16 140, "MB session in"=w1568) -> ("error out"=w1555:errorcluster, "Coils"=w1564:bool[], "MB session out"=w1556:refnum<class "MB_Master_Serial.lvclass">)  [unwired: 5 in]
        n924 = Index Array(array=w1564) -> (element #1=→"进水样":bool, element #2=→"进蒸馏水":bool, element #3=→"进标液":bool, element #4=→"进质控样":bool, element #5=→"进加标回收样":bool, element #6=→"进高锰酸钾":bool, element #7=→"进草酸钠":bool, element #8=→"进硫酸":bool)  [unwired: 9 in, 1 out]
        n925 = call <vilib>:"Read Coils.vi"("error in (no error)"=w1555, "quantity"=u16 1, "starting address"=u16 137, "MB session in"=w1556) -> ("error out"=w1551:errorcluster, "Coils"=w1545:bool[], "MB session out"=w1552:refnum<class "MB_Master_Serial.lvclass">)  [unwired: 5 in]
        n926 = Index Array(array=w1545) -> (element=→"搅拌":bool)  [unwired: 1 in]
        n927 = call <vilib>:"Read Coils.vi"("error in (no error)"=w1551, "quantity"=u16 1, "starting address"=u16 400, "MB session in"=w1552) -> ("error out"=w1542:errorcluster, "Coils"=w1548:bool[], "MB session out"=w1543:refnum<class "MB_Master_Serial.lvclass">)  [unwired: 5 in]
        n928 = Index Array(array=w1548) -> (element=→"加热":bool)  [unwired: 1 in]
      }
      frame "写入数据" {
        n929 = flat-sequence {
          tunnel: w1587 -> [w1598]
          tunnel: w1586 -> [w1597]
          tunnel: w1583 -> [w1591]
          tunnel: w1582 -> [w1590]
          tunnel: [w1593] -> w1581
          tunnel: [w1592] -> w1580
          tunnel: [w1589] -> w1579
          tunnel: [w1588] -> w1578
          tunnel: [w1599] -> w1584
          tunnel: [w1605] -> w1585
          tunnel: w1581 -> [w1605]
          tunnel: w1580 -> [w1599]
          tunnel: w1579 -> [w1604]
          tunnel: w1578 -> [w1603]
          frame #0 {
            n930 = Dequeue Element(queue=w1597, error in (no error)=w1590) -> (queue out=w1589:refnum<queue>, element=w1596:cluster{"starting address":u16, "values":u16[]}, error out=w1588:errorcluster)  [unwired: 1 in, 1 out]
            n931 = Unbundle By Name(w1596) -> ("starting address"=w1595:u16, "values"=w1594:u16[])
            n932 = call <vilib>:"Write Multiple Registers.vi"("error in (no error)"=w1591, "values"=w1594, "starting address"=w1595, "MB session in"=w1598) -> ("error out"=w1592:errorcluster, "MB session out"=w1593:refnum<class "MB_Master_Serial.lvclass">)  [unwired: 6 in]
          }
          frame #1 {
            n933 = Get Queue Status(queue=w1604, error in (no error)=w1603) -> (# elements in queue=w1602:i32)  [unwired: 1 in, 7 out]
            n934 = Equal To 0?(x=w1602) -> (x = 0?=w1601:bool)
            n935 = case shown="真" w1601 {
              tunnel: [enum16{"读取数据", "写入数据", "读取写入DATABASE", "读取参数"}."写入数据" ("枚举") enum16{"读取数据", "写入数据", "读取写入DATABASE", "读取参数"}."读取数据" ("枚举")] -> w1600
              tunnel: w1599 -> [_ w1607]
              frame False {
              }
              frame True {
                n936 = case shown="无错误" w1607 {
                  tunnel: ["保存成功" ("消息") "保存失败" ("消息")] -> _
                  frame No Error {
                  }
                  frame Error {
                  }
                }
              }
            }
            n937 = local write "枚举"(w1600) -> ()
          }
        }
      }
      frame "读取写入DATABASE" {
        n938 = Dequeue Element(queue=w1683, timeout in ms (-1)=1000 ("超时毫秒(-1)"), error in (no error)=w1682) -> (element=w1690:T4)  [unwired: 3 out]
        n939 = Unbundle By Name(w1690) -> ("starting address"=w1689:u16, "number of holding registers"=w1688:u16)
        n940 = call <vilib>:"Read Holding Registers.vi"("error in (no error)"=w1684, "quantity"=w1688, "starting address"=w1689, "MB session in"=w1685) -> ("error out"=w1686:errorcluster, "Registers"=w1620:u16[], "MB session out"=w1687:refnum<class "MB_Master_Serial.lvclass">)  [unwired: 5 in]
        n941 = To Word Integer(number=w1620) -> (16bit integer=w1619:i16[])
        n942 = Split 1D Array(array=w1619, index=3 ("索引")) -> (first subarray=w1680:i16[], second subarray=w1670:i16[])
        n943 = case shown="\"维护模式\", 默认" enum16{"维护模式", "常规模式", "应急模式", "质控模式"}."维护模式" ("运行模式") {
          tunnel: ["M" ("单位") "N" ("单位") "N" ("单位") "N" ("单位")] -> w1638
          frame "维护模式", Default {
          }
          frame "常规模式" {
          }
          frame "应急模式" {
          }
          frame "质控模式" {
          }
        }
        n944 = Index Array(array=w1680) -> (element #1=w1678:i16, element #2=w1677:i16, element #3=w1676:i16)  [unwired: 3 in]
        n945 = Index Array(array=w1670) -> (element #1=w1628:i16, element #2=w1674:i16, element #3=w1673:i16, element #4=w1672:i16, element #5=w1671:i16)  [unwired: 5 in]
        n946 = Index Array(array=w1670, index=6 ("索引")) -> (element=w1668:i16)
        n947 = To Single Precision Float(number=w1628) -> (single precision float=w1630:sgl)
        n948 = Divide(x=w1630, y=sgl 100.0) -> (x/y=w1629:sgl)
        n949 = Less Or Equal?(x=w1629, y=sgl 0.01) -> (x <= y?=w1632:bool)
        n950 = case shown="假" w1632 {
          tunnel: [w1762 w1763] -> w1631
          tunnel: w1629 -> [w1762 _]
          frame False {
          }
          frame True {
            n951 = Random Number (0-1)() -> (number: 0 to 1=w1766:dbl)
            n952 = Increment(x=w1766) -> (x+1=w1764:dbl)
            n953 = Divide(x=w1764, y=sgl 100.0) -> (x/y=w1763:dbl)
          }
        }
        n954 = Build Array(w1678, w1677, w1676) -> (w1675:i16[])
        n955 = To Single Precision Float(number=w1674) -> (single precision float=w1642:sgl)
        n956 = To Single Precision Float(number=w1673) -> (single precision float=w1643:sgl)
        n957 = To Single Precision Float(number=w1672) -> (single precision float=w1644:sgl)
        n958 = To Single Precision Float(number=w1671) -> (single precision float=w1665:sgl)
        n959 = call "HexToDate.vi"("数组"=w1675) -> ("DATE"=w1679:timestamp[])  [unwired: 10 in]
        n960 = Index Array(array=w1679) -> ()  [unwired: 1 in, 1 out]
        n961 = disable-structure shown="启用" {
          disable-tunnel: w1631 -> [w1692 w1716]
          disable-tunnel: [w1691 w1716] -> w1621
          frame Disabled {
            # "高量程0-5之间会乘1.2的系数\n低量程0-2之间会乘1.1的系数"
            n962 = property on="基本量程" class="Enum (严格)"() -> ("Value"=w1693:enum16{"L", "H"})  [unwired: 2 in, 2 out]
            n963 = case shown="\"L\", 默认" w1693 {
              tunnel: w1692 -> [w1696 w1706]
              tunnel: [w1694 w1705] -> w1691
              frame "L", Default {
                n964 = Less Or Equal?(x=w1696, y=2.0) -> (x <= y?=w1699:bool)
                n965 = Greater?(x=w1696, y=0.0) -> (0:w1698:bool)
                n966 = And(x=w1699, y=w1698) -> (x .and. y?=w1695:bool)
                n967 = case shown="假" w1695 {
                  tunnel: w1696 -> [w1701 w1704]
                  tunnel: [w1701 w1702] -> w1694
                  frame False {
                  }
                  frame True {
                    n968 = Multiply(x=w1704, y=1.1) -> (x*y=w1702:dbl)
                  }
                }
              }
              frame "H" {
                n969 = Greater?(x=w1706, y=0.0) -> (0:w1709:bool)
                n970 = Less Or Equal?(x=w1706, y=5.0) -> (x <= y?=w1710:bool)
                n971 = And(x=w1710, y=w1709) -> (x .and. y?=w1707:bool)
                n972 = case shown="真" w1707 {
                  tunnel: w1706 -> [w1712 w1715]
                  tunnel: [w1712 w1713] -> w1705
                  frame False {
                  }
                  frame True {
                    n973 = Multiply(x=w1715, y=1.2) -> (x*y=w1713:dbl)
                  }
                }
              }
            }
          }
          frame Enabled {
          }
        }
        "COD浓度（mg/L)" <- w1621
        n974 = To Single Precision Float(number=w1668) -> (single precision float=w1634:sgl)
        n975 = global read "COD测量模式全局.vi" "测量模式"() -> (w1618:string)
        n976 = global read "COD测量模式全局.vi" "测量模式"() -> (w1635:string)
        n977 = global read "COD测量模式全局.vi" "测量模式"() -> (w1627:string)
        n978 = local read "启动时间"() -> (w1616:timestamp)
        n979 = Divide(x=w1665, y=sgl 1000.0) -> (x/y=w1645:sgl)
        n980 = Format Into String(format string="w%05d" ("格式字符串"), u32 1019 ("因子编码")) -> (resulting string=w1641:string)  [unwired: 2 in, 1 out]
        n981 = case shown="\"\", 默认" w1618 {
          tunnel: [0.0 w1718 w1721] -> w1617
          frame "", Default {
          }
          frame "标样核查", "校标" {
            n982 = local read "标样浓度 2"() -> (w1719:dbl)
            n983 = Divide(x=w1719, y=100.0) -> (x/y=w1718:dbl)
          }
          frame "跨度核查" {
            n984 = local read "跨度液浓度"() -> (w1721:dbl)
          }
        }
        n985 = Not Equal?(x=w1627, y="校标") -> (x != y?=w1625:bool)
        n986 = case shown="真" w1625 {
          tunnel: w1636 -> [_ w1732]
          tunnel: w1621 -> [_ w1730]
          frame False {
            n987 = local write "枚举"(enum16{"读取数据", "写入数据", "读取写入DATABASE", "读取参数"}."读取数据" ("枚举")) -> ()
          }
          frame True {
            n988 = case shown="真" "自动切换量程" {
              tunnel: w1732 -> [_ w1734]
              tunnel: w1730 -> [_ w1735]
              frame False {
                n989 = local write "枚举"(enum16{"读取数据", "写入数据", "读取写入DATABASE", "读取参数"}."读取数据" ("枚举")) -> ()
              }
              frame True {
                n990 = local read "基本量程"() -> (w1736:enum16{"L", "H"})
                n991 = case shown="\"L\", 默认" w1736 {
                  tunnel: w1735 -> [w1740 w1751]
                  tunnel: w1734 -> [w1737 w1749]
                  frame "L", Default {
                    n992 = Greater?(x=w1740, y="低切高阈值") -> (0:w1738:bool)
                    n993 = case shown="真" w1738 {
                      tunnel: w1737 -> [_ w1742]
                      frame False {
                        n994 = local write "枚举"(enum16{"读取数据", "写入数据", "读取写入DATABASE", "读取参数"}."读取数据" ("枚举")) -> ()
                      }
                      frame True {
                        n995 = local write "枚举"(enum16{"读取数据", "写入数据", "读取写入DATABASE", "读取参数"}."写入数据" ("枚举")) -> ()
                        n996 = Bundle By Name(cluster=cluster{"starting address":u16, "values":u16[]} {"starting address"=0, "values"=[]}, "starting address"=u16 4276, "values"=u16[] [1]) -> (w1746:cluster{"starting address":u16, "values":u16[]})
                        n997 = Enqueue Element(queue=w1742, element=w1746) -> ()  [unwired: 2 in, 3 out]
                      }
                    }
                  }
                  frame "H" {
                    n998 = Less?(x=w1751, y="高切低阈值") -> (x < y?=w1748:bool)
                    n999 = case shown="真" w1748 {
                      tunnel: w1749 -> [_ w1754]
                      frame False {
                        n1000 = local write "枚举"(enum16{"读取数据", "写入数据", "读取写入DATABASE", "读取参数"}."读取数据" ("枚举")) -> ()
                      }
                      frame True {
                        n1001 = local write "枚举"(enum16{"读取数据", "写入数据", "读取写入DATABASE", "读取参数"}."写入数据" ("枚举")) -> ()
                        n1002 = Bundle By Name(cluster=cluster{"starting address":u16, "values":u16[]} {"starting address"=0, "values"=[]}, "starting address"=u16 4276, "values"=u16[] [0]) -> (w1756:cluster{"starting address":u16, "values":u16[]})
                        n1003 = Enqueue Element(queue=w1754, element=w1756) -> ()  [unwired: 2 in, 3 out]
                      }
                    }
                  }
                }
              }
            }
          }
        }
        n1004 = local read "温度"() -> (w1637:dbl)
        n1005 = global read "COD浓度全局变量.vi" "序列号:"() -> (w1611:string)
        n1006 = global read "COD测量模式全局.vi" "测量模式"() -> (w1624:string)
        n1007 = Bundle(cluster=T17 {"时间"=timestamp(0 s since 1904-01-01), "测量模式"="", "数据类型"="", "检测值"=0.0, "单位"="", "数据标识"="", "因子编码"="", "标样参考值"=0.0, "ORP-A"=0.0, "ORP-B"=0.0, "ORP-K"=0.0, "COD滴定值"=0.0, "高锰酸钾滴定数"=0.0, "温度"=0.0, "序列号"=""} ("data"), "时间"=w1616, "测量模式"=w1635, "数据类型"=w1638, "检测值"=w1621, "单位"="mg/L", "数据标识"="N", "因子编码"=w1641, "标样参考值"=w1617, "ORP-A"=w1642, "ORP-B"=w1643, "ORP-K"=w1644, "COD滴定值"=w1645, "高锰酸钾滴定数"=w1634, "温度"=w1637, "序列号"=w1611) -> (w1612:T17)
        n1008 = Build Array("时间", "测量模式", "数据类型", "检测值", "单位", "数据标识", "因子编码", "标样参考值", "ORPA", "ORPB", "ORPK", "COD滴定值", "高锰酸钾滴定数", "温度", "序列号" ("元素")) -> (w1652:string[])
        n1009 = Equal?(x=w1624, y="校标") -> (x = y?=w1622:bool)
        n1010 = global write "COD浓度全局变量.vi" "COD浓度（mg/L)"(w1621) -> ()
        n1011 = global write "COD读取DATA全局.vi" "data"(w1612) -> ()
        n1012 = flat-sequence {
          tunnel: "CODMn" ("table") -> [w1761]
          tunnel: w1652 -> [w1760]
          tunnel: w1612 -> [w1759]
          frame #0 {
            n1013 = call "数据写入database.vi"("data"=w1759, "columns"=w1760, "table"=w1761) -> ()  [unwired: 8 in, 1 out]
          }
        }
        n1014 = case shown="真" w1622 {
          tunnel: w1634 -> [_ w1722]
          frame False {
          }
          frame True {
            n1015 = local read "当前校准"() -> (w1723:i32)
            n1016 = case shown="3" w1723 {
              tunnel: w1722 -> [w1724 w1725 w1726 w1727 w1728]
              frame 1, Default {
                n1017 = local write "泵滴定数1"(w1724) -> ()
              }
              frame 2 {
                n1018 = local write "泵滴定数2"(w1725) -> ()
              }
              frame 3 {
                n1019 = local write "泵滴定数3"(w1726) -> ()
              }
              frame 4 {
                n1020 = local write "泵滴定数4"(w1727) -> ()
              }
              frame 5 {
                n1021 = local write "泵滴定数5"(w1728) -> ()
              }
            }
          }
        }
      }
      frame "读取参数" {
        n1022 = Dequeue Element(queue=w1777, timeout in ms (-1)=1000 ("超时毫秒(-1)"), error in (no error)=w1776) -> (element=w1783:T4)  [unwired: 3 out]
        n1023 = local write "枚举"(enum16{"读取数据", "写入数据", "读取写入DATABASE", "读取参数"}."读取数据" ("枚举")) -> ()
        n1024 = Unbundle By Name(w1783) -> ("starting address"=w1782:u16, "number of holding registers"=w1781:u16)
        n1025 = local read "读取KB值"() -> (w1772:bool)
        n1026 = call <vilib>:"Read Holding Registers.vi"("error in (no error)"=w1778, "quantity"=w1781, "starting address"=w1782, "MB session in"=w1779) -> ("error out"=w1771:errorcluster, "Registers"=w1775:u16[], "MB session out"=w1773:refnum<class "MB_Master_Serial.lvclass">)  [unwired: 5 in]
        n1027 = case shown="真" w1772 {
          tunnel: w1775 -> [w1795 w1816]
          tunnel: w1771 -> [_ w1818]
          frame False {
            n1028 = Index Array(array=w1795) -> (element #1=w1789:u16, element #2=w1808:u16, element #3=w1807:u16, element #4=w1787:u16, element #5=w1806:u16, element #6=w1805:u16, element #7=w1804:u16, element #8=w1803:u16, element #9=w1802:u16, element #10=w1801:u16, element #11=w1800:u16, element #12=w1799:u16, element #13=w1798:u16, element #14=w1797:u16, element #15=w1796:u16, element #16=w1794:u16, element #17=w1785:u16, element #18=w1784:u16)  [unwired: 18 in]
            n1029 = local write "浓度"(w1807) -> ()
            n1030 = local write "水样"(w1805) -> ()
            n1031 = local write "硫酸"(w1798) -> ()
            n1032 = local write "标液"(w1803) -> ()
            n1033 = local write "高量程稀释倍数:"(w1785) -> ()
            n1034 = local write "低量程稀释倍数:"(w1784) -> ()
            n1035 = Divide(x=w1789, y=u16 10) -> (x/y=w1790:dbl)
            n1036 = local write "草酸钠"(w1799) -> ()
            n1037 = local write "蒸馏水"(w1804) -> ()
            n1038 = local write "质控样"(w1802) -> ()
            n1039 = local write "恒温时间"(w1808) -> ()
            n1040 = local write "基本量程"(w1806) -> ()
            n1041 = local write "加标回收"(w1801) -> ()
            n1042 = local write "高锰酸钾"(w1800) -> ()
            n1043 = local write "零点泵计量数 2"(w1797) -> ()
            n1044 = local write "标度泵计量数 2"(w1796) -> ()
            n1045 = Divide(x=w1787, y=u16 100) -> (x/y=w1786:dbl)
            n1046 = Divide(x=w1794, y=u16 100) -> (x/y=w1793:dbl)
            n1047 = local write "温度"(w1790) -> ()
            n1048 = local write "修正系数 2"(w1786) -> ()
            n1049 = local write "浓度 2"(w1793) -> ()
          }
          frame True {
            (unwired) 9 ("索引")
            n1050 = case shown="错误" w1818 {
              tunnel: ["读取成功" ("消息") "读取失败" ("消息")] -> w1817
              frame No Error {
              }
              frame Error {
              }
            }
            n1051 = Array Subset(array=w1816, index=10 ("索引"), length=84 ("长度")) -> (w1813:u16[])
            n1052 = call "浮点CDAB转换COD.vi"("数组"=w1813) -> ("数组 2"=w1812:sgl[])  [unwired: 10 in]
            n1053 = One Button Dialog(message=w1817) -> ()  [unwired: 1 in, 1 out]
            n1054 = Array To Cluster(array=w1812) -> (cluster=w1810:T18)
            n1055 = local read "测量模式(公式)"() -> (w1811:u16)
            n1056 = case shown="7" w1811 {
              tunnel: [cluster{"X":dbl, "b":dbl, "X^2":dbl} {"X"=999.0, "b"=999.0, "X^2"=999.0} ("方程系数") w1822 w1841 w1860 w1879 w1898 w1917 w1936] -> w1809
              tunnel: w1810 -> [_ w1821 w1840 w1859 w1878 w1897 w1916 w1935]
              frame 0, Default {
              }
              frame 1 {
                n1057 = local read "量程选择"() -> (w1820:enum16{"低量程", "高量程", "0-2量程"})
                n1058 = case shown="\"低量程\", 默认" w1820 {
                  tunnel: w1821 -> [w1830 w1834 w1838]
                  tunnel: [w1829 w1833 w1837] -> w1826
                  tunnel: [w1828 w1832 w1836] -> w1825
                  tunnel: [w1827 w1831 w1835] -> w1824
                  frame "低量程", Default {
                    n1059 = Unbundle By Name(w1830) -> ("数组 2[0]"=w1829:sgl, "数组 2[1]"=w1828:sgl, "数组 2[2]"=w1827:sgl)
                  }
                  frame "高量程" {
                    n1060 = Unbundle By Name(w1834) -> ("数组 2[3]"=w1833:sgl, "数组 2[4]"=w1832:sgl, "数组 2[5]"=w1831:sgl)
                  }
                  frame "0-2量程" {
                    n1061 = Unbundle By Name(w1838) -> ("数组 2[6]"=w1837:sgl, "数组 2[7]"=w1836:sgl, "数组 2[8]"=w1835:sgl)
                  }
                }
                n1062 = Bundle By Name(cluster=cluster{"X":dbl, "b":dbl, "X^2":dbl} {"X"=0.0, "b"=0.0, "X^2"=0.0} ("方程系数"), "X"=w1826, "b"=w1825, "X^2"=w1824) -> (w1822:cluster{"X":dbl, "b":dbl, "X^2":dbl})
              }
              frame 2 {
                n1063 = local read "量程选择"() -> (w1839:enum16{"低量程", "高量程", "0-2量程"})
                n1064 = case shown="\"高量程\"" w1839 {
                  tunnel: w1840 -> [w1849 w1853 w1857]
                  tunnel: [w1848 w1852 w1856] -> w1845
                  tunnel: [w1847 w1851 w1855] -> w1844
                  tunnel: [w1846 w1850 w1854] -> w1843
                  frame "低量程", Default {
                    n1065 = Unbundle By Name(w1849) -> ("数组 2[6]"=w1848:sgl, "数组 2[7]"=w1847:sgl, "数组 2[8]"=w1846:sgl)
                  }
                  frame "高量程" {
                    n1066 = Unbundle By Name(w1853) -> ("数组 2[9]"=w1852:sgl, "数组 2[10]"=w1851:sgl, "数组 2[11]"=w1850:sgl)
                  }
                  frame "0-2量程" {
                    n1067 = Unbundle By Name(w1857) -> ("数组 2[6]"=w1856:sgl, "数组 2[7]"=w1855:sgl, "数组 2[8]"=w1854:sgl)
                  }
                }
                n1068 = Bundle By Name(cluster=cluster{"X":dbl, "b":dbl, "X^2":dbl} {"X"=0.0, "b"=0.0, "X^2"=0.0} ("方程系数"), "X"=w1845, "b"=w1844, "X^2"=w1843) -> (w1841:cluster{"X":dbl, "b":dbl, "X^2":dbl})
              }
              frame 3 {
                n1069 = local read "量程选择"() -> (w1858:enum16{"低量程", "高量程", "0-2量程"})
                n1070 = case shown="\"高量程\"" w1858 {
                  tunnel: w1859 -> [w1868 w1872 w1876]
                  tunnel: [w1867 w1871 w1875] -> w1864
                  tunnel: [w1866 w1870 w1874] -> w1863
                  tunnel: [w1865 w1869 w1873] -> w1862
                  frame "低量程", Default {
                    n1071 = Unbundle By Name(w1868) -> ("数组 2[12]"=w1867:sgl, "数组 2[13]"=w1866:sgl, "数组 2[14]"=w1865:sgl)
                  }
                  frame "高量程" {
                    n1072 = Unbundle By Name(w1872) -> ("数组 2[15]"=w1871:sgl, "数组 2[16]"=w1870:sgl, "数组 2[17]"=w1869:sgl)
                  }
                  frame "0-2量程" {
                    n1073 = Unbundle By Name(w1876) -> ("数组 2[6]"=w1875:sgl, "数组 2[7]"=w1874:sgl, "数组 2[8]"=w1873:sgl)
                  }
                }
                n1074 = Bundle By Name(cluster=cluster{"X":dbl, "b":dbl, "X^2":dbl} {"X"=0.0, "b"=0.0, "X^2"=0.0} ("方程系数"), "X"=w1864, "b"=w1863, "X^2"=w1862) -> (w1860:cluster{"X":dbl, "b":dbl, "X^2":dbl})
              }
              frame 4 {
                n1075 = local read "量程选择"() -> (w1877:enum16{"低量程", "高量程", "0-2量程"})
                n1076 = case shown="\"高量程\"" w1877 {
                  tunnel: w1878 -> [w1887 w1891 w1895]
                  tunnel: [w1886 w1890 w1894] -> w1883
                  tunnel: [w1885 w1889 w1893] -> w1882
                  tunnel: [w1884 w1888 w1892] -> w1881
                  frame "低量程", Default {
                    n1077 = Unbundle By Name(w1887) -> ("数组 2[18]"=w1886:sgl, "数组 2[19]"=w1885:sgl, "数组 2[20]"=w1884:sgl)
                  }
                  frame "高量程" {
                    n1078 = Unbundle By Name(w1891) -> ("数组 2[21]"=w1890:sgl, "数组 2[22]"=w1889:sgl, "数组 2[23]"=w1888:sgl)
                  }
                  frame "0-2量程" {
                    n1079 = Unbundle By Name(w1895) -> ("数组 2[6]"=w1894:sgl, "数组 2[7]"=w1893:sgl, "数组 2[8]"=w1892:sgl)
                  }
                }
                n1080 = Bundle By Name(cluster=cluster{"X":dbl, "b":dbl, "X^2":dbl} {"X"=0.0, "b"=0.0, "X^2"=0.0} ("方程系数"), "X"=w1883, "b"=w1882, "X^2"=w1881) -> (w1879:cluster{"X":dbl, "b":dbl, "X^2":dbl})
              }
              frame 5 {
                n1081 = local read "量程选择"() -> (w1896:enum16{"低量程", "高量程", "0-2量程"})
                n1082 = case shown="\"高量程\"" w1896 {
                  tunnel: w1897 -> [w1906 w1910 w1914]
                  tunnel: [w1905 w1909 w1913] -> w1902
                  tunnel: [w1904 w1908 w1912] -> w1901
                  tunnel: [w1903 w1907 w1911] -> w1900
                  frame "低量程", Default {
                    n1083 = Unbundle By Name(w1906) -> ("数组 2[24]"=w1905:sgl, "数组 2[25]"=w1904:sgl, "数组 2[26]"=w1903:sgl)
                  }
                  frame "高量程" {
                    n1084 = Unbundle By Name(w1910) -> ("数组 2[27]"=w1909:sgl, "数组 2[28]"=w1908:sgl, "数组 2[29]"=w1907:sgl)
                  }
                  frame "0-2量程" {
                    n1085 = Unbundle By Name(w1914) -> ("数组 2[6]"=w1913:sgl, "数组 2[7]"=w1912:sgl, "数组 2[8]"=w1911:sgl)
                  }
                }
                n1086 = Bundle By Name(cluster=cluster{"X":dbl, "b":dbl, "X^2":dbl} {"X"=0.0, "b"=0.0, "X^2"=0.0} ("方程系数"), "X"=w1902, "b"=w1901, "X^2"=w1900) -> (w1898:cluster{"X":dbl, "b":dbl, "X^2":dbl})
              }
              frame 6 {
                n1087 = local read "量程选择"() -> (w1915:enum16{"低量程", "高量程", "0-2量程"})
                n1088 = case shown="\"高量程\"" w1915 {
                  tunnel: w1916 -> [w1925 w1929 w1933]
                  tunnel: [w1924 w1928 w1932] -> w1921
                  tunnel: [w1923 w1927 w1931] -> w1920
                  tunnel: [w1922 w1926 w1930] -> w1919
                  frame "低量程", Default {
                    n1089 = Unbundle By Name(w1925) -> ("数组 2[30]"=w1924:sgl, "数组 2[31]"=w1923:sgl, "数组 2[32]"=w1922:sgl)
                  }
                  frame "高量程" {
                    n1090 = Unbundle By Name(w1929) -> ("数组 2[33]"=w1928:sgl, "数组 2[34]"=w1927:sgl, "数组 2[35]"=w1926:sgl)
                  }
                  frame "0-2量程" {
                    n1091 = Unbundle By Name(w1933) -> ("数组 2[6]"=w1932:sgl, "数组 2[7]"=w1931:sgl, "数组 2[8]"=w1930:sgl)
                  }
                }
                n1092 = Bundle By Name(cluster=cluster{"X":dbl, "b":dbl, "X^2":dbl} {"X"=0.0, "b"=0.0, "X^2"=0.0} ("方程系数"), "X"=w1921, "b"=w1920, "X^2"=w1919) -> (w1917:cluster{"X":dbl, "b":dbl, "X^2":dbl})
              }
              frame 7 {
                n1093 = local read "量程选择"() -> (w1934:enum16{"低量程", "高量程", "0-2量程"})
                n1094 = case shown="\"高量程\"" w1934 {
                  tunnel: w1935 -> [w1944 w1948 w1952]
                  tunnel: [w1943 w1947 w1951] -> w1940
                  tunnel: [w1942 w1946 w1950] -> w1939
                  tunnel: [w1941 w1945 w1949] -> w1938
                  frame "低量程", Default {
                    n1095 = Unbundle By Name(w1944) -> ("数组 2[36]"=w1943:sgl, "数组 2[37]"=w1942:sgl, "数组 2[38]"=w1941:sgl)
                  }
                  frame "高量程" {
                    n1096 = Unbundle By Name(w1948) -> ("数组 2[39]"=w1947:sgl, "数组 2[40]"=w1946:sgl, "数组 2[41]"=w1945:sgl)
                  }
                  frame "0-2量程" {
                    n1097 = Unbundle By Name(w1952) -> ("数组 2[6]"=w1951:sgl, "数组 2[7]"=w1950:sgl, "数组 2[8]"=w1949:sgl)
                  }
                }
                n1098 = Bundle By Name(cluster=cluster{"X":dbl, "b":dbl, "X^2":dbl} {"X"=0.0, "b"=0.0, "X^2"=0.0} ("方程系数"), "X"=w1940, "b"=w1939, "X^2"=w1938) -> (w1936:cluster{"X":dbl, "b":dbl, "X^2":dbl})
              }
            }
            n1099 = local write "方程系数"(w1809) -> ()
          }
        }
      }
    }
    n1100 = Unbundle By Name(w1527) -> ("status"=w1528:bool)
    n1101 = Not(x=w1528) -> (.not. x?=→"通讯状态":bool)
  }
  n1102 = call-dynamic "Close Session.vi"("error in (no error)"=w42, "MB_Serial session"=w41) -> ()  [unwired: 9 in, 1 out]
